vi "BRig_RT_start_v1,12__PortC.vi"() -> ()   [LabVIEW 2014]
uses:
  myRIO_BRig_RT__Case_Exp_stateList.ctl
  myRIO_BRig_RT__Case_NonExp_stateList.ctl
  <vilib>/WebDAVClient/Advanced/SessionHandle.ctl
  <vilib>/Platform/TimedLoop/XDataNode/timing_clust.ctl
  <vilib>/Platform/TimedLoop/XDataNode/nitl_modes.ctl
  <vilib>/Platform/TimedLoop/XDataNode/wakeup.ctl
  <vilib>/myRIO/Common/Instrument Driver Framework/myRIO v1.0/UART/vis/myRIO v1.0 Close UART.vi
  <vilib>/FPGAPlugInAG/myRIO-1900/niLvFpga_Open_myRIO-1900.vi
  <vilib>/rvi/interface/common/dynamic/niFpgaDynamicAddResources.vi
  <vilib>/Utility/error.llb/Error Cluster From Error Code.vi
  <vilib>/rvi/errors/niLvFpgaAdjustHostInterfaceError.vi
  <vilib>/Utility/file.llb/Read From Spreadsheet File (I64).vi
  <vilib>/Utility/file.llb/Write To Spreadsheet File (DBL).vi
  <vilib>/FPGAPlugInAG/Dynamic/niLvFpga_Close_Dynamic.vi
  <vilib>/myRIO/Common/Instrument Driver Framework/Utilities/vis/FPGA Ref Manager.vi
  <vilib>/myRIO/Common/Instrument Driver Framework/myRIO v1.0/myRIO v1.0 Reset FPGA.vi
  <vilib>/myRIO/Common/Instrument Driver Framework/myRIO v1.0/IRQ/vis/myRIO v1.0 IRQ Info FGV.vi
  <vilib>/myRIO/Common/Instrument Driver Framework/myRIO v1.0/IRQ/vis/myRIO v1.0 Timer IRQ Info FGV.vi
  <vilib>/myRIO/Common/Instrument Driver Framework/myRIO v1.0/IRQ/vis/myRIO v1.0 ISR Agent.vi
  <vilib>/rvi/interface/nirviOpenFPGA/nirviOpenFPGA.xnode
  BRig_FPGA_v3,93__PortC__build.lvbitx
  BRig_FPGA_v3,93__PortC.vi
  <vilib>/rvi/interface/nirviReadWriteControl/nirviReadWriteControl.xnode
  <vilib>/Platform/TimedLoop/XDataNode/XDataNode.xnode
  <vilib>/rvi/interface/nirviCloseFPGA/nirviCloseFPGA.xnode
  <vilib>/Platform/TimedLoop/XDataNode/XDNodeRunTimeDep.lvlib
  <vilib>/rvi/interface/Simulation/niFpgaSimulationCallBeginRW.vi
  <vilib>/myRIO/Instrument Drivers/Utilities/Utilities.lvlib
  NiFpgaLv.dll
  <vilib>/WebDAVClient/NI_WebDAV.lvlib
panel:
  out "Solenoid R":bool
  out "Solenoid L":bool
  out "Laser2":bool
  out "Laser1":bool
  out "FreeReward_c_R":u16
  out "FreeReward_c_L":u16
  in  "Laser2_LED":bool
  in  "Laser1_LED":bool
  in  "lick_Rising(F)_or_Falling(T)":bool
  out "T_ExpRun_min":dbl
  out "stop_TimedLoop":bool
  out "BTPR_avg_R":dbl
  out "T2R_avg_R":dbl
  out "BTPR_avg_L":dbl
  out "T2R_avg_L":dbl
  out "BTPR_block":u16
  out "T2R_block":u16
  in  "comm_WebDAV_connect":bool
  in  "I_sendData":bool
  in  "comm_TCP_connect":bool
  out "nRewards_total":u16 caption="# Rewards in Current Block"
  out "BUR_target":u16 caption="Target Trials Per Block"
  in  "input_Threshold_reset":bool
  out "nTrial":u16
  out "allReward_R":bool
  out "allReward_L":bool
  out "Threshold":bool
  out "tLoop":dbl format="%#_2g"
  out "L_Power_l2":dbl
  out "comm_TCP":bool
  in  "get_countPerMS":bool
  out "SolenoidReward":bool
  out "L_Power_l1":dbl caption="LaserPower"
  in  "Recording":bool
  out "FPGA_count2ms":dbl=159.0
  out "error out":errorcluster
  out "cSpout":enum16{"Left", "Right"}(ring) caption="Left or Right Spout"
  out "A4":u32 caption="LickCounter_Right"
  out "A2":u32 caption="LickCounter_Left"
  out "nRewards_Right":u16 caption="# Rewards Total (Right)"
  out "nRewards_Left":u16 caption="# Rewards Total (Left)"
  out "nRewards_cur":u16 caption="# Rewards in Current Block"
  out "TpB_target":u16 caption="Target Trials Per Block"
  out "cState_NonExp":T1 caption="WarmUp State"
  out "iBlock":u16 caption="Current Block"
  out "cState":T2 caption="Experimental State"
  out "iTrial":u16 caption="Current Trial"
  in  "Data Set Prefix":string="Exp1_TM2"
  out "comm_WebDAV":bool
  in  "Host Password":string="sabalab"
  in  "Host UserName":string="Test2"
  in  "STOP_abort":bool caption="Stop LabView\n(Stops myRio and FPGA)"
  in  "STOP_endBlock":bool caption="Stop Experiment\n@ End of Block"
  in  "STOP_endTrial":bool caption="Stop Experiment\n@ End of Trial"
  in  "START":bool caption="Start Experiment"
  # "Experimental Run"
  # "Recording Rig"
  # "FPGA Conversion\n[counts per ms]"
  # "RealTime Cycle\nShould be <5ms"
  # "STOP experiment at"
  # "Exp Run Time"
  # "Reset"
  # "min"
  # "Communication with Host"
  # "Lick Counter"
  # "Give Water?\n(Reward)"
  # "Experimental State"
  # "Left/Right"
  # "Left           Right"
  # "Direction\n(NonSpecific Licking)"
  # "Block Target"
  # "# Blocks"
  # "L          R"
  # "# Trials"
  # "# Rewards"
  # "Bad Trials\nPost Reward"
  # "Trials 2 Reward"
  # "Block"
  # "# Trials"
  # "# Rewards"
  # "Current\nBlock"
  # "WarmUp State"
  # "avg L"
  # "Total"
  # "# Rewards"
  # "# Trials"
  # "avg R"
  # "Laser Power [V]"
  # "Left           Right"
  # "FreeRewards"
  # "Laser1"
  # "Laser2"
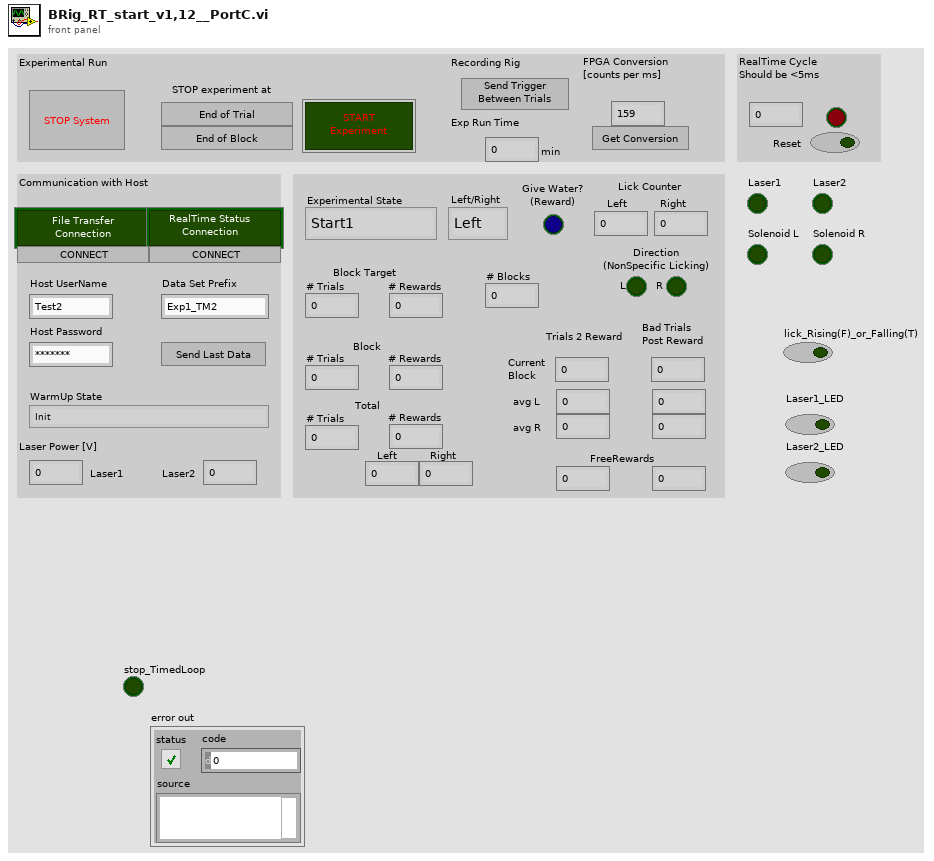
[diagram p1: front panel]
types:
  T1 = typedef "myRIO_BRig_RT__Case_NonExp_stateList.ctl" = enum16{"Init", "UploadSettings_pre", "UploadSettings_Read_dataExp", "UploadSettings_dataExp_1", "UploadSettings_dataExp_2", "UploadSettings_Read_dataLC", "UploadSettings_dataLC_1", "UploadSettings_dataLC_2", "UploadSettings_dataLC_3", "UploadSettings_dataLC_4", "UploadSettings_Read_dataMTrig", "UploadSettings_dataMTrig_1", "UploadSettings_post", "Idle_pre", "IdleEmpty", "IdleEmpty2", "IdleEmpty3", "IdleEmpty4", "Idle", "Idle_2", "Idle_3", "Idle_4", "Idle_5", "Idle_6", "Idle_post", "Cue_pre__pre", "Cue_pre", "Cue", "Cue_LED", "Cue_post", "RewardCalibration_pre", "RewardCalibration", "DispenseWater_pre__pre", "DispenseWater_pre", "DispenseWater", "DispenseWater_post", "TestConnection", "SendData", "Get_FPGA_count_per_ms", "End", "commTCP_connect"}
  T2 = typedef "myRIO_BRig_RT__Case_Exp_stateList.ctl" = enum16{"Start1", "Start2", "Start3", "saveSettings1", "saveSettings2", "saveSettings3", "saveSettings4", "saveSettings_LC_ENL_l1", "saveSettings_LC_ENL_l2", "saveSettings_LC_Cue_l1", "saveSettings_LC_Cue_l2", "saveSettings6_LC_l1_Other", "SaveSettings6_LC_l2_Other", "setSettings_Audio", "setSettings_Laser", "initBlock_pre", "initBlock", "initBlock2", "initBlock_post", "initTrial_pre", "initTrial", "initTrial2", "initTrial3", "initTrial4", "initTrial_LC_ENL1", "initTrial_LC_Cue1", "initTrial_LC_Cue1_2", "initTrial_LC_Sel", "initTrial_post", "ENL1_pre", "ENL1", "ENL1_post", "ENL1Penalty_pre", "ENL1Penalty", "ENL2_pre", "ENL2", "ENL2Penalty_pre", "ENL2Penalty", "Cue1_pre", "Cue1", "Cue1_post", "Cue1Penalty_pre", "Cue1Penalty", "Cue2_pre", "Cue2", "Cue2Penalty_pre", "Cue2Penalty", "Selection_pre", "Selection", "Select_post", "SelectReward_pre", "SelectReward", "SelectRewardPost_pre", "SelectRewardPost", "SelectWrong_pre", "SelectWrong", "SelectWrong_post", "SelectTimeout_pre", "SelectTimeout", "SelectTimeout_post", "endTrial_pre", "endTrial1", "endTrial2", "endTrial3", "endTrial_post", "endBlock_pre", "endBlock", "endBlock_post", "endExp", "commConnect", "commUpload_pre", "commUpload_dataBlock", "commUpload_dataCurrent", "commUpload_dataExp", "commUpload_dataLC", "commUpload_dataTrial", "commUpload_post", "saveData_pre", "saveData_dataBlock", "saveData_dataCurrent", "saveData_dataExp", "saveData_dataLC", "saveData_dataTrial", "saveData_post", "empty_endBlock1", "empty_endBlock2", "empty_endTrial1", "empty_endTrial2", "empty_endTrial3", "empty_endTrial4", "empty_endTrial5", "dummyState", "dummyState_endBlock", "FreeReward_pre", "FreeReward", "FreeRewardPost_pre", "FreeRewardPost"}
  T3 = enum8{"Enabled", "Disabled", "Disabled and Grayed Out"}
  T4 = typedef "NI_WebDAV.lvlib/SessionHandle.ctl" = refnum<k1>
  T5 = typedef "XDNodeRunTimeDep.lvlib/timing_clust.ctl" = cluster{"Expected End [f-1]":u64, "Actual End [f-1]":u64, "Finished Late? [f-1]":bool, "Expected End [i-1]":u64, "Actual End [i-1]":u64, "Finished Late? [i-1]":bool, "Expected Start [i]":u64, "Actual Start [i]":u64, "Expected Start [f]":u64, "Actual Start [f]":u64, "Source Name":string, "Structure Name":string, "Period":i64, "Deadline":i64, "Offset":i64, "Start":i64, "Priority":i32, "Timeout":i32, "Mode":T6, "Wakeup Reason":T7, "Error":errorcluster, "Source Type":string, "Secondary Source Type":string, "Global End Time":u64, "Global Start Time":u64, "Frame Duration":u64, "Iteration Duration":u64, "Assigned CPU":i32, "I/O Scan Engine Mode":u32}
  T6 = typedef "XDNodeRunTimeDep.lvlib/nitl_modes.ctl" = enum32{"No Change", "Process missed periods, maintain original phase", "Discard missed periods, maintain original phase", "Process missed periods, ignore original phase", "Discard missed periods, ignore original phase"}
  T7 = typedef "XDNodeRunTimeDep.lvlib/wakeup.ctl" = enum32{"Normal", "Aborted", "Asynchronous wakeup", "Timing source error", "Timed loop error", "Timeout"}
  T8 = cluster{"read mode":enum16{"polling", "blocking"}, "write mode":enum16{"polling", "blocking"}}
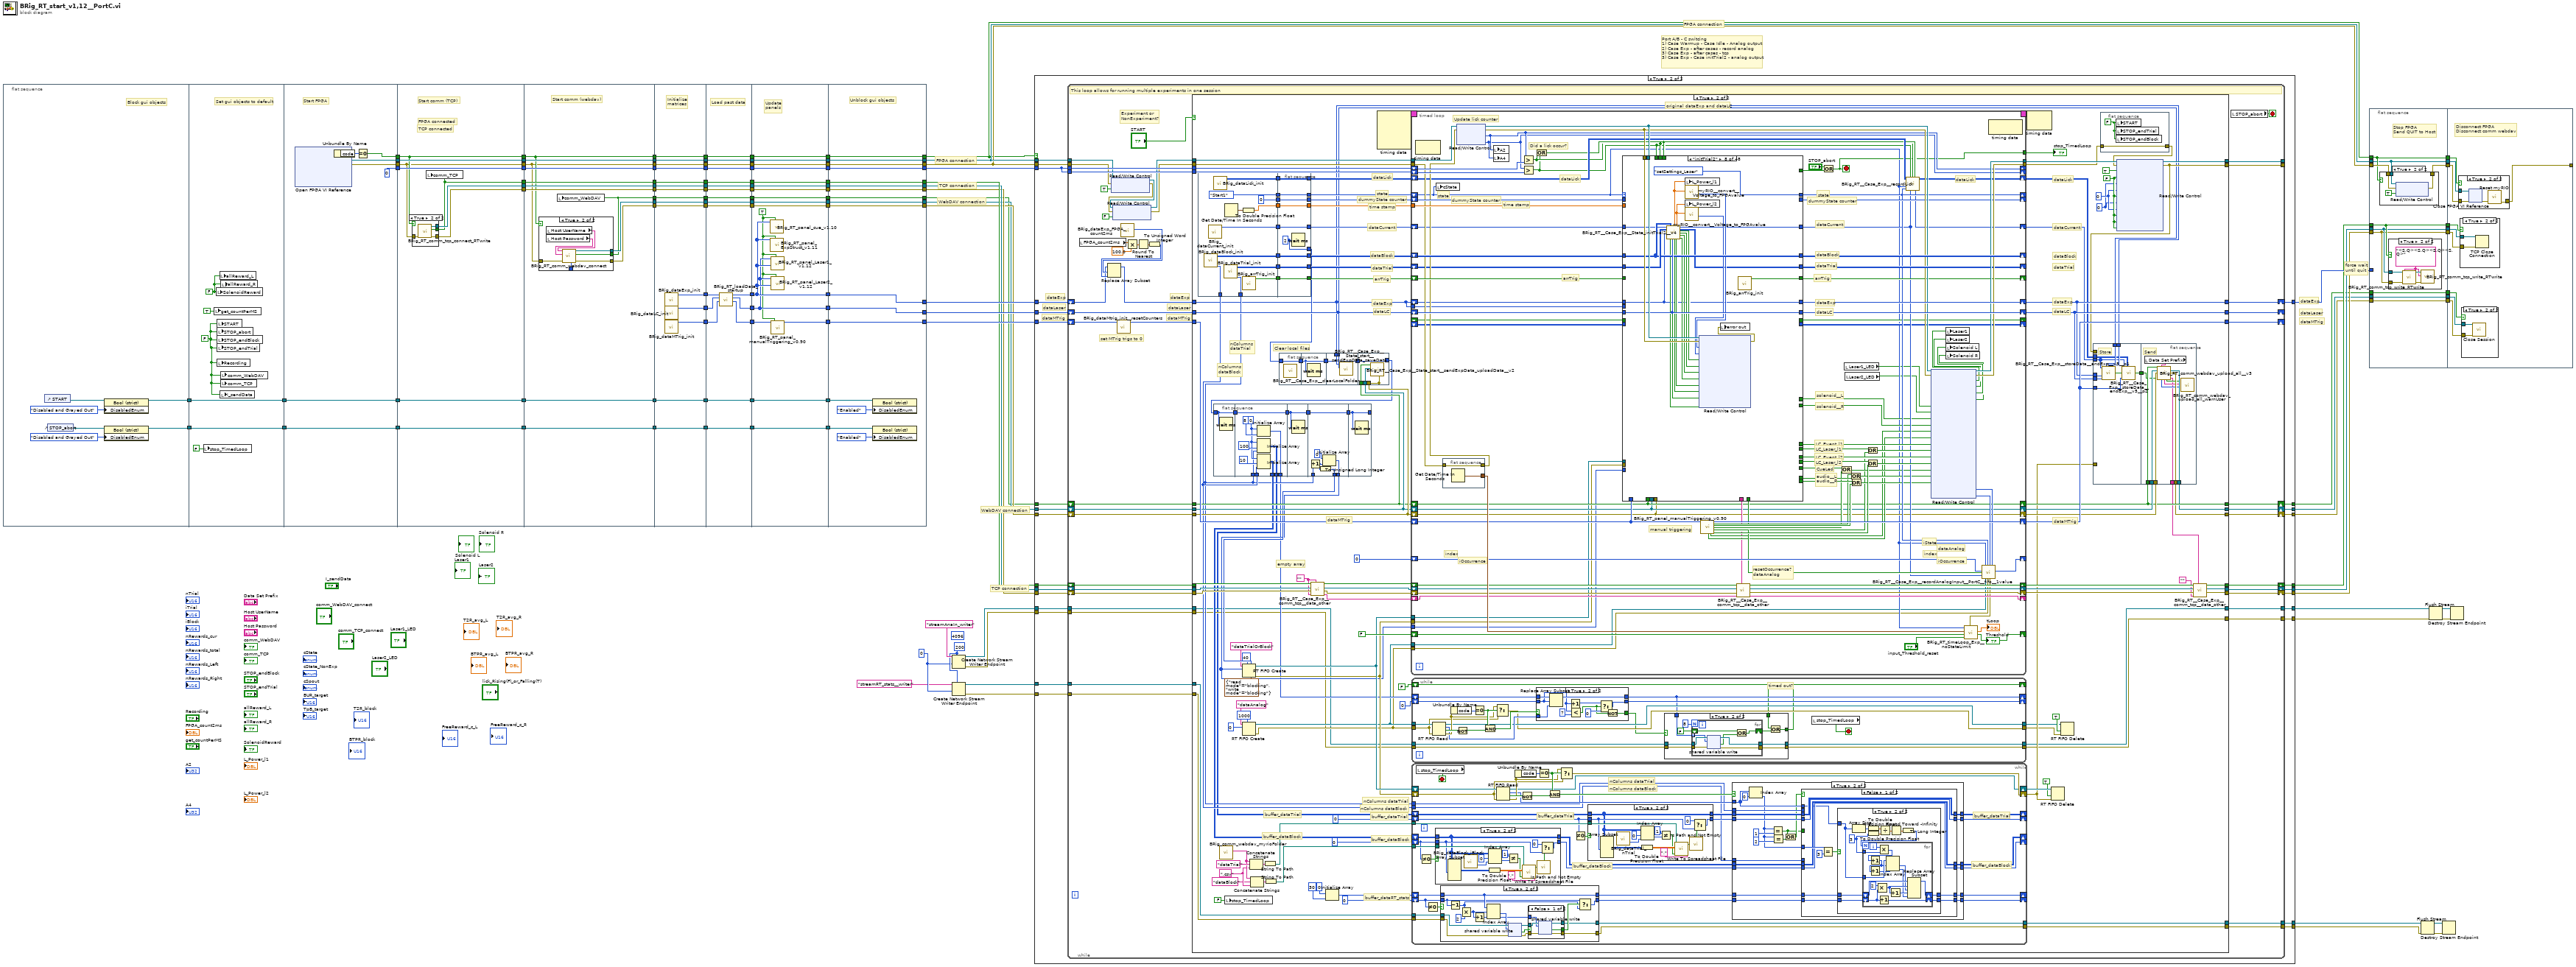
[diagram p0: block diagram]
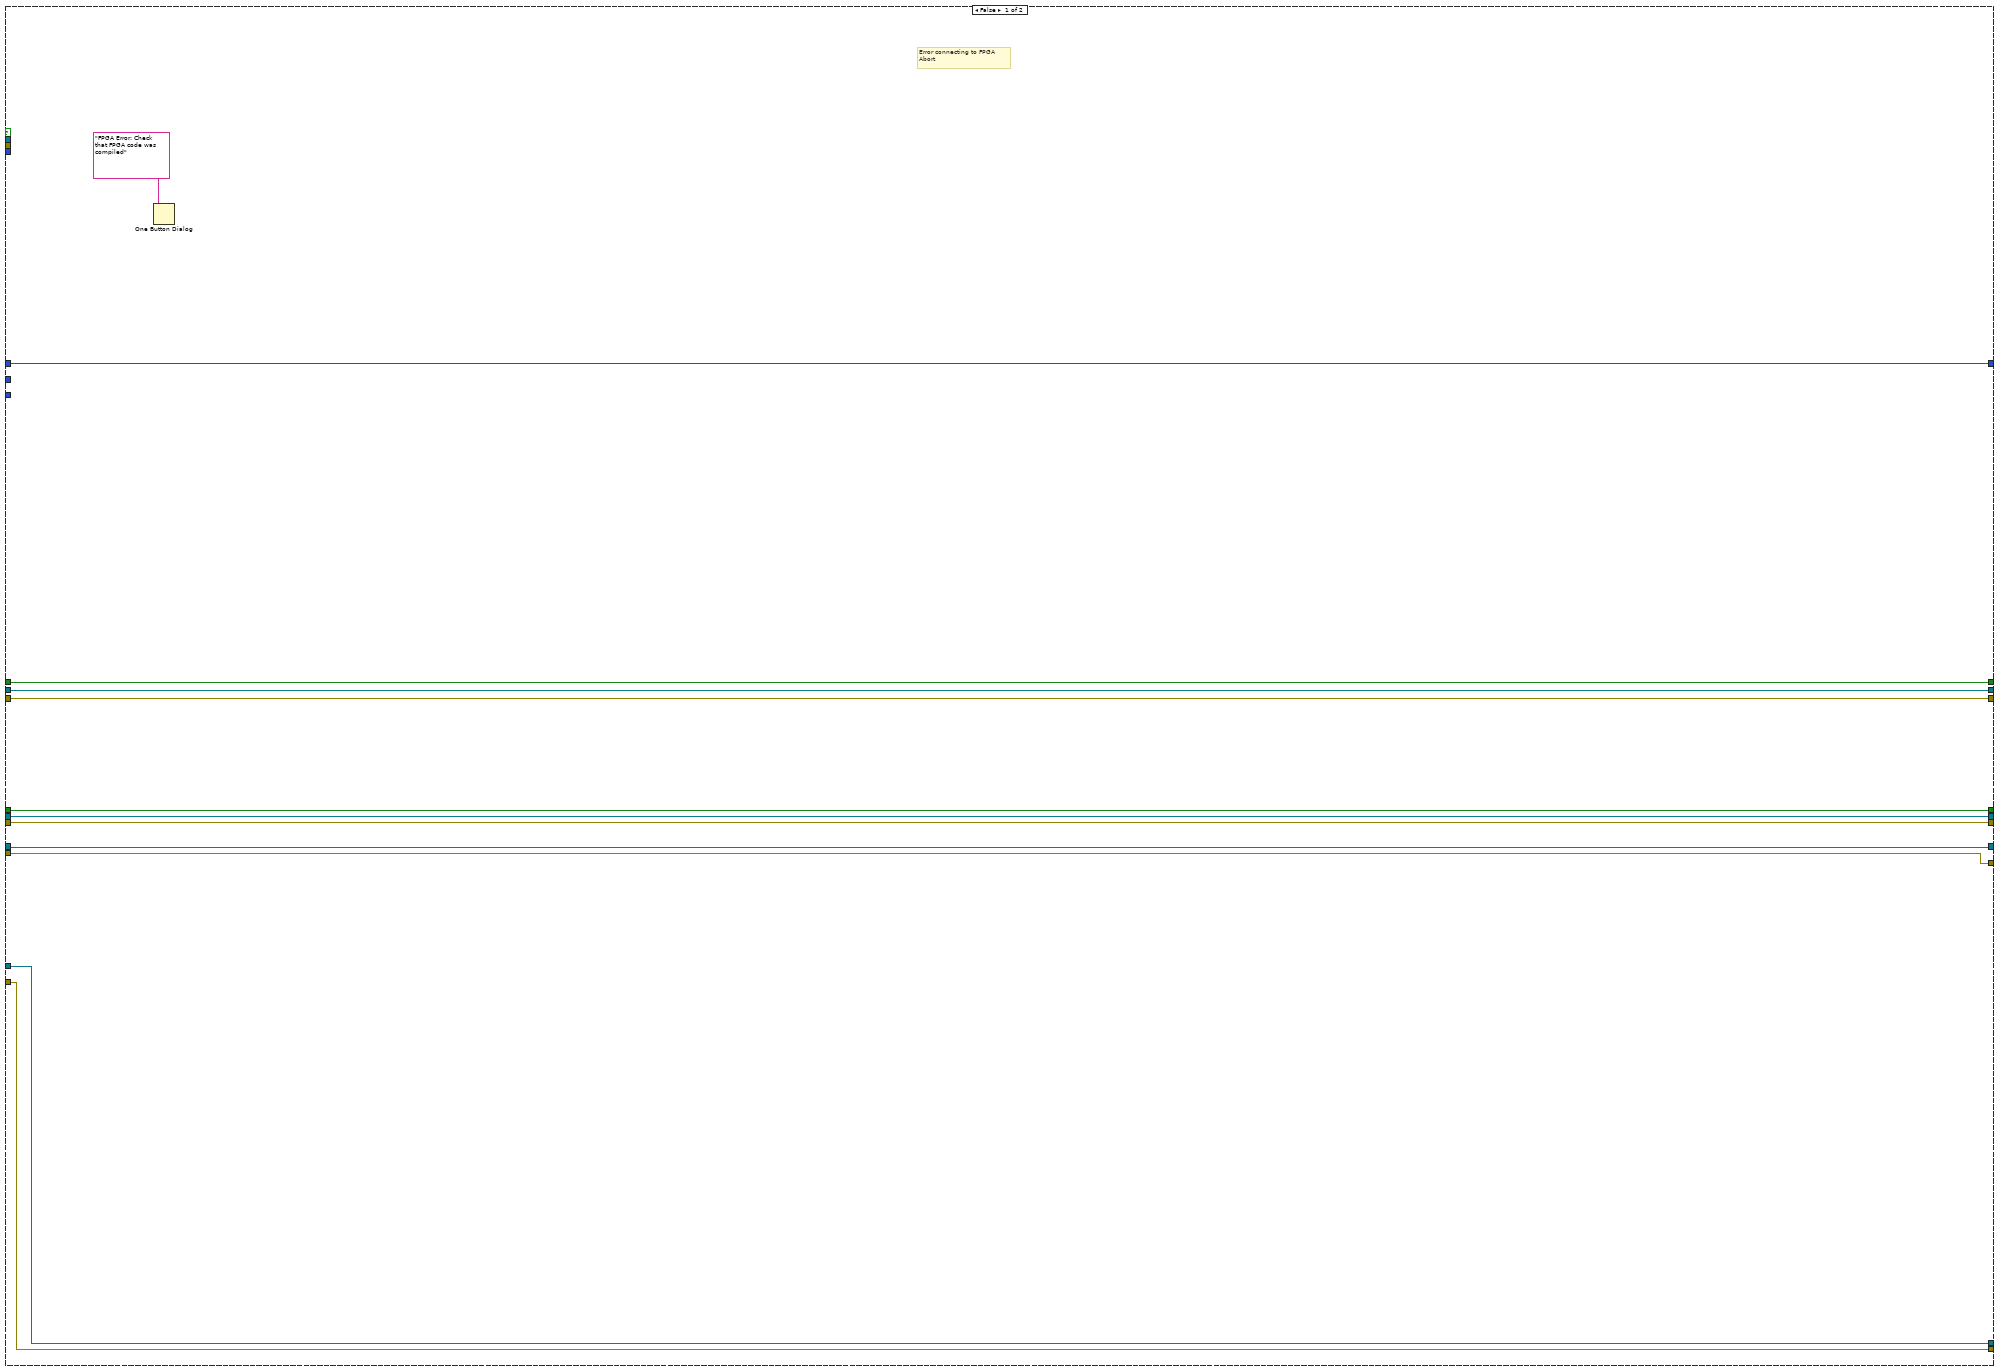
[diagram p2: hidden frame]
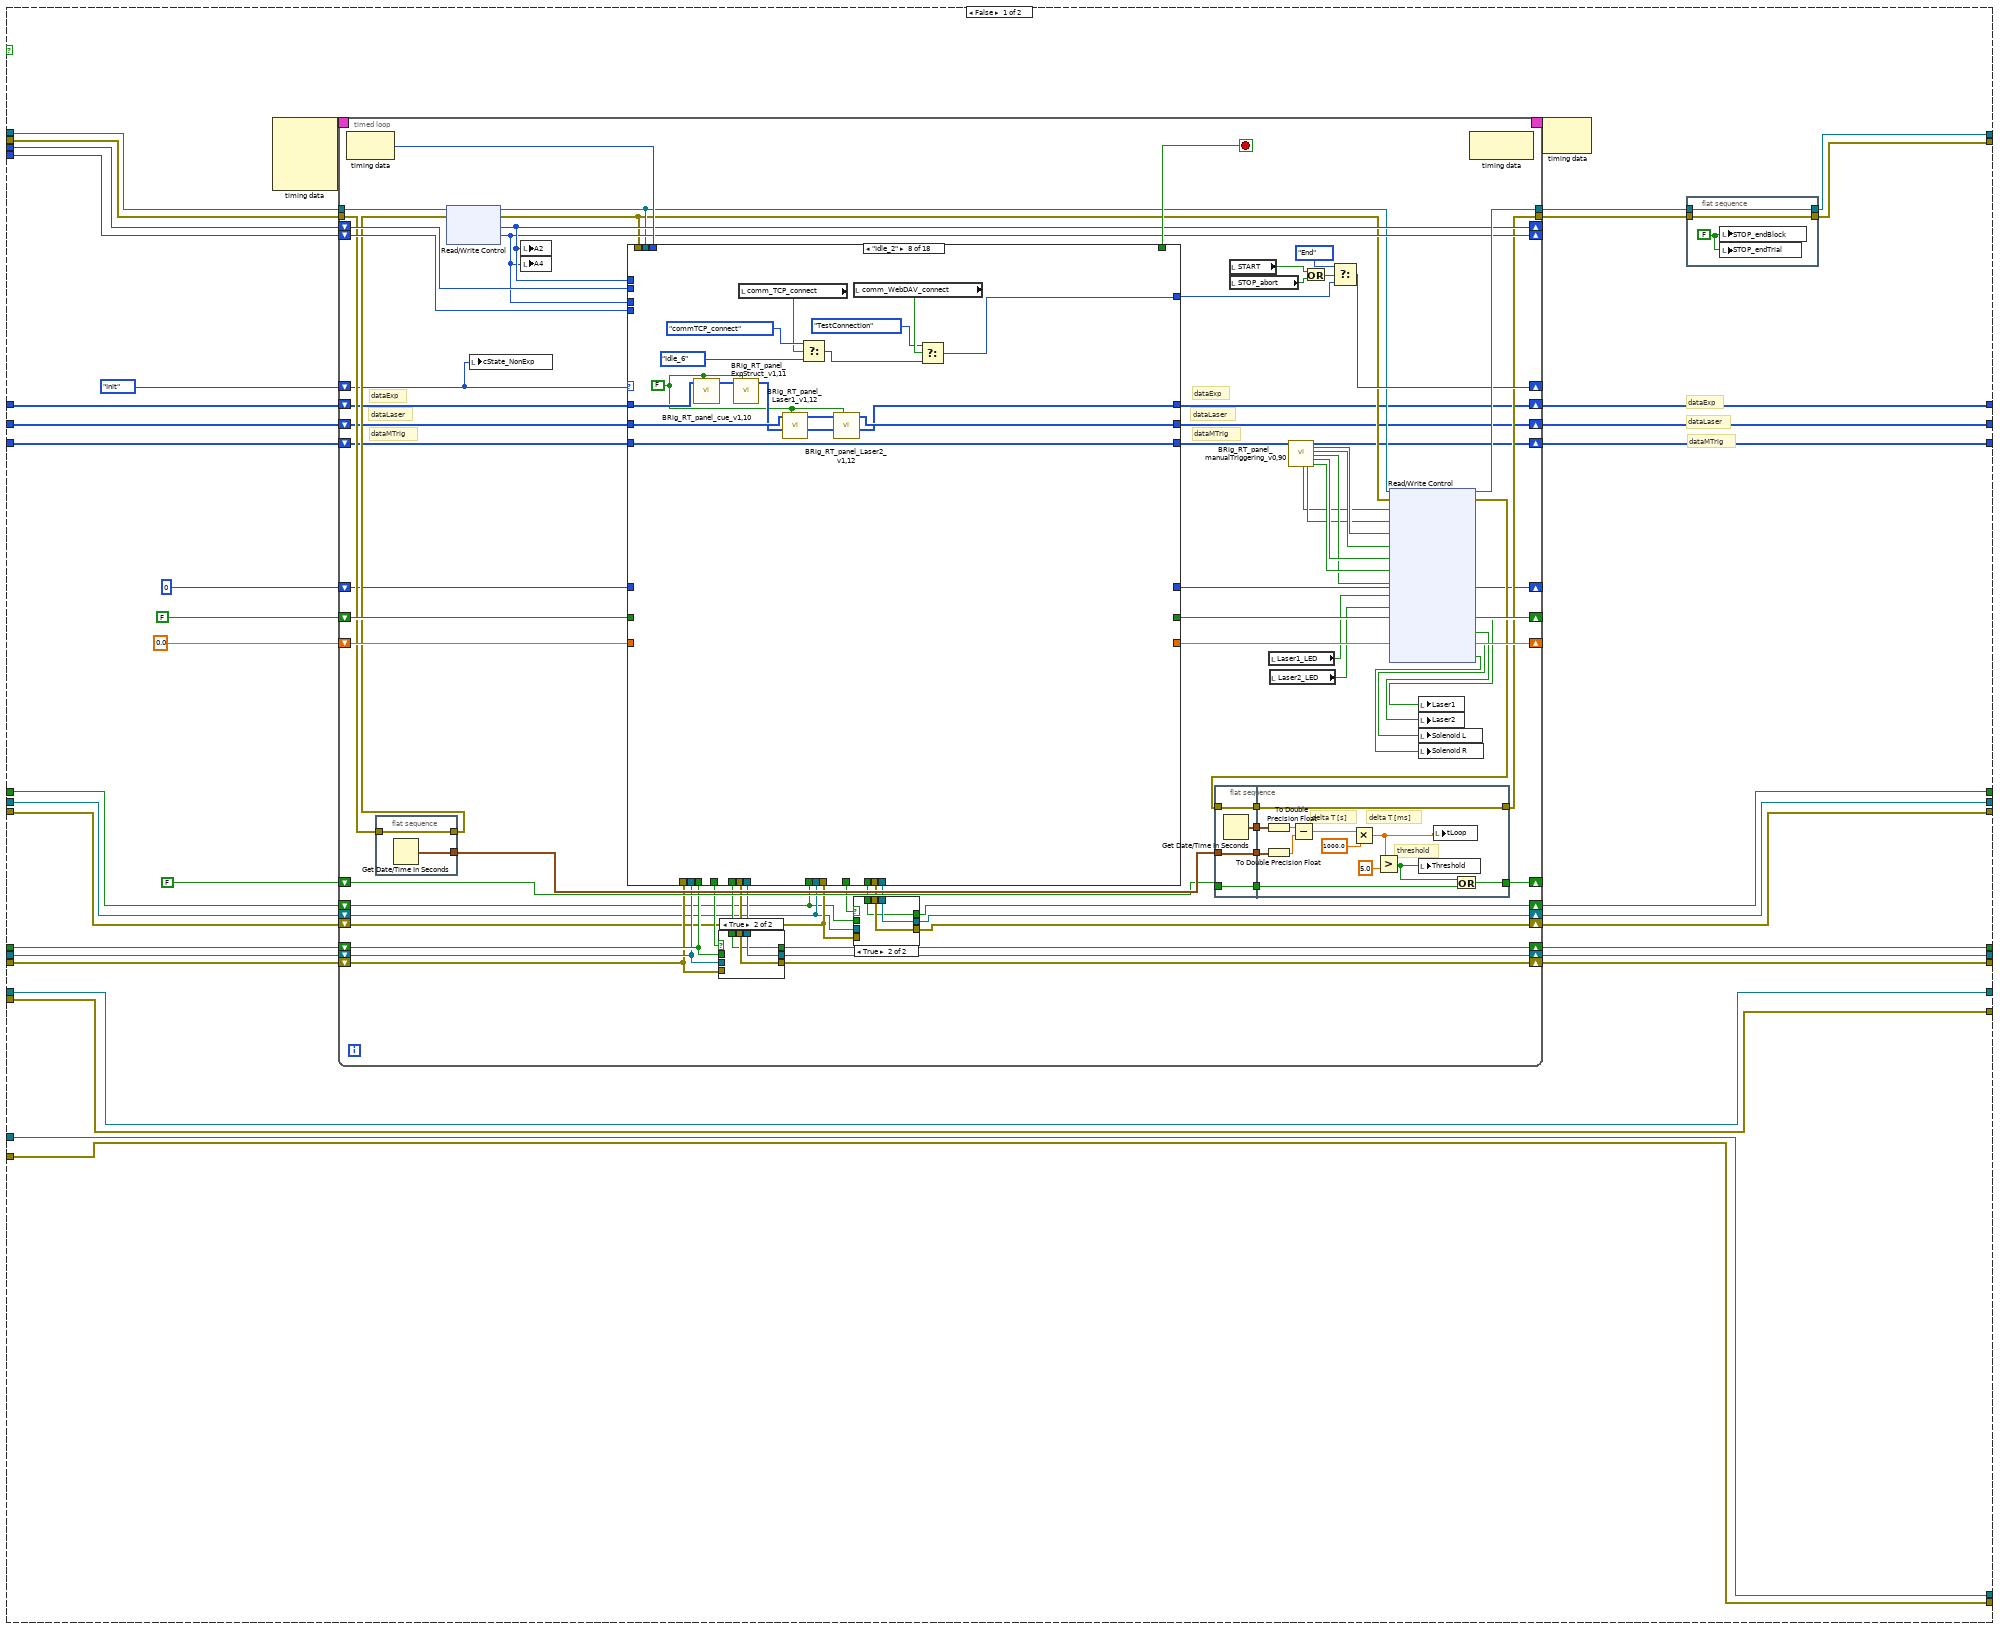
[diagram p3: hidden frame]
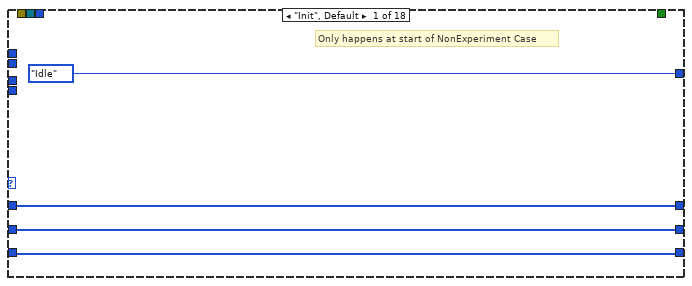
[diagram p6: hidden frame]
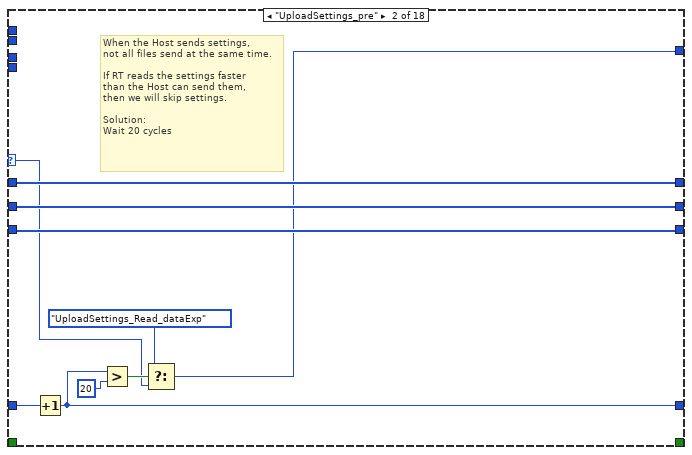
[diagram p7: hidden frame]
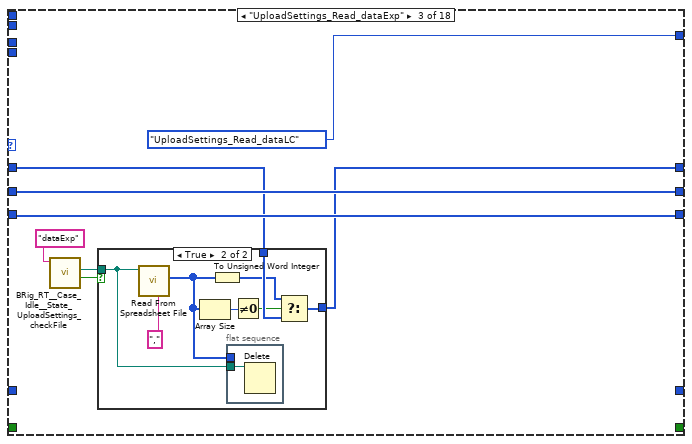
[diagram p8: hidden frame]
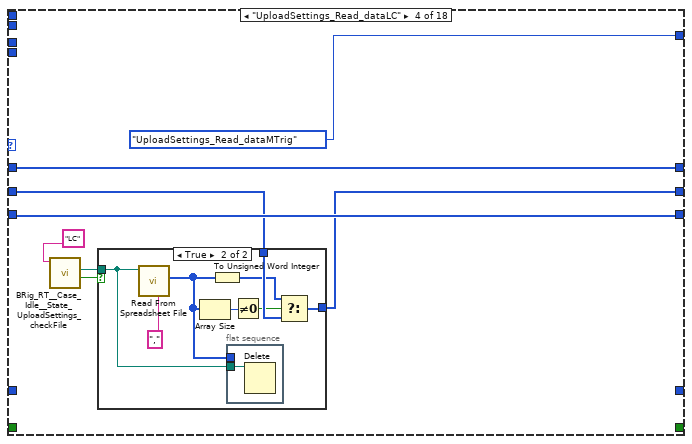
[diagram p10: hidden frame]
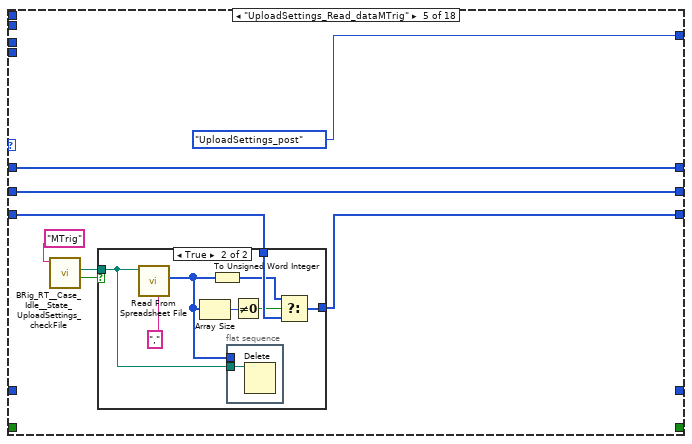
[diagram p12: hidden frame]
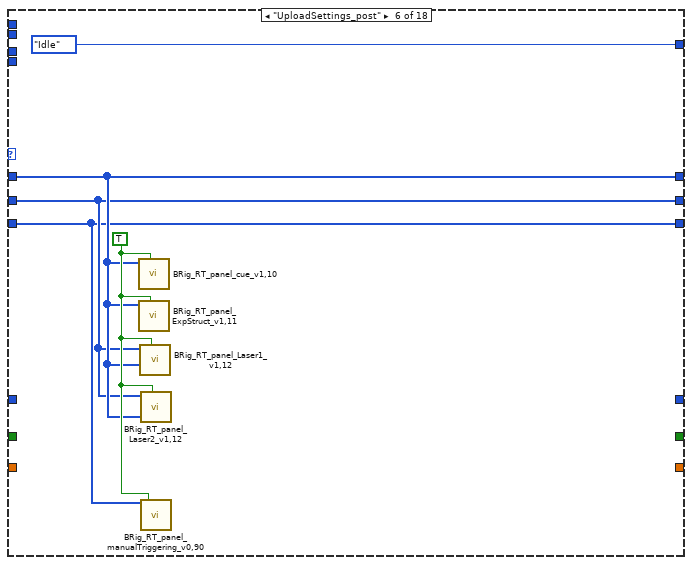
[diagram p14: hidden frame]
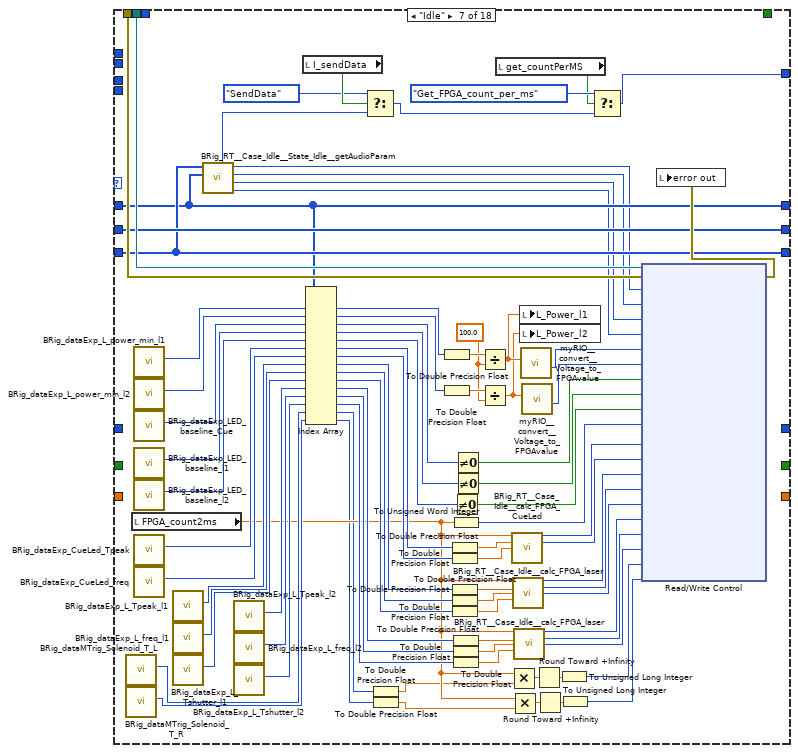
[diagram p15: hidden frame]
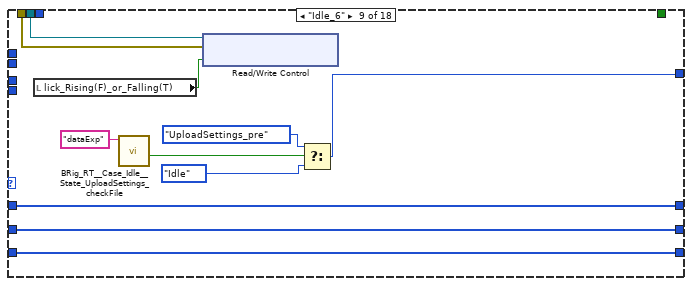
[diagram p16: hidden frame]
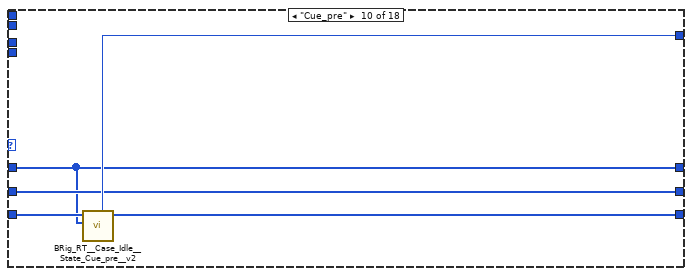
[diagram p17: hidden frame]
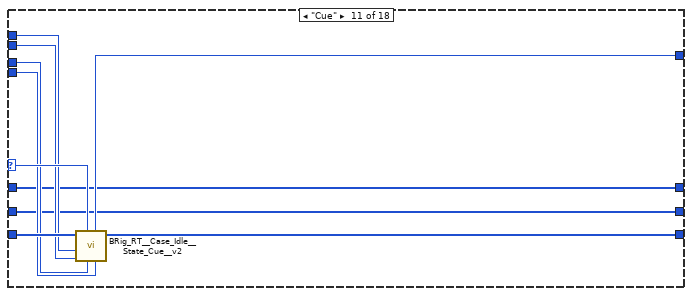
[diagram p18: hidden frame]
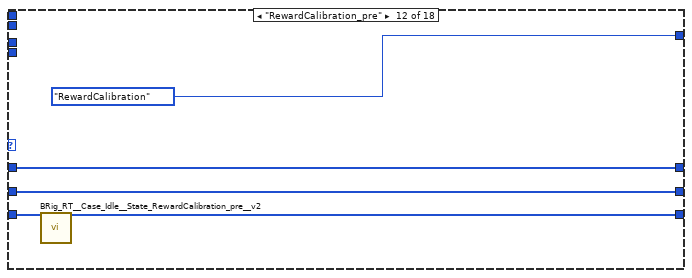
[diagram p19: hidden frame]
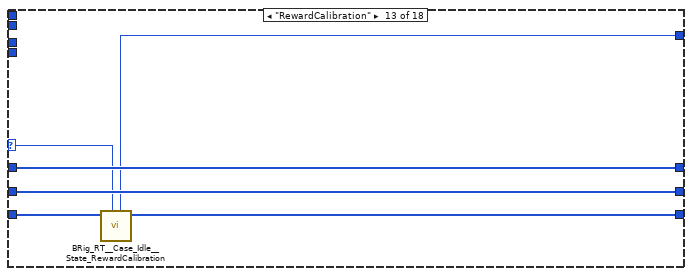
[diagram p20: hidden frame]
diagram:
  w8 = u16 0 ("element")
  (unwired) 4096 ("reader buffer size")
  w9 = 200 ("reader buffer size")
  # "WebDAV connection"
  # "TCP connection"
  # "WebDAV connection"
  # "TCP connection"
  # "FPGA connection"
  # "FPGA connection"
  # "Port A/B - C switcing\n1) Case Warmup - Case Idle - Analog output\n2) Case Exp - after cases - record analog\n3) Case Exp - after cases - tcp\n3) Case Exp - Case initTrial2 - analog output"
  # "force wait\nuntil quit"
  # "dataLaser"
  # "dataExp"
  # "dataMTrig"
  n1 = flat-sequence {
    tunnel: [w123] -> w106
    tunnel: [w122] -> w102
    tunnel: [w132] -> w107
    tunnel: w106 -> [w132]
    tunnel: [w131] -> w103
    tunnel: w102 -> [w131]
    tunnel: [w138] -> w120
    tunnel: [w140] -> w119
    tunnel: [u32 0] -> w118
    tunnel: [w136] -> w117
    tunnel: [w135] -> w108
    tunnel: w107 -> [w135]
    tunnel: [w134] -> w104
    tunnel: w103 -> [w134]
    tunnel: w120 -> [w146]
    tunnel: w119 -> [w149]
    tunnel: w118 -> [w148]
    tunnel: w117 -> [w147]
    tunnel: [w146] -> w116
    tunnel: [w149] -> w115
    tunnel: [w148] -> w114
    tunnel: [w147] -> w113
    tunnel: [w141] -> w112
    tunnel: [w145] -> w111
    tunnel: [w144] -> w110
    tunnel: [w143] -> w109
    tunnel: w108 -> [w143]
    tunnel: [w142] -> w105
    tunnel: w104 -> [w142]
    tunnel: w116 -> [w160]
    tunnel: w115 -> [w168]
    tunnel: w114 -> [w167]
    tunnel: w113 -> [w161]
    tunnel: w112 -> [w166]
    tunnel: w111 -> [w165]
    tunnel: w110 -> [w164]
    tunnel: [w160] -> w73
    tunnel: [w168] -> w72
    tunnel: [w167] -> w71
    tunnel: [w161] -> w70
    tunnel: [w166] -> w69
    tunnel: [w165] -> w68
    tunnel: [w164] -> w67
    tunnel: [w163] -> w66
    tunnel: w109 -> [w163]
    tunnel: [w162] -> w65
    tunnel: w105 -> [w162]
    tunnel: [w159] -> w64
    tunnel: [w157] -> w63
    tunnel: [w158] -> w62
    tunnel: w73 -> [w193]
    tunnel: [w193] -> w61
    tunnel: w72 -> [w192]
    tunnel: [w192] -> w60
    tunnel: w71 -> [w191]
    tunnel: [w191] -> w59
    tunnel: w70 -> [w190]
    tunnel: [w190] -> w58
    tunnel: w69 -> [w189]
    tunnel: [w189] -> w57
    tunnel: w68 -> [w188]
    tunnel: [w188] -> w56
    tunnel: w67 -> [w187]
    tunnel: [w187] -> w55
    tunnel: w66 -> [w186]
    tunnel: [w186] -> w54
    tunnel: w65 -> [w185]
    tunnel: [w185] -> w53
    tunnel: w64 -> [w184]
    tunnel: [w184] -> w52
    tunnel: w63 -> [w183]
    tunnel: [w183] -> w51
    tunnel: w62 -> [w182]
    tunnel: [w182] -> w50
    tunnel: [w181] -> w49
    tunnel: [w180] -> w48
    tunnel: [w179] -> w47
    tunnel: w61 -> [w211]
    tunnel: [w211] -> w46
    tunnel: w60 -> [w210]
    tunnel: [w210] -> w44
    tunnel: w59 -> [w209]
    tunnel: [w209] -> w42
    tunnel: w58 -> [w208]
    tunnel: [w208] -> w40
    tunnel: w57 -> [w207]
    tunnel: [w207] -> w38
    tunnel: w56 -> [w206]
    tunnel: [w206] -> w36
    tunnel: w55 -> [w205]
    tunnel: [w205] -> w34
    tunnel: w54 -> [w204]
    tunnel: [w204] -> w32
    tunnel: w53 -> [w203]
    tunnel: [w203] -> w30
    tunnel: w52 -> [w202]
    tunnel: [w202] -> w28
    tunnel: w51 -> [w201]
    tunnel: [w201] -> w26
    tunnel: w50 -> [w200]
    tunnel: [w200] -> w24
    tunnel: w49 -> [w195]
    tunnel: [w194] -> w22
    tunnel: w48 -> [w197]
    tunnel: [w196] -> w20
    tunnel: w47 -> [w199]
    tunnel: [w198] -> w19
    tunnel: w46 -> [w228]
    tunnel: [w228] -> w45
    tunnel: w44 -> [w227]
    tunnel: [w227] -> w43
    tunnel: w42 -> [w226]
    tunnel: [w226] -> w41
    tunnel: w40 -> [w225]
    tunnel: [w225] -> w39
    tunnel: w38 -> [w224]
    tunnel: [w224] -> w37
    tunnel: w36 -> [w223]
    tunnel: [w223] -> w35
    tunnel: w34 -> [w222]
    tunnel: [w222] -> w33
    tunnel: w32 -> [w221]
    tunnel: [w221] -> w31
    tunnel: w30 -> [w220]
    tunnel: [w220] -> w29
    tunnel: w28 -> [w219]
    tunnel: [w219] -> w27
    tunnel: w26 -> [w218]
    tunnel: [w218] -> w25
    tunnel: w24 -> [w217]
    tunnel: [w217] -> w23
    tunnel: w22 -> [w214]
    tunnel: [w213] -> w21
    tunnel: w20 -> [w215]
    tunnel: w19 -> [w216]
    tunnel: [w216] -> w18
    tunnel: [w215] -> w17
    tunnel: [w235] -> w83
    tunnel: [w236] -> w84
    tunnel: [w237] -> w85
    tunnel: [w242] -> w89
    tunnel: [w243] -> w121
    tunnel: [w244] -> w96
    tunnel: [w245] -> w95
    tunnel: w45 -> [w245]
    tunnel: w43 -> [w244]
    tunnel: w41 -> [w243]
    tunnel: w39 -> [w242]
    tunnel: w37 -> [w237]
    tunnel: w35 -> [w236]
    tunnel: w33 -> [w235]
    tunnel: w31 -> [w239]
    tunnel: w29 -> [w238]
    tunnel: w27 -> [w233]
    tunnel: w25 -> [w234]
    tunnel: w23 -> [w232]
    tunnel: [w234] -> w77
    tunnel: [w233] -> w78
    tunnel: [w232] -> w79
    tunnel: [w229] -> w92
    tunnel: [w230] -> w91
    tunnel: [w231] -> w90
    tunnel: w21 -> [w231]
    tunnel: w18 -> [w229]
    tunnel: w17 -> [w230]
    frame #0 {
      # "Block gui objects"
      n2 = control-ref of="START"() -> (w127:refnum<vi>)
      n3 = control-ref of="STOP_abort"() -> (w124:refnum<vi>)
      n4 = property class="Bool (strict)"(reference=w127, "DisabledEnum"=T3."Disabled and Grayed Out" ("Disabled")) -> (reference out=w123:refnum<vi>)  [unwired: 1 in, 1 out]
      n5 = property class="Bool (strict)"(reference=w124, "DisabledEnum"=T3."Disabled and Grayed Out" ("Disabled")) -> (reference out=w122:refnum<vi>)  [unwired: 1 in, 1 out]
    }
    frame #1 {
      w129 = FALSE ("SolenoidReward")
      w130 = FALSE
      # "Set gui objects to default"
      n6 = local write "stop_TimedLoop"(FALSE ("stop_TimedLoop")) -> ()
      n7 = local write "get_countPerMS"(TRUE ("get_countPerMS")) -> ()
      n8 = local write "SolenoidReward"(w129) -> ()
      n9 = local write "START"(w130) -> ()
      n10 = local write "STOP_abort"(w130) -> ()
      n11 = local write "STOP_endBlock"(w130) -> ()
      n12 = local write "STOP_endTrial"(w130) -> ()
      n13 = local write "Recording"(w130) -> ()
      n14 = local write "allReward_L"(w129) -> ()
      n15 = local write "I_sendData"(w130) -> ()
      n16 = local write "comm_WebDAV"(w130) -> ()
      n17 = local write "comm_TCP"(w130) -> ()
      n18 = local write "allReward_R"(w129) -> ()
    }
    frame #2 {
      # "Start FPGA"
      n19 = xnode "Open FPGA VI Reference"() -> ("FPGA VI Reference Out"=w140:refnum<k20>, "error out"=w138:errorcluster)  [unwired: 2 in]
      n20 = Unbundle By Name(w138) -> ("code"=w137:i32)
      n21 = Equal To 0?(x=w137) -> (x = 0?=w136:bool)
    }
    frame #3 {
      # "TCP connected"
      # "Start comm (TCP)"
      # "FPGA connected"
      n22 = case shown="True" w147 {
        selector: w147 -> [w150 _]
        tunnel: w146 -> [w152 w156]
        tunnel: [refnum<k5> refnum ("output_hTCP") w155] -> w145
        tunnel: [w150 w154] -> w141
        tunnel: [w152 w153] -> w144
        frame False {
        }
        frame True {
          n23 = call "BRig_RT_comm_tcp_connect_RTwrite.vi"("input_error"=w156) -> ("output_error"=w153:errorcluster, "output_connected"=w154:bool, "output_hTCP"=w155:refnum<k5>)  [unwired: 8 in]
        }
      }
      n24 = local write "comm_TCP"(w141) -> ()
    }
    frame #4 {
      # "Start comm (webdav)"
      n25 = case shown="True" w161 {
        selector: w161 -> [w170 _]
        tunnel: [w169 w176] -> w159
        tunnel: [w170 w175] -> w157
        tunnel: w160 -> [w171 w174]
        tunnel: [w171 w173] -> w158
        tunnel: [_ w172] -> _
        frame False {
          w169 = T4 refnum items=["Session NI_WebDAV"] ("output_hSession")
        }
        frame True {
          n26 = local read "Host UserName"() -> (w177:string)
          n27 = local read "Host Password"() -> (w178:string)
          n28 = call "BRig_RT_comm_webdav_connect.vi"("input_error"=w174, "input_password"=w178, "input_username"=w177) -> ("output_error"=w173:errorcluster, "output_Iconnected"=w175:bool, "output_hSession"=w176:T4, "output_code"=w172:u8)  [unwired: 5 in]
        }
      }
      n29 = local write "comm_WebDAV"(w157) -> ()
    }
    frame #5 {
      # "Initialize\nmatrices"
      n30 = call "BRig_dataExp_init.vi"() -> ("output_dataExp"=w179:u16[])  [unwired: 11 in]
      n31 = call "BRig_dataLC_init.vi"() -> ("output_dataLC"=w180:u16[])  [unwired: 11 in]
      n32 = call "BRig_dataMTrig_init.vi"() -> ("output_dataMTrig"=w181:u16[])  [unwired: 5 in]
    }
    frame #6 {
      # "Load past data"
      n33 = call "BRig_RT_loadData_startup.vi"("input_dataMTrig"=w195, "input_dataLC"=w197, "input_dataExp"=w199) -> ("output_dataMTrig"=w194:u16[], "output_dataLC"=w196:u16[], "output_dataExp"=w198:u16[])  [unwired: 6 in]
    }
    frame #7 {
      w212 = TRUE ("input_setValues")
      # "Update\npanels"
      n34 = call "BRig_RT_panel_cue_v1,10.vi"("input_setValues"=w212, "input_dataExp"=w216) -> ()  [unwired: 9 in, 1 out]
      n35 = call "BRig_RT_panel_ExpStruct_v1,11.vi"("input_setValues"=w212, "input_dataExp"=w216) -> ()  [unwired: 9 in, 1 out]
      n36 = call "BRig_RT_panel_Laser1_v1,12.vi"("input_setValues"=w212, "input_dataExp"=w216, "input_dataLC"=w215) -> ()  [unwired: 7 in, 2 out]
      n37 = call "BRig_RT_panel_Laser2_v1,12.vi"("input_setValues"=w212, "input_dataExp"=w216, "input_dataLC"=w215) -> ()  [unwired: 7 in, 2 out]
      n38 = call "BRig_RT_panel_manualTriggering_v0,90.vi"("input_dataMTrig"=w214, "input_setValues"=w212) -> ("output_dataMTrig"=w213:u16[])  [unwired: 10 in, 7 out]
    }
    frame #8 {
      # "Unblock gui objects"
      n39 = property class="Bool (strict)"(reference=w239, "DisabledEnum"=T3."Enabled" ("Disabled")) -> ()  [unwired: 1 in, 2 out]
      n40 = property class="Bool (strict)"(reference=w238, "DisabledEnum"=T3."Enabled" ("Disabled")) -> ()  [unwired: 1 in, 2 out]
    }
  }
  n41 = Create Network Stream Writer Endpoint(7:w9, 9:w8, 11:"streamAnaIn_writer" ("reader name")) -> (0:w10:errorcluster, 3:w11:refnum<k21>)  [unwired: 4 in]
  n42 = Create Network Stream Writer Endpoint(7:w9, 9:w8, 11:"streamRT_stats__writer" ("writer name")) -> (0:w5:errorcluster, 3:w6:refnum<k21>)  [unwired: 4 in]
  n43 = case shown="True" w89 {
    tunnel: w121 -> [_ w284]
    tunnel: w96 -> [_ w283]
    tunnel: w95 -> [_ w282]
    tunnel: [w257 w281] -> w93
    tunnel: w92 -> [w257 w280]
    tunnel: w91 -> [_ w279]
    tunnel: w90 -> [_ w278]
    tunnel: w85 -> [w256 w277]
    tunnel: w84 -> [w255 w276]
    tunnel: w83 -> [w254 w275]
    tunnel: [w256 w274] -> w82
    tunnel: [w255 w273] -> w81
    tunnel: [w254 w272] -> w80
    tunnel: w79 -> [w253 w271]
    tunnel: w78 -> [w252 w270]
    tunnel: w77 -> [w251 w269]
    tunnel: [w253 w268] -> w76
    tunnel: [w252 w267] -> w75
    tunnel: [w251 w266] -> w74
    tunnel: [w250 w265] -> w14
    tunnel: [w249 w264] -> w13
    tunnel: w11 -> [w250 w263]
    tunnel: w10 -> [w249 w262]
    tunnel: w6 -> [w247 w261]
    tunnel: w5 -> [w246 w260]
    tunnel: [w247 w259] -> w2
    tunnel: [w246 w258] -> w1
    frame False {
      # "Error connecting to FPGA\nAbort"
      n44 = One Button Dialog(message="FPGA Error: Check that FPGA code was compiled") -> ()  [unwired: 1 in, 1 out]
    }
    frame True {
      # "dataExp"
      # "dataLaser"
      # "dataMTrig"
      n45 = while {
        tunnel: w283 -> [w322]
        tunnel: w282 -> [w327]
        tunnel: w284 -> [w330]
        tunnel: w284 -> [w329]
        tunnel: [w320] -> _
        tunnel: [w319] -> _
        shift-right: [w318] -> _
        shift-left: w278 -> [w314]
        shift-right: [w316] -> _
        shift-left: w279 -> [w317]
        shift-right: [w315] -> w281
        shift-left: w280 -> [w294]
        shift-right: [w309] -> w274
        shift-left: w277 -> [w312]
        shift-right: [w308] -> w273
        shift-left: w276 -> [w311]
        shift-right: [w307] -> w272
        shift-left: w275 -> [w310]
        shift-right: [w303] -> w268
        shift-left: w271 -> [w306]
        shift-right: [w302] -> w267
        shift-left: w270 -> [w305]
        shift-right: [w301] -> w266
        shift-left: w269 -> [w304]
        tunnel: [w292] -> w265
        tunnel: [w291] -> w264
        tunnel: w263 -> [w290]
        tunnel: w262 -> [w289]
        tunnel: w261 -> [w288]
        tunnel: w260 -> [w287]
        tunnel: [w286] -> w259
        tunnel: [w285] -> w258
        stop <- w328 stop-if-true
        # "set MTrig trigs to 0"
        # "dataExp"
        # "dataLaser"
        # "dataMTrig"
        # "Experiment or\nNonExperiment?"
        # "This loop allows for running multiple experiments in one session"
        n46 = local read "FPGA_count2ms"() -> (w298:dbl)
        n47 = xnode "Read/Write Control"("FPGA VI Reference In"=w322, "error in"=w327, "Counts_Reset"=TRUE) -> ("FPGA VI Reference Out"=w324:refnum<k20>, "error out"=w325:errorcluster)
        n48 = xnode "Read/Write Control"("FPGA VI Reference In"=w324, "error in"=w325, "Counts_Reset"=FALSE) -> ("FPGA VI Reference Out"=w321:refnum<k20>, "error out"=w323:errorcluster)
        n49 = call "BRig_dataMtrig_init__resetCounters.vi"("input_dataMTrig"=w314) -> ("output_dataMTrig"=w313:u16[])  [unwired: 10 in]
        n50 = call "BRig_dataExp_FPGA_count2ms.vi"() -> ("output_FPGA_count2ms"=w299:i32)  [unwired: 11 in]
        n51 = Multiply(x=w298, y=100.0) -> (x*y=w296:dbl)
        n52 = Round To Nearest(number=w296) -> (nearest integer value=w295:dbl)
        n53 = To Unsigned Word Integer(number=w295) -> (unsigned 16bit integer=w300:u16)
        n54 = Replace Array Subset(array=w294, new element=w300, index=w299) -> (w293:u16[])
        n55 = case shown="True" "START" {
          tunnel: w330 -> [w366 w941]
          tunnel: w329 -> [w365 w940]
          tunnel: w323 -> [w363 w929]
          tunnel: w321 -> [w364 w930]
          tunnel: [w361 w938] -> w320
          tunnel: [w359 w907] -> w319
          tunnel: w313 -> [w355 w927]
          tunnel: [w354 w913] -> w318
          tunnel: w317 -> [w353 w877]
          tunnel: w293 -> [w352 w830]
          tunnel: [w351 w912] -> w316
          tunnel: [w350 w911] -> w315
          tunnel: w312 -> [w349 w921]
          tunnel: w311 -> [w348 w920]
          tunnel: w310 -> [w347 w919]
          tunnel: [w346 w896] -> w309
          tunnel: [w345 w895] -> w308
          tunnel: [w344 w894] -> w307
          tunnel: w306 -> [w343 w876]
          tunnel: w305 -> [w342 w875]
          tunnel: w304 -> [w341 w874]
          tunnel: [w340 w903] -> w303
          tunnel: [w339 w902] -> w302
          tunnel: [w338 w904] -> w301
          tunnel: w290 -> [w336 w835]
          tunnel: w289 -> [w335 w834]
          tunnel: [w336 w833] -> w292
          tunnel: [w335 w832] -> w291
          tunnel: w288 -> [w334 w826]
          tunnel: w287 -> [w333 w827]
          tunnel: [w334 w821] -> w286
          tunnel: [w333 w820] -> w285
          frame False {
            # "dataExp"
            # "dataLaser"
            # "dataMTrig"
            n56 = node-c288() -> (w369:T5)  [unwired: 4 in]
            n57 = timed-loop {
              timing: w369 -> [_]
              timing-out: [_] -> w368
              shift-right: [w437] -> _
              shift-left: myRIO_BRig_RT__Case_NonExp_stateList."Init" ("Enum") -> [w406]
              shift-right: [w435] -> _
              shift-left: w366 -> [w436]
              shift-right: [w433] -> _
              shift-left: w365 -> [w434]
              tunnel: [w443] -> w362
              tunnel: [w419] -> w360
              tunnel: w363 -> [w426]
              tunnel: w364 -> [w444]
              shift-right: [w429] -> _
              shift-left: FALSE -> [w430]
              shift-right: [w427] -> _
              shift-left: 0.0 -> [w428]
              shift-right: [w416] -> _
              shift-left: FALSE -> [w417]
              shift-right: [w415] -> w354
              shift-left: w355 -> [w407]
              shift-right: [w401] -> w350
              shift-left: w352 -> [w404]
              shift-right: [w402] -> w351
              shift-left: w353 -> [w403]
              shift-right: [w400] -> w346
              shift-left: w349 -> [w396]
              shift-right: [w399] -> w345
              shift-left: w348 -> [w395]
              shift-right: [w398] -> w344
              shift-left: w347 -> [w394]
              shift-right: [w384] -> w340
              shift-left: w343 -> [w390]
              shift-right: [w385] -> w339
              shift-left: w342 -> [w389]
              shift-right: [w386] -> w338
              shift-left: w341 -> [w388]
              shift-right: [w379] -> _
              shift-left: u16 0 ("y") -> [w380]
              stop <- w446 stop-if-true
              # "dataExp"
              # "dataLaser"
              # "dataExp"
              # "dataLaser"
              # "dataMTrig"
              # "dataMTrig"
              n58 = node-c288() -> (w445:i64)  [unwired: 1 in]
              n59 = flat-sequence {
                tunnel: w426 -> [w475]
                tunnel: [w476] -> w418
                tunnel: [w475] -> w425
                frame #0 {
                  n60 = Get Date/Time In Seconds() -> (seconds since 1Jan1904=w476:timestamp)
                }
              }
              n61 = xnode "Read/Write Control"("FPGA VI Reference In"=w444, "error in"=w425) -> ("FPGA VI Reference Out"=w432:refnum<k20>, "error out"=w431:errorcluster, "A2_LickL"=w435:u32, "A4_LickR"=w433:u32)
              n62 = local write "cState_NonExp"(w406) -> ()
              n63 = local write "A2"(w435) -> ()
              n64 = local write "A4"(w433) -> ()
              n65 = case shown="\"Idle_2\"" w406 {
                selector: w406 -> [_ w483 _ _ _ _ _ _ _ _ w674 _ w682 _ _ w726 w769 w775]
                tunnel: [myRIO_BRig_RT__Case_NonExp_stateList."Idle" ("Enum") w484 myRIO_BRig_RT__Case_NonExp_stateList."UploadSettings_Read_dataLC" ("t") myRIO_BRig_RT__Case_NonExp_stateList."UploadSettings_Read_dataMTrig" ("t") myRIO_BRig_RT__Case_NonExp_stateList."UploadSettings_post" ("t") myRIO_BRig_RT__Case_NonExp_stateList."Idle" ("t") w565 w633 w657 w663 w672 myRIO_BRig_RT__Case_NonExp_stateList."RewardCalibration" ("Enum") w681 myRIO_BRig_RT__Case_NonExp_stateList."Idle" ("Enum") myRIO_BRig_RT__Case_NonExp_stateList."Idle" ("Enum") w725 w769 w776] -> w438
                tunnel: [w479 w490 w498 w516 w530 w545 w577 w649 w655 w664 w673 w676 w683 w697 w709 w735 w767 w784] -> w405
                tunnel: [_ _ _ _ _ _ _ _ _ _ _ _ _ _ _ _ TRUE _] -> w446
                tunnel: w407 -> [w479 w490 w498 w516 w527 w545 w577 w649 w655 w665 w675 w677 w684 w697 w709 w735 w767 w784]
                tunnel: w445 -> [_ _ _ _ _ _ _ _ _ _ _ _ _ _ _ _ _ _]
                tunnel: w436 -> [_ _ _ _ _ _ _ _ _ _ w670 _ _ _ _ _ _ _]
                tunnel: w435 -> [_ _ _ _ _ _ _ _ _ _ w671 _ _ _ _ _ _ _]
                tunnel: w434 -> [_ _ _ _ _ _ _ _ _ _ w668 _ _ _ _ _ _ _]
                tunnel: w433 -> [_ _ _ _ _ _ _ _ _ _ w669 _ _ _ _ _ _ _]
                tunnel: w432 -> [_ _ _ _ _ _ w632 _ w652 _ _ _ _ _ _ w730 _ _]
                tunnel: w431 -> [_ _ _ _ _ _ w631 _ w651 _ _ _ _ _ _ w729 _ _]
                tunnel: w430 -> [_ _ _ _ _ _ _ _ _ _ _ _ _ _ _ w734 _ _]
                tunnel: [_ _ _ _ _ _ _ _ _ _ _ _ _ _ _ TRUE _ _] -> w429
                tunnel: w428 -> [_ _ _ _ _ _ _ _ _ _ _ _ _ _ _ w732 _ _]
                tunnel: [_ _ _ _ _ _ _ _ _ _ _ _ _ _ _ w731 _ _] -> w427
                tunnel: w404 -> [w477 w488 w493 w515 w534 w547 w576 w647 w653 w661 w666 w679 w685 w694 w706 w722 w765 w782]
                tunnel: w403 -> [w478 w489 w497 w509 w531 w546 w578 w646 w654 w662 w667 w678 w686 w695 w707 w723 w766 w783]
                tunnel: [w478 w489 w497 w512 w531 w546 w578 w642 w654 w662 w667 w678 w686 w695 w707 w723 w766 w783] -> w402
                tunnel: [w477 w488 w492 w515 w534 w547 w576 w639 w653 w661 w666 w679 w685 w694 w706 w722 w765 w782] -> w401
                tunnel: [_ _ _ _ _ _ _ _ _ _ _ _ _ _ _ _ _ TRUE] -> w397
                tunnel: w396 -> [_ _ _ _ _ _ _ _ _ _ _ _ _ _ w700 _ _ w781]
                tunnel: w395 -> [_ _ _ _ _ _ _ _ _ _ _ _ _ _ w702 _ _ w777]
                tunnel: w394 -> [_ _ _ _ _ _ _ _ _ _ _ _ _ _ w701 _ _ w780]
                tunnel: [_ _ _ _ _ _ _ _ _ _ _ _ _ _ _ _ _ w779] -> w393
                tunnel: [_ _ _ _ _ _ _ _ _ _ _ _ _ _ _ _ _ w778] -> w392
                tunnel: [_ _ _ _ _ _ _ _ _ _ _ _ _ _ _ _ _ w770] -> w391
                tunnel: w388 -> [_ _ _ _ _ _ _ _ _ _ _ _ _ _ w699 _ _ _]
                tunnel: w389 -> [_ _ _ _ _ _ _ _ _ _ _ _ _ _ w705 _ _ _]
                tunnel: w390 -> [_ _ _ _ _ _ _ _ _ _ _ _ _ w687 w704 _ _ _]
                tunnel: [_ _ _ _ _ _ _ _ _ _ _ _ _ TRUE _ _ _ _] -> w387
                tunnel: [_ _ _ _ _ _ _ _ _ _ _ _ _ w689 _ _ _ _] -> w383
                tunnel: [_ _ _ _ _ _ _ _ _ _ _ _ _ w687 _ _ _ _] -> w382
                tunnel: [_ _ _ _ _ _ _ _ _ _ _ _ _ w688 _ _ _ _] -> w381
                tunnel: w380 -> [_ w482 _ _ _ _ _ _ _ _ _ _ _ _ _ _ _ _]
                tunnel: [_ w481 _ _ _ _ _ _ _ _ _ _ _ _ _ _ _ _] -> w379
                frame "Init", Default {
                  # "Only happens at start of NonExperiment Case"
                }
                frame "UploadSettings_pre" {
                  # "When the Host sends settings,\nnot all files send at the same time.\n\nIf RT reads the settings faster\nthan the Host can send them,\nthen we will skip settings.\n\nSolution:\nWait 20 cycles"
                  n66 = Increment(x=w482) -> (x+1=w481:u16)
                  n67 = Greater?(x=w481, y=u16 20) -> (0:w486:bool)
                  n68 = Select(t=myRIO_BRig_RT__Case_NonExp_stateList."UploadSettings_Read_dataExp", s=w486, f=w483) -> (s? t:f=w484:T1)
                }
                frame "UploadSettings_Read_dataExp" {
                  n69 = call "BRig_RT__Case_Idle__State_UploadSettings_checkFile.vi"("input_dataName"="dataExp") -> ("output_Iexist"=w495:bool, "output_dataPath"=w494:path)  [unwired: 9 in]
                  n70 = case shown="True" w495 {
                    tunnel: w494 -> [_ w501]
                    tunnel: w493 -> [w499 w505]
                    tunnel: [w499 w503] -> w492
                    frame False {
                    }
                    frame True {
                      n71 = call-poly <vilib>:"Read From Spreadsheet File.vi"("delimiter (\\t)"="," ("delimiter (\\t)"), "file path (dialog if empty)"=w501) -> ("first row"=w500:i64[])  [unwired: 5 in, 4 out]
                      n72 = Array Size(array=w500) -> (size(s)=w506:i32)
                      n73 = To Unsigned Word Integer(number=w500) -> (unsigned 16bit integer=w504:u16[])
                      n74 = flat-sequence {
                        tunnel: w501 -> [w508]
                        tunnel: w500 -> [_]
                        frame #0 {
                          n75 = Delete(path (use dialog)=w508) -> ()  [unwired: 4 in, 3 out]
                        }
                      }
                      n76 = Not Equal To 0?(x=w506) -> (x != 0?=w502:bool)
                      n77 = Select(t=w504, s=w502, f=w505) -> (s? t:f=w503:u16[])
                    }
                  }
                }
                frame "UploadSettings_Read_dataLC" {
                  n78 = call "BRig_RT__Case_Idle__State_UploadSettings_checkFile.vi"("input_dataName"="LC") -> ("output_Iexist"=w510:bool, "output_dataPath"=w511:path)  [unwired: 9 in]
                  n79 = case shown="True" w510 {
                    tunnel: w511 -> [_ w519]
                    tunnel: w509 -> [w517 w523]
                    tunnel: [w517 w521] -> w512
                    frame False {
                    }
                    frame True {
                      n80 = call-poly <vilib>:"Read From Spreadsheet File.vi"("delimiter (\\t)"="," ("delimiter (\\t)"), "file path (dialog if empty)"=w519) -> ("first row"=w518:i64[])  [unwired: 5 in, 4 out]
                      n81 = Array Size(array=w518) -> (size(s)=w524:i32)
                      n82 = To Unsigned Word Integer(number=w518) -> (unsigned 16bit integer=w522:u16[])
                      n83 = flat-sequence {
                        tunnel: w519 -> [w526]
                        tunnel: w518 -> [_]
                        frame #0 {
                          n84 = Delete(path (use dialog)=w526) -> ()  [unwired: 4 in, 3 out]
                        }
                      }
                      n85 = Not Equal To 0?(x=w524) -> (x != 0?=w520:bool)
                      n86 = Select(t=w522, s=w520, f=w523) -> (s? t:f=w521:u16[])
                    }
                  }
                }
                frame "UploadSettings_Read_dataMTrig" {
                  n87 = call "BRig_RT__Case_Idle__State_UploadSettings_checkFile.vi"("input_dataName"="MTrig") -> ("output_Iexist"=w528:bool, "output_dataPath"=w529:path)  [unwired: 9 in]
                  n88 = case shown="True" w528 {
                    tunnel: w529 -> [_ w537]
                    tunnel: w527 -> [w535 w541]
                    tunnel: [w535 w539] -> w530
                    frame False {
                    }
                    frame True {
                      n89 = call-poly <vilib>:"Read From Spreadsheet File.vi"("delimiter (\\t)"="," ("delimiter (\\t)"), "file path (dialog if empty)"=w537) -> ("first row"=w536:i64[])  [unwired: 5 in, 4 out]
                      n90 = Array Size(array=w536) -> (size(s)=w542:i32)
                      n91 = To Unsigned Word Integer(number=w536) -> (unsigned 16bit integer=w540:u16[])
                      n92 = flat-sequence {
                        tunnel: w537 -> [w544]
                        tunnel: w536 -> [_]
                        frame #0 {
                          n93 = Delete(path (use dialog)=w544) -> ()  [unwired: 4 in, 3 out]
                        }
                      }
                      n94 = Not Equal To 0?(x=w542) -> (x != 0?=w538:bool)
                      n95 = Select(t=w540, s=w538, f=w541) -> (s? t:f=w539:u16[])
                    }
                  }
                }
                frame "UploadSettings_post" {
                  w548 = TRUE ("input_setValues")
                  n96 = call "BRig_RT_panel_cue_v1,10.vi"("input_setValues"=w548, "input_dataExp"=w547) -> ()  [unwired: 9 in, 1 out]
                  n97 = call "BRig_RT_panel_ExpStruct_v1,11.vi"("input_setValues"=w548, "input_dataExp"=w547) -> ()  [unwired: 9 in, 1 out]
                  n98 = call "BRig_RT_panel_Laser1_v1,12.vi"("input_setValues"=w548, "input_dataExp"=w547, "input_dataLC"=w546) -> ()  [unwired: 7 in, 2 out]
                  n99 = call "BRig_RT_panel_Laser2_v1,12.vi"("input_setValues"=w548, "input_dataExp"=w547, "input_dataLC"=w546) -> ()  [unwired: 7 in, 2 out]
                  n100 = call "BRig_RT_panel_manualTriggering_v0,90.vi"("input_dataMTrig"=w545, "input_setValues"=w548) -> ()  [unwired: 10 in, 8 out]
                }
                frame "Idle" {
                  w622 = 100.0 ("y")
                  n101 = call "BRig_dataMTrig_Solenoid_T_L.vi"() -> ("output_Solenoid_T_L"=w560:i32)  [unwired: 11 in]
                  n102 = call "BRig_dataMTrig_Solenoid_T_R.vi"() -> ("output_Solenoid_T_R"=w559:i32)  [unwired: 11 in]
                  n103 = local read "FPGA_count2ms"() -> (w558:dbl)
                  n104 = call "BRig_dataExp_L_power_min_l1.vi"() -> ("output_L_power_min_l1"=w627:i32)  [unwired: 11 in]
                  n105 = call "BRig_dataExp_L_power_min_l2.vi"() -> ("output_L_power_min_l2"=w626:i32)  [unwired: 11 in]
                  n106 = call "BRig_dataExp_LED_baseline_Cue.vi"() -> ("output_LED_baseline_Cue"=w620:i32)  [unwired: 11 in]
                  n107 = call "BRig_dataExp_LED_baseline_l1.vi"() -> ("output_LED_baseline_l1"=w619:i32)  [unwired: 11 in]
                  n108 = call "BRig_dataExp_LED_baseline_l2.vi"() -> ("output_LED_baseline_l2"=w618:i32)  [unwired: 11 in]
                  n109 = call "BRig_dataExp_CueLed_Tpeak.vi"() -> ("output_CueLed_Tpeak"=w610:i32)  [unwired: 11 in]
                  n110 = call "BRig_dataExp_CueLed_freq.vi"() -> ("output_CueLed_Freq"=w609:i32)  [unwired: 11 in]
                  n111 = call "BRig_dataExp_L_Tpeak_l1.vi"() -> ("output_L_Tpeak_l1"=w602:i32)  [unwired: 11 in]
                  n112 = call "BRig_dataExp_L_freq_l1.vi"() -> ("output_L_freq_l1"=w601:i32)  [unwired: 11 in]
                  n113 = call "BRig_dataExp_L_Tshutter_l1.vi"() -> ("output_L_Tshutter_l1"=w600:i32)  [unwired: 11 in]
                  n114 = call "BRig_RT__Case_Idle__State_Idle__getAudioParam.vi"("input_dataExp"=w576, "input_dataMTrig"=w577) -> ("output_Audio_freq_R"=w572:u8, "output_Audio_amp_R"=w573:u16, "output_Audio_freq_L"=w574:u8, "output_Audio_amp_L"=w575:u16, "output_state"=w571:T1)  [unwired: 5 in]
                  n115 = call "BRig_dataExp_L_Tpeak_l2.vi"() -> ("output_L_Tpeak_l2"=w584:i32)  [unwired: 11 in]
                  n116 = call "BRig_dataExp_L_freq_l2.vi"() -> ("output_L_freq_l2"=w583:i32)  [unwired: 11 in]
                  n117 = call "BRig_dataExp_L_Tshutter_l2.vi"() -> ("output_L_Tshutter_l2"=w582:i32)  [unwired: 11 in]
                  n118 = local read "I_sendData"() -> (w570:bool)
                  n119 = Index Array(array=w576, index #1=w627, index #2=w626, index #3=w620, index #4=w619, index #5=w618, index #6=w610, index #7=w609, index #8=w602, index #9=w601, index #10=w600, index #11=w584, index #12=w583, index #13=w582, index #14=w560, index #15=w559) -> (element #1=w625:u16, element #2=w621:u16, element #3=w617:u16, element #4=w616:u16, element #5=w615:u16, element #6=w606:u16, element #7=w605:u16, element #8=w599:u16, element #9=w598:u16, element #10=w597:u16, element #11=w587:u16, element #12=w586:u16, element #13=w585:u16, element #14=w557:u16, element #15=w556:u16)
                  n120 = Select(t=myRIO_BRig_RT__Case_NonExp_stateList."SendData" ("Enum"), s=w570, f=w571) -> (s? t:f=w567:T1)
                  n121 = To Double Precision Float(number=w557) -> (double precision float=w555:dbl)
                  n122 = To Double Precision Float(number=w556) -> (double precision float=w554:dbl)
                  n123 = To Double Precision Float(number=w625) -> (double precision float=w624:dbl)
                  n124 = To Double Precision Float(number=w621) -> (double precision float=w623:dbl)
                  n125 = To Double Precision Float(number=w606) -> (double precision float=w608:dbl)
                  n126 = To Double Precision Float(number=w605) -> (double precision float=w607:dbl)
                  n127 = To Double Precision Float(number=w599) -> (double precision float=w596:dbl)
                  n128 = To Double Precision Float(number=w598) -> (double precision float=w595:dbl)
                  n129 = To Double Precision Float(number=w597) -> (double precision float=w594:dbl)
                  n130 = To Unsigned Word Integer(number=w558) -> (unsigned 16bit integer=w611:u16)
                  n131 = To Double Precision Float(number=w587) -> (double precision float=w588:dbl)
                  n132 = To Double Precision Float(number=w586) -> (double precision float=w589:dbl)
                  n133 = To Double Precision Float(number=w585) -> (double precision float=w590:dbl)
                  n134 = Not Equal To 0?(x=w615) -> (x != 0?=w612:bool)
                  n135 = Not Equal To 0?(x=w617) -> (x != 0?=w614:bool)
                  n136 = Not Equal To 0?(x=w616) -> (x != 0?=w613:bool)
                  n137 = Divide(x=w624, y=w622) -> (x/y=w551:dbl)
                  n138 = Divide(x=w623, y=w622) -> (x/y=w550:dbl)
                  n139 = local read "get_countPerMS"() -> (w566:bool)
                  n140 = Multiply(x=w558, y=w555) -> (x*y=w564:dbl)
                  n141 = Multiply(x=w558, y=w554) -> (x*y=w562:dbl)
                  n142 = call "BRig_RT__Case_Idle__calc_FPGA_CueLed.vi"("input_FPGA_ms2count"=w558, "input_Tpeak"=w608, "input_Freq"=w607) -> ("output_laser_Npeak"=w604:u32, "output_laser_Nvalley"=w603:u32)  [unwired: 11 in]
                  n143 = call "BRig_RT__Case_Idle__calc_FPGA_laser.vi"("input_FPGA_ms2count"=w558, "input_Tpeak"=w596, "input_Freq"=w595, "input_Tshutter"=w594) -> ("output_laser_Npeak"=w593:u32, "output_laser_Nvalley"=w592:u32, "output_laser_Nshutter"=w591:u32)  [unwired: 9 in]
                  n144 = call "BRig_RT__Case_Idle__calc_FPGA_laser.vi"("input_FPGA_ms2count"=w558, "input_Tpeak"=w588, "input_Freq"=w589, "input_Tshutter"=w590) -> ("output_laser_Npeak"=w581:u32, "output_laser_Nvalley"=w580:u32, "output_laser_Nshutter"=w579:u32)  [unwired: 9 in]
                  n145 = local write "L_Power_l1"(w551) -> ()
                  n146 = local write "L_Power_l2"(w550) -> ()
                  n147 = call "myRIO__convert__Voltage_to_FPGAvalue.vi"("input_voltage"=w551) -> ("output_PortC"=w628:i16)  [unwired: 9 in, 1 out]
                  n148 = call "myRIO__convert__Voltage_to_FPGAvalue.vi"("input_voltage"=w550) -> ("output_PortC"=w629:i16)  [unwired: 9 in, 1 out]
                  n149 = Round Toward +Infinity(x=w564) -> (ceil(x): smallest int >= x=w563:dbl)
                  n150 = Round Toward +Infinity(x=w562) -> (ceil(x): smallest int >= x=w561:dbl)
                  n151 = To Unsigned Long Integer(number=w563) -> (unsigned 32bit integer=w553:u32)
                  n152 = To Unsigned Long Integer(number=w561) -> (unsigned 32bit integer=w552:u32)
                  n153 = Select(t=myRIO_BRig_RT__Case_NonExp_stateList."Get_FPGA_count_per_ms" ("Enum"), s=w566, f=w567) -> (s? t:f=w565:T1)
                  n154 = xnode "Read/Write Control"("FPGA VI Reference In"=w632, "error in"=w631, "audioAmp_L"=w575, "audioFreq_L_kHz"=w574, "audioAmp_R"=w573, "audioFreq_R_kHz"=w572, "AnaOut_0"=w628, "AnaOut_1"=w629, "CueLed_Baseline"=w614, "L1Led_Baseline"=w613, "L2Led_Baseline"=w612, "k1__counter_per_ms"=w611, "CueLed_nPeak"=w604, "CueLed_nValley"=w603, "LC_nPeak_l1"=w593, "LC_nValley_l1"=w592, "LC_nShutter_l1"=w591, "LC_nPeak_l2"=w581, "LC_nValley_l2"=w580, "LC_nShutter_l2"=w579, "Solenoid_nTotal_L"=w553, "Solenoid_nTotal_R"=w552) -> ("error out"=w630:errorcluster)  [unwired: 1 out]
                  n155 = local write "error out"(w630) -> ()
                }
                frame "Idle_2" {
                  w638 = FALSE
                  n156 = call "BRig_RT_panel_cue_v1,10.vi"("input_setValues"=w638, "input_dataExp"=w647) -> ("output_dataExp"=w648:u16[])  [unwired: 9 in]
                  n157 = call "BRig_RT_panel_ExpStruct_v1,11.vi"("input_setValues"=w638, "input_dataExp"=w648) -> ("output_dataExp"=w641:u16[])  [unwired: 9 in]
                  n158 = local read "comm_TCP_connect"() -> (w637:bool)
                  n159 = call "BRig_RT_panel_Laser1_v1,12.vi"("input_setValues"=w638, "input_dataExp"=w641, "input_dataLC"=w646) -> ("output_dataExp"=w640:u16[], "output_dataLC"=w643:u16[])  [unwired: 7 in]
                  n160 = Select(t=myRIO_BRig_RT__Case_NonExp_stateList."commTCP_connect" ("Enum"), s=w637, f=myRIO_BRig_RT__Case_NonExp_stateList."Idle_6" ("Enum")) -> (s? t:f=w635:T1)
                  n161 = call "BRig_RT_panel_Laser2_v1,12.vi"("input_setValues"=w638, "input_dataExp"=w640, "input_dataLC"=w643) -> ("output_dataExp"=w639:u16[], "output_dataLC"=w642:u16[])  [unwired: 7 in]
                  n162 = local read "comm_WebDAV_connect"() -> (w636:bool)
                  n163 = Select(t=myRIO_BRig_RT__Case_NonExp_stateList."TestConnection" ("Enum"), s=w636, f=w635) -> (s? t:f=w633:T1)
                }
                frame "Idle_6" {
                  n164 = local read "lick_Rising(F)_or_Falling(T)"() -> (w650:bool)
                  n165 = call "BRig_RT__Case_Idle__State_UploadSettings_checkFile.vi"("input_dataName"="dataExp") -> ("output_Iexist"=w659:bool)  [unwired: 9 in, 1 out]
                  n166 = xnode "Read/Write Control"("FPGA VI Reference In"=w652, "error in"=w651, "Rising(F)_or_Falling(T)"=w650) -> ()  [unwired: 2 out]
                  n167 = Select(t=myRIO_BRig_RT__Case_NonExp_stateList."UploadSettings_pre" ("Enum"), s=w659, f=myRIO_BRig_RT__Case_NonExp_stateList."Idle") -> (s? t:f=w657:T1)
                }
                frame "Cue_pre" {
                  n168 = call "BRig_RT__Case_Idle__State_Cue_pre__v2.vi"("input_dataExp"=w661, "input_dataMTrig"=w665) -> ("output_dataMTrig"=w664:u16[], "output_state"=w663:T1)  [unwired: 8 in]
                }
                frame "Cue" {
                  n169 = call "BRig_RT__Case_Idle__State_Cue__v2.vi"("input_cLick_R_prev"=w668, "input_cLick_R"=w669, "input_state"=w674, "input_cLick_L_prev"=w670, "input_cLick_L"=w671, "input_dataMTrig"=w675) -> ("output_dataMTrig"=w673:u16[], "output_state"=w672:T1)  [unwired: 4 in]
                }
                frame "RewardCalibration_pre" {
                  n170 = call "BRig_RT__Case_Idle__State_RewardCalibration_pre__v2.vi"("input_dataMTrig"=w677) -> ("output_dataMTrig"=w676:u16[])  [unwired: 26 in]
                }
                frame "RewardCalibration" {
                  n171 = call "BRig_RT__Case_Idle__State_RewardCalibration.vi"("input_state"=w682, "input_dataMTrig"=w684) -> ("output_dataMtrig"=w683:u16[], "output_state"=w681:T1)  [unwired: 8 in]
                }
                frame "TestConnection" {
                  n172 = local read "Host Password"() -> (w690:string)
                  n173 = local read "Host UserName"() -> (w691:string)
                  n174 = call "BRig_RT_comm_webdav_connect.vi"("input_password"=w690, "input_username"=w691) -> ("output_Iconnected"=w689:bool, "output_hSession"=w688:T4)  [unwired: 6 in, 2 out]
                  n175 = local write "comm_WebDAV_connect"(FALSE ("comm_WebDAV_connect")) -> ()
                  n176 = local write "comm_WebDAV"(w689) -> ()
                }
                frame "SendData" {
                  n177 = And(x=w700, y=w699) -> (x .and. y?=w698:bool)
                  n178 = case shown="True" w698 {
                    tunnel: w699 -> [_ w717]
                    tunnel: w705 -> [_ w716]
                    tunnel: w704 -> [_ w715]
                    tunnel: w702 -> [_ w713]
                    tunnel: w701 -> [_ w712]
                    frame False {
                      n179 = One Button Dialog(message="Unable to send data:\n Missing one or more\n connections") -> ()  [unwired: 1 in, 1 out]
                    }
                    frame True {
                      n180 = local read "Data Set Prefix"() -> (w718:string)
                      n181 = call "BRig_RT_comm_webdav_upload_all__v3.vi"("input_I_connected_webdav"=w717, "input_fileName_prefix"=w718, "input_hSession"=w716, "input_error"=w715, "input_True"=TRUE) -> ("output_nFilenames"=w719:i32, "output_arrFilenames"=w720:string[], "output_uploaded"=w721:bool[], "output_strCmd"=w714:string)  [unwired: 5 in, 2 out]
                      n182 = call "BRig_RT_comm_tcp_write_RTwrite.vi"("input_error"=w712, "input_packet"=w714, "input_hTCP"=w713) -> ()  [unwired: 5 in, 4 out]
                      n183 = call "BRig_RT_comm_webdav_upload_all_warnUser.vi"("input_n"=w719, "input_arrFilenames"=w720, "input_arrUploaded"=w721) -> ()  [unwired: 9 in]
                    }
                  }
                  n184 = local write "I_sendData"(FALSE ("I_sendData")) -> ()
                }
                frame "Get_FPGA_count_per_ms" {
                  # "Used to automatically determine how many FPGA cycles in 1 ms"
                  n185 = case shown="True" w734 {
                    selector: w734 -> [w736 _]
                    tunnel: w732 -> [_ w749]
                    tunnel: [w740 w749] -> w731
                    tunnel: w730 -> [w739 w747]
                    tunnel: w729 -> [w738 w746]
                    tunnel: [w737 w744] -> w724
                    tunnel: [w736 w743] -> w728
                    frame False {
                      n186 = Get Date/Time In Seconds() -> (seconds since 1Jan1904=w741:timestamp)
                      n187 = To Double Precision Float(number=w741) -> (double precision float=w740:dbl)
                      n188 = xnode "Read/Write Control"("FPGA VI Reference In"=w739, "error in"=w738, "timeTrial_trig"=TRUE ("timeTrial")) -> ("error out"=w737:errorcluster)  [unwired: 1 out]
                      n189 = local write "get_countPerMS"(w736) -> ()
                    }
                    frame True {
                      w745 = 1.0
                      n190 = Get Date/Time In Seconds() -> (seconds since 1Jan1904=w750:timestamp)
                      n191 = To Double Precision Float(number=w750) -> (double precision float=w751:dbl)
                      n192 = Subtract(x=w751, y=w749) -> (x-y=w748:dbl)
                      n193 = Less Or Equal?(x=w745, y=w748) -> (x <= y?=w743:bool)
                      n194 = case shown="True" w743 {
                        tunnel: w747 -> [_ w764]
                        tunnel: w746 -> [w752 w763]
                        tunnel: w745 -> [_ w754]
                        tunnel: [w752 w753] -> w744
                        frame False {
                        }
                        frame True {
                          n195 = xnode "Read/Write Control"("FPGA VI Reference In"=w764, "error in"=w763) -> ("FPGA VI Reference Out"=w761:refnum<k20>, "error out"=w760:errorcluster, "timeTrial_count"=w755:u32)
                          n196 = Multiply(x=w754, y=1000.0) -> (x*y=w758:dbl)
                          n197 = To Double Precision Float(number=w755) -> (double precision float=w757:dbl)
                          n198 = Divide(x=w757, y=w758) -> (x/y=w759:dbl)
                          n199 = local write "FPGA_count2ms"(w759) -> ()
                          n200 = xnode "Read/Write Control"("FPGA VI Reference In"=w761, "error in"=w760, "timeTrial_trig"=FALSE ("timeTrial")) -> ("error out"=w753:errorcluster)  [unwired: 1 out]
                        }
                      }
                    }
                  }
                  n201 = Select(t=myRIO_BRig_RT__Case_NonExp_stateList."Idle" ("Enum"), s=w728, f=w726) -> (s? t:f=w725:T1)
                  n202 = local write "error out"(w724) -> ()
                }
                frame "End" {
                }
                frame "commTCP_connect" {
                  n203 = local read "comm_TCP_connect"() -> (w774:bool)
                  n204 = case shown="True" w781 {
                    tunnel: w780 -> [w791 w800]
                    tunnel: [w790 w796] -> w778
                    tunnel: [w789 w793] -> w770
                    tunnel: [w788 w794] -> w779
                    tunnel: w777 -> [_ w801]
                    frame False {
                      n205 = call "BRig_RT_comm_tcp_connect_RTwrite.vi"("input_error"=w791) -> ("output_error"=w788:errorcluster, "output_connected"=w789:bool, "output_hTCP"=w790:refnum<k5>)  [unwired: 8 in]
                    }
                    frame True {
                      n206 = call "BRig_RT_comm_tcp_write_RTwrite.vi"("input_error"=w800, "input_packet"="<test>", "input_hTCP"=w801) -> ("output_error"=w795:errorcluster, "output_I_NotDisconnected"=w792:bool, "output_I_write"=w798:bool, "output_hTCP"=w797:refnum<k5>)  [unwired: 5 in]
                      n207 = case shown="False" w798 {
                        selector: w798 -> [_ w812]
                        tunnel: w797 -> [w807 w814]
                        tunnel: [w802 w814] -> w796
                        tunnel: w795 -> [w806 w813]
                        tunnel: [w804 w813] -> w794
                        tunnel: [w803 w812] -> w793
                        tunnel: w792 -> [w808 _]
                        frame False {
                          n208 = case shown="True" w808 {
                            tunnel: w807 -> [_ w811]
                            tunnel: w806 -> [w809 w810]
                            tunnel: [w809 w810] -> w805
                            frame False {
                            }
                            frame True {
                              n209 = TCP Close Connection(connection ID=w811, error in (no error)=w810) -> ()  [unwired: 1 in, 2 out]
                            }
                          }
                          n210 = call "BRig_RT_comm_tcp_connect_RTwrite.vi"("input_error"=w805) -> ("output_error"=w804:errorcluster, "output_connected"=w803:bool, "output_hTCP"=w802:refnum<k5>)  [unwired: 8 in]
                        }
                        frame True {
                        }
                      }
                    }
                  }
                  n211 = Not(x=w774) -> (.not. x?=w773:bool)
                  n212 = Or(x=w773, y=w770) -> (x .or. y?=w772:bool)
                  n213 = case shown="True" w772 {
                    tunnel: [w785 myRIO_BRig_RT__Case_NonExp_stateList."Idle" ("Enum")] -> w776
                    tunnel: w775 -> [w785 _]
                    frame False {
                    }
                    frame True {
                      n214 = local write "comm_TCP_connect"(FALSE) -> ()
                    }
                  }
                  n215 = local write "comm_TCP"(w770) -> ()
                }
              }
              n216 = case shown="True" w397 {
                tunnel: [w455 w456] -> w400
                tunnel: [w454 w457] -> w399
                tunnel: [w453 w458] -> w398
                tunnel: w396 -> [w455 _]
                tunnel: w395 -> [w454 _]
                tunnel: w394 -> [w453 _]
                tunnel: w393 -> [_ w458]
                tunnel: w392 -> [_ w457]
                tunnel: w391 -> [_ w456]
                frame False {
                }
                frame True {
                }
              }
              n217 = case shown="True" w387 {
                tunnel: [w449 w450] -> w386
                tunnel: [w448 w451] -> w385
                tunnel: [w447 w452] -> w384
                tunnel: w388 -> [w449 _]
                tunnel: w389 -> [w448 _]
                tunnel: w390 -> [w447 _]
                tunnel: w382 -> [_ w452]
                tunnel: w381 -> [_ w451]
                tunnel: w383 -> [_ w450]
                frame False {
                }
                frame True {
                }
              }
              n218 = flat-sequence {
                tunnel: w420 -> [w462]
                tunnel: w418 -> [w460]
                tunnel: [w462] -> w424
                tunnel: [w461] -> w423
                tunnel: [w460] -> w422
                tunnel: [w459] -> w421
                tunnel: w417 -> [w459]
                tunnel: [w474] -> w419
                tunnel: w424 -> [w474]
                tunnel: w423 -> [w473]
                tunnel: w422 -> [w471]
                tunnel: w421 -> [w466]
                tunnel: [w465] -> w416
                frame #0 {
                  n219 = Get Date/Time In Seconds() -> (seconds since 1Jan1904=w461:timestamp)
                }
                frame #1 {
                  # "threshold"
                  # "delta T [ms]"
                  # "delta T [s]"
                  n220 = To Double Precision Float(number=w473) -> (double precision float=w472:dbl)
                  n221 = To Double Precision Float(number=w471) -> (double precision float=w470:dbl)
                  n222 = Subtract(x=w472, y=w470) -> (x-y=w469:dbl)
                  n223 = Multiply(x=w469, y=1000.0) -> (x*y=w464:dbl)
                  n224 = Greater?(x=w464, y=5.0) -> (0:w463:bool)
                  n225 = local write "Threshold"(w463) -> ()
                  n226 = local write "tLoop"(w464) -> ()
                  n227 = Or(x=w463, y=w466) -> (x .or. y?=w465:bool)
                }
              }
              n228 = local read "START"() -> (w441:bool)
              n229 = local read "STOP_abort"() -> (w440:bool)
              n230 = local read "Laser1_LED"() -> (w378:bool)
              n231 = local read "Laser2_LED"() -> (w377:bool)
              n232 = call "BRig_RT_panel_manualTriggering_v0,90.vi"("input_dataMTrig"=w405) -> ("output_Solenoid_R"=w408:bool, "output_Solenoid_L"=w409:bool, "output_dataMTrig"=w415:u16[], "output_Audio_L"=w410:bool, "output_Audio_R"=w411:bool, "output_CueLed"=w412:bool, "output_Laser_l1"=w413:bool, "output_Laser_l2"=w414:bool)  [unwired: 11 in]
              n233 = Or(x=w441, y=w440) -> (x .or. y?=w439:bool)
              n234 = Select(t=myRIO_BRig_RT__Case_NonExp_stateList."End" ("Enum"), s=w439, f=w438) -> (s? t:f=w437:T1)
              n235 = xnode "Read/Write Control"("FPGA VI Reference In"=w432, "error in"=w431, "A1_SR"=w408, "A3_SL"=w409, "audioTrigger_L"=w410, "audioTrigger_R"=w411, "LC_Laser_l1"=w413, "LC_Laser_l2"=w414, "CueLed_Event"=w412, "L1Led_ON"=w378, "L2Led_ON"=w377) -> ("FPGA VI Reference Out"=w443:refnum<k20>, "error out"=w420:errorcluster, "fpga_laser1"=w373:bool, "fpga_laser2"=w374:bool, "fpga_solenoid_L"=w375:bool, "fpga_solenoid_R"=w376:bool)
              n236 = local write "Laser1"(w373) -> ()
              n237 = local write "Laser2"(w374) -> ()
              n238 = local write "Solenoid L"(w375) -> ()
              n239 = local write "Solenoid R"(w376) -> ()
              n240 = node-c288() -> ()  [unwired: 1 in, 1 out]
            }
            n241 = node-c288(w368) -> ()  [unwired: 1 out]
            n242 = flat-sequence {
              tunnel: w362 -> [w372]
              tunnel: [w372] -> w361
              tunnel: w360 -> [w371]
              tunnel: [w371] -> w359
              frame #0 {
                w370 = FALSE
                n243 = local write "STOP_endBlock"(w370) -> ()
                n244 = local write "STOP_endTrial"(w370) -> ()
              }
            }
          }
          frame True {
            w884 = ".csv" ("string")
            w914 = ""
            w923 = u8 0
            w924 = u16 0 ("AudioLeft_phase_inc")
            w925 = FALSE
            # "buffer_dataRT_stats"
            # "Clear local files"
            # "empty array"
            # "buffer_dataBlock"
            # "buffer_dataTrial"
            # "nColumns dataBlock"
            # "nColumns dataTrial"
            # "buffer_dataBlock"
            # "buffer_dataTrial"
            # "nColumns\ndataBlock"
            # "nColumns\ndataTrial"
            # "original dataExp and dataLC"
            # "dataLick"
            # "dataTrial"
            # "dataBlock"
            # "dataCurrent"
            # "arrTrig"
            # "time stamp"
            # "dummyState counter"
            # "dataTrial"
            # "dataLick"
            # "dataLC"
            # "dataLC"
            # "dataBlock"
            # "dataMTrig"
            # "dataMTrig"
            # "dataExp"
            # "dataExp"
            # "dataCurrent"
            # "state"
            n245 = flat-sequence {
              tunnel: [w1021] -> w854
              tunnel: [w1020] -> w858
              tunnel: [w1029] -> w872
              tunnel: [w1028] -> w871
              tunnel: [myRIO_BRig_RT__Case_Exp_stateList."Start1" ("Enum")] -> w870
              tunnel: [w1026] -> w869
              tunnel: [u16 0] -> w868
              tunnel: [w1024] -> w867
              tunnel: [w1023] -> w866
              tunnel: [w1022] -> w865
              tunnel: [w1031] -> w880
              tunnel: [w1032] -> w881
              tunnel: [w1033] -> w931
              tunnel: [w1034] -> w933
              tunnel: [w1035] -> w934
              tunnel: [w1036] -> w935
              tunnel: [w1037] -> w936
              tunnel: [w1038] -> w937
              tunnel: w872 -> [w1038]
              tunnel: w871 -> [w1037]
              tunnel: w870 -> [w1036]
              tunnel: w869 -> [w1035]
              tunnel: w868 -> [w1034]
              tunnel: w867 -> [w1033]
              tunnel: w866 -> [w1032]
              tunnel: w865 -> [w1031]
              tunnel: [w1030] -> w863
              frame #0 {
                n246 = call "BRig_dataBlock_init.vi"() -> ("output_nCol"=w1020:i32, "output_dataBlock"=w1022:u16[][])  [unwired: 10 in]
                n247 = call "BRig_dataCurrent_init.vi"() -> ("output_dataCurrent"=w1029:u16[])  [unwired: 11 in]
                n248 = call "BRig_dataLick_init.vi"() -> ("output_dataLick"=w1028:u16[][])  [unwired: 11 in]
                n249 = call "BRig_dataTrial_init.vi"() -> ("output_nCol"=w1021:i32, "output_dataTrial"=w1023:u16[][])  [unwired: 10 in]
                n250 = Get Date/Time In Seconds() -> (seconds since 1Jan1904=w1019:timestamp)
                n251 = To Double Precision Float(number=w1019) -> (double precision float=w1026:dbl)
                n252 = call "BRig_arrTrig_init.vi"() -> ("output_arrTrig"=w1024:bool[])  [unwired: 11 in]
              }
              frame #1 {
                w1030 = u32 2 ("milliseconds to wait")
                n253 = Wait (ms)(milliseconds to wait=w1030) -> ()  [unwired: 1 out]
              }
            }
            n254 = flat-sequence {
              tunnel: w860 -> [w1000]
              tunnel: [w1000] -> w859
              tunnel: w859 -> [w1009]
              tunnel: [w1007] -> w842
              tunnel: [w1006] -> w829
              tunnel: [w1003] -> w857
              tunnel: w858 -> [w1002]
              tunnel: w854 -> [w1001]
              tunnel: [w1009] -> w856
              tunnel: w856 -> [w1011]
              tunnel: [w1011] -> w855
              tunnel: w855 -> [w1017]
              tunnel: w854 -> [w1016]
              tunnel: [w1014] -> w849
              tunnel: [w1012] -> w852
              tunnel: [w1017] -> w853
              tunnel: [w1018] -> _
              tunnel: w853 -> [w1018]
              frame #0 {
                n255 = Wait (ms)(milliseconds to wait=w1000) -> ()  [unwired: 1 out]
              }
              frame #1 {
                w1004 = u16 0 ("element")
                n256 = Initialize Array(w1004, 8 ("dimension size")) -> (w1007:u16[])
                n257 = Initialize Array(w1004, 100 ("dimension size"), w1001) -> (w1006:u16[][])
                n258 = Initialize Array(w1004, 10 ("dimension size"), w1002) -> (w1003:u16[][])
              }
              frame #2 {
                n259 = Wait (ms)(milliseconds to wait=w1011) -> ()  [unwired: 1 out]
              }
              frame #3 {
                n260 = Increment(x=w1016) -> (x+1=w1013:i32)
                n261 = To Unsigned Long Integer(number=w1013) -> (unsigned 32bit integer=w1012:u32)
                n262 = Initialize Array(u16 0 ("element"), w1013) -> (w1014:u16[])
              }
              frame #4 {
                n263 = Wait (ms)(milliseconds to wait=w1018) -> ()  [unwired: 1 out]
              }
            }
            n264 = call "BRig_comm_webdav_myrioFolder.vi"() -> ("output_myrioFolder"=w885:string)  [unwired: 11 in]
            n265 = local write "stop_TimedLoop"(FALSE ("stop_TimedLoop")) -> ()
            n266 = RT FIFO Create(0:"dataTrialOrBlock" ("name (unnamed)"), 1:w849, 4:u32 40 ("size (10)"), 6:w852, 7:T8 {"read mode"=enum."blocking", "write mode"=enum."blocking"} ("r/w modes (polling,polling)")) -> (8:w851:refnum<k33>, 11:w850:errorcluster)  [unwired: 3 in, 1 out]
            n267 = RT FIFO Create(0:"dataAnalog" ("name (unnamed)"), 1:u16 0 ("element"), 4:u32 1000 ("size (10)")) -> (8:w837:refnum<k33>, 11:w836:errorcluster)  [unwired: 5 in, 1 out]
            n268 = Concatenate Strings(w885, "dataTrial" ("input_filename"), w884) -> (w886:string)
            n269 = Concatenate Strings(w885, "dataBlock" ("input_filename"), w884) -> (w887:string)
            n270 = String To Path(string=w886) -> (path=w890:path)
            n271 = String To Path(string=w887) -> (path=w882:path)
            n272 = flat-sequence {
              tunnel: [w1039] -> w864
              tunnel: w863 -> [w1039]
              tunnel: w864 -> [w1040]
              tunnel: [w1040] -> w861
              tunnel: w877 -> [w1043]
              tunnel: w830 -> [w1042]
              tunnel: [w1041] -> w862
              tunnel: w861 -> [w1041]
              tunnel: [w1047] -> _
              tunnel: w876 -> [w1047]
              tunnel: w875 -> [w1046]
              tunnel: w874 -> [w1045]
              tunnel: [w1044] -> w860
              tunnel: w862 -> [w1044]
              frame #0 {
                n273 = call "BRig_RT__Case_Exp__clearLocalFolder.vi"() -> ()  [unwired: 12 in]
              }
              frame #1 {
                n274 = Wait (ms)(milliseconds to wait=w1040) -> ()  [unwired: 1 out]
              }
              frame #2 {
                n275 = call "BRig_RT__Case_Exp__State_start__sendExpData_saveData.vi"("input_dataLC"=w1043, "input_dataExp"=w1042) -> ()  [unwired: 10 in]
              }
              frame #3 {
                n276 = call "BRig_RT__Case_Exp__State_start__sendExpData_uploadData__v2.vi"("input_error"=w1047, "input_hSession"=w1046, "input_connected"=w1045) -> ()  [unwired: 8 in, 1 out]
              }
            }
            n277 = call "BRig_RT__Case_Exp__comm_tcp__data_other.vi"("input_strState"=w914, "input_strAccum"=w914, "input_error"=w919, "input_hTCP"=w920, "input_I_connected_TCP"=w921) -> ("output_strAccum"=w915:string, "output_error"=w916:errorcluster, "output_hTCP"=w917:refnum<k5>, "output_I_connect_TCP"=w918:bool)  [unwired: 3 in]
            n278 = Initialize Array(u16 0 ("element"), 30 ("dimension size")) -> (w824:u16[])
            n279 = node-c288() -> (w943:T5)  [unwired: 4 in]
            n280 = timed-loop {
              timing: w943 -> [_]
              timing-out: [_] -> w942
              shift-right: [w1333] -> _
              shift-left: w935 -> [w1288]
              tunnel: w930 -> [w1377]
              tunnel: w929 -> [w1357]
              shift-right: [w1321] -> _
              shift-left: w941 -> [w1376]
              shift-right: [w1320] -> _
              shift-left: w940 -> [w1375]
              tunnel: [w1368] -> w922
              tunnel: [w1369] -> w939
              shift-right: [w1331] -> w910
              shift-left: w937 -> [w1305]
              shift-right: [w1374] -> w911
              shift-left: w830 -> [w1307]
              shift-right: [w1351] -> w913
              shift-left: w927 -> [w1308]
              shift-right: [w1372] -> _
              shift-left: w880 -> [w1373]
              shift-right: [w1370] -> w912
              shift-left: w877 -> [w1371]
              shift-right: [w1327] -> w909
              shift-left: w936 -> [w1334]
              shift-right: [w1367] -> _
              shift-left: w881 -> [w1306]
              tunnel: w934 -> [w1366]
              shift-right: [w1340] -> _
              shift-left: u16 0 -> [w1339]
              shift-right: [w1360] -> _
              shift-left: w933 -> [w1361]
              shift-right: [w1358] -> _
              shift-left: w931 -> [w1359]
              shift-right: [w1352] -> _
              shift-left: FALSE -> [w1354]
              shift-right: [w1296] -> w901
              shift-left: w918 -> [w1315]
              shift-right: [w1295] -> w900
              shift-left: w917 -> [w1314]
              shift-right: [w1293] -> w899
              shift-left: w916 -> [w1313]
              shift-right: [w1294] -> _
              shift-left: w915 -> [w1312]
              shift-right: [w1302] -> w906
              shift-left: w876 -> [w1302]
              shift-right: [w1304] -> w904
              shift-left: w874 -> [w1304]
              shift-right: [w1303] -> w905
              shift-left: w875 -> [w1303]
              shift-right: [w1301] -> _
              shift-left: _ -> [w1299]
              shift-right: [w1300] -> _
              shift-left: _ -> [w1298]
              tunnel: [w1297] -> w893
              tunnel: w851 -> [w1291]
              tunnel: w850 -> [w1290]
              tunnel: w849 -> [w1289]
              tunnel: w837 -> [w1287]
              tunnel: w836 -> [w1286]
              tunnel: w830 -> [w1285]
              stop <- w1297 stop-if-true
              # "iOccurrence"
              # "index"
              # "resetOccurrence?\ndataAnalog"
              # "dataLick"
              # "dataLick"
              # "dummyState counter"
              # "dummyState counter"
              # "iOccurrence"
              # "arrTrig"
              # "arrTrig"
              # "CueLed"
              # "LC_Laser_l2"
              # "LC_Event_l2"
              # "LC_Laser_l1"
              # "LC_Event_l1"
              # "iState"
              # "dataAnalog"
              # "index"
              # "manual triggering"
              # "dataTrial"
              # "dataBlock"
              # "dataExp"
              # "dataCurrent"
              # "time stamp"
              # "audio__L\naudio__R"
              # "dataLC"
              # "solenoid__R"
              # "solenoid__L"
              # "Did a lick occur?"
              # "Update lick counter"
              # "state"
              # "state"
              n281 = node-c288() -> ()  [unwired: 1 in, 1 out]
              n282 = local write "cState"(w1288) -> ()
              n283 = flat-sequence {
                tunnel: w1357 -> [w1378]
                tunnel: [w1379] -> w1355
                tunnel: [w1378] -> w1356
                frame #0 {
                  n284 = Get Date/Time In Seconds() -> (seconds since 1Jan1904=w1379:timestamp)
                }
              }
              n285 = xnode "Read/Write Control"("FPGA VI Reference In"=w1377, "error in"=w1356) -> ("FPGA VI Reference Out"=w1363:refnum<k20>, "error out"=w1362:errorcluster, "A2_LickL"=w1321:u32, "A4_LickR"=w1320:u32)
              n286 = local write "A2"(w1321) -> ()
              n287 = local write "A4"(w1320) -> ()
              n288 = Greater?(x=w1321, y=w1376) -> (0:w1329:bool)
              n289 = Greater?(x=w1320, y=w1375) -> (0:w1328:bool)
              n290 = Or(x=w1329, y=w1328) -> (x .or. y?=w1330:bool)
              n291 = case shown="\"initTrial2\"" w1288 {
                selector: w1288 -> [_ _ _ _ _ _ _ _ _ _ _ _ _ _ w1634 w1650 _ w1679 _ _ w1726 w1753 _ w1779 _ w1823 _ w1875 _ w1895 _ w1961 _ w2031 _ _ _ _ w2149 _ w2173 w2204 w2225 w2250 _ w2315 w2325 _]
                tunnel: [myRIO_BRig_RT__Case_Exp_stateList."Start2" ("Enum") myRIO_BRig_RT__Case_Exp_stateList."Start3" ("Enum") myRIO_BRig_RT__Case_Exp_stateList."saveSettings1" ("Enum") myRIO_BRig_RT__Case_Exp_stateList."initBlock" ("Enum") myRIO_BRig_RT__Case_Exp_stateList."initTrial_LC_ENL1" ("Enum") myRIO_BRig_RT__Case_Exp_stateList."initTrial" ("Enum") myRIO_BRig_RT__Case_Exp_stateList."initTrial2" ("Enum") myRIO_BRig_RT__Case_Exp_stateList."setSettings_Laser" ("Enum") myRIO_BRig_RT__Case_Exp_stateList."ENL1_pre" ("Enum") myRIO_BRig_RT__Case_Exp_stateList."initTrial_LC_Cue1" ("Enum") myRIO_BRig_RT__Case_Exp_stateList."initTrial_LC_Sel" ("Enum") myRIO_BRig_RT__Case_Exp_stateList."initTrial4" ("Enum") w1612 w1624 w1632 w1648 myRIO_BRig_RT__Case_Exp_stateList."ENL1Penalty" ("Enum") w1677 w1692 w1704 w1725 w1752 myRIO_BRig_RT__Case_Exp_stateList."Cue1Penalty" ("Enum") w1780 w1796 w1818 myRIO_BRig_RT__Case_Exp_stateList."SelectReward" ("Enum") w1874 myRIO_BRig_RT__Case_Exp_stateList."SelectRewardPost" ("Enum") w1894 myRIO_BRig_RT__Case_Exp_stateList."SelectWrong" ("Enum") w1960 myRIO_BRig_RT__Case_Exp_stateList."SelectTimeout" ("Enum") w2030 myRIO_BRig_RT__Case_Exp_stateList."saveData_dataTrial" ("Enum") w2065 w2100 w2138 w2149 myRIO_BRig_RT__Case_Exp_stateList."initBlock" ("Enum") w2171 w2205 w2224 w2249 myRIO_BRig_RT__Case_Exp_stateList."FreeReward" ("Enum") w2313 w2323 myRIO_BRig_RT__Case_Exp_stateList."FreeRewardPost" ("Enum")] -> w1333
                tunnel: w1330 -> [_ _ _ _ _ _ _ _ _ _ _ _ w1613 w1625 w1633 w1649 _ _ w1693 w1705 w1727 w1754 _ _ _ _ _ _ _ _ _ _ _ _ _ _ _ _ _ _ _ _ _ _ _ _ _ _]
                tunnel: w1329 -> [_ _ _ _ _ _ _ _ _ _ _ _ _ _ _ _ _ _ _ _ _ _ _ _ w1788 w1819 _ _ _ _ _ _ _ _ _ _ _ _ _ _ _ _ _ _ _ _ _ _]
                tunnel: w1328 -> [_ _ _ _ _ _ _ _ _ _ _ _ _ _ _ _ _ _ _ _ _ _ _ _ w1787 w1820 _ _ _ _ _ _ _ _ _ _ _ _ _ _ _ _ _ _ _ _ _ _]
                tunnel: w1305 -> [w1389 w1395 w1427 w1431 w1452 w1504 w1517 w1530 w1557 w1572 w1582 w1599 w1611 w1623 w1641 w1657 w1668 w1676 w1694 w1706 w1728 w1755 w1772 w1778 w1799 w1816 w1860 w1871 w1883 w1893 w1922 w1959 w1992 w2029 w2044 w2071 w2109 w2128 w2148 w2155 w2174 w2207 w2223 w2240 w2285 w2311 w2322 w2333]
                tunnel: w1307 -> [w1380 w1394 w1417 w1429 w1440 w1503 w1525 w1531 w1568 w1571 w1581 w1591 w1607 w1619 w1644 w1660 w1667 w1684 w1691 w1703 w1731 w1758 w1765 w1786 w1795 w1815 w1862 w1873 w1881 w1900 w1918 w1966 w1988 w2036 w2054 w2063 w2107 w2111 w2147 w2152 w2176 w2209 w2235 w2255 w2268 w2316 w2326 w2332]
                tunnel: [w1389 w1395 w1427 w1431 w1452 w1502 w1516 w1533 w1557 w1575 w1589 w1598 w1614 w1626 w1640 w1656 w1669 w1675 w1688 w1700 w1711 w1738 w1771 w1777 w1794 w1817 w1857 w1876 w1882 w1891 w1915 w1957 w1985 w2028 w2046 w2071 w2109 w2128 w2148 w2155 w2174 w2207 w2223 w2240 w2291 w2312 w2321 w2331] -> w1332
                tunnel: [w1380 w1394 w1416 w1429 w1440 w1503 w1525 w1531 w1568 w1571 w1581 w1591 w1607 w1619 w1644 w1660 w1667 w1684 w1691 w1703 w1731 w1758 w1765 w1786 w1795 w1815 w1862 w1873 w1881 w1900 w1918 w1966 w1988 w2036 w2054 w2060 w2107 w2114 w2147 w2152 w2176 w2209 w2235 w2255 w2269 w2316 w2326 w2332] -> w1374
                tunnel: [_ _ _ _ _ _ _ _ _ _ _ _ _ _ _ _ _ _ _ _ _ _ _ _ _ _ _ w1865 _ _ _ _ _ _ _ _ _ _ _ _ _ _ _ _ _ w2305 _ _] -> w1317
                tunnel: [_ _ _ _ _ _ _ _ _ _ _ _ _ _ _ _ _ _ _ _ _ _ _ _ _ _ _ w1864 _ _ _ _ _ _ _ _ _ _ _ _ _ _ _ _ _ w2306 _ _] -> w1316
                tunnel: w1373 -> [w1388 w1392 w1425 w1433 w1465 w1500 w1521 w1547 w1569 w1577 w1588 w1596 w1616 w1628 w1643 w1659 w1664 w1682 w1696 w1708 w1730 w1757 w1770 w1783 w1805 w1827 w1859 w1878 w1887 w1898 w1920 w1964 w1990 w2035 w2040 w2072 w2098 w2130 w2145 w2154 w2156 w2210 w2233 w2253 w2294 w2318 w2328 w2340]
                tunnel: [w1388 w1392 w1425 w1433 w1465 w1499 w1520 w1547 w1569 w1577 w1588 w1596 w1616 w1628 w1643 w1659 w1664 w1682 w1696 w1708 w1730 w1757 w1770 w1783 w1805 w1827 w1858 w1878 w1887 w1898 w1919 w1964 w1989 w2035 w2040 w2072 w2098 w2130 w2145 w2154 w2156 w2210 w2233 w2253 w2294 w2318 w2328 w2340] -> w1372
                tunnel: w1371 -> [w1381 w1393 w1426 w1432 w1460 w1505 w1529 w1548 w1570 w1576 w1583 w1597 w1615 w1627 w1642 w1658 w1665 w1683 w1695 w1707 w1729 w1756 w1769 w1785 w1804 w1828 w1861 w1877 w1890 w1899 w1924 w1965 w1994 w2034 w2053 w2062 w2110 w2132 w2146 w2151 w2175 w2208 w2234 w2254 w2295 w2319 w2329 w2341]
                tunnel: [w1381 w1393 w1426 w1432 w1460 w1505 w1529 w1548 w1570 w1576 w1583 w1597 w1615 w1627 w1642 w1658 w1665 w1683 w1695 w1707 w1729 w1756 w1769 w1785 w1804 w1828 w1861 w1877 w1890 w1899 w1924 w1965 w1994 w2034 w2053 w2061 w2110 w2132 w2146 w2151 w2175 w2208 w2234 w2254 w2295 w2319 w2329 w2341] -> w1370
                tunnel: [_ _ _ _ _ _ _ _ _ _ _ _ _ _ _ _ _ _ _ _ _ _ _ _ _ _ _ _ _ _ _ _ _ _ _ _ _ _ TRUE _ _ _ _ _ _ _ _ _] -> w1335
                tunnel: [_ _ _ _ _ _ _ _ _ _ _ _ _ _ _ _ _ _ _ _ w1713 w1740 _ _ _ _ _ _ _ _ _ _ _ _ _ _ _ _ _ _ _ _ _ _ _ _ _ _] -> w1365
                tunnel: [_ _ _ _ _ _ _ _ _ _ _ _ _ _ _ _ _ _ _ _ w1712 w1739 _ _ _ _ _ _ _ _ _ _ _ _ _ _ _ _ _ _ _ _ _ _ _ _ _ _] -> w1364
                tunnel: w1306 -> [w1386 w1391 w1423 w1430 w1464 w1498 w1524 w1549 w1561 w1578 w1587 w1595 w1610 w1622 w1631 w1647 w1661 w1681 w1690 w1702 w1716 w1743 w1767 w1782 w1803 w1807 w1854 w1872 w1888 w1897 w1917 w1963 w1987 w2033 w2052 w2070 w2108 w2129 w2143 w2153 w2160 w2187 w2232 w2252 w2289 w2317 w2327 w2339]
                tunnel: [w1386 w1391 w1423 w1430 w1464 w1497 w1519 w1532 w1555 w1574 w1586 w1594 w1609 w1621 w1630 w1646 w1661 w1681 w1689 w1701 w1715 w1742 w1767 w1782 w1803 w1806 w1853 w1872 w1888 w1897 w1914 w1963 w1984 w2033 w2051 w2070 w2108 w2129 w2143 w2153 w2160 w2187 w2232 w2252 w2289 w2317 w2327 w2339] -> w1367
                tunnel: w1366 -> [_ _ _ _ _ _ _ _ _ _ _ _ _ _ _ _ _ _ _ _ _ _ _ _ _ _ _ _ _ _ _ _ _ _ w2045 _ _ _ _ _ _ _ _ _ _ _ _ _]
                tunnel: w1363 -> [w1385 _ _ _ w1461 w1492 w1528 w1553 w1566 _ _ w1602 _ _ _ _ _ _ _ _ w1717 w1744 _ _ w1801 w1826 w1852 _ _ _ _ _ w1968 _ w2048 _ _ _ w2141 _ _ _ _ _ w2275 _ _ _]
                tunnel: w1362 -> [w1384 _ _ _ w1462 w1491 w1518 w1552 w1565 _ _ w1601 _ _ _ _ _ _ _ _ w1718 w1745 _ _ w1802 w1825 w1851 _ _ _ _ _ w1967 _ w2047 _ _ _ w2140 _ _ _ _ _ w2274 _ _ _]
                tunnel: [_ _ _ _ _ _ _ _ _ _ _ _ _ _ w1639 w1655 _ _ _ _ w1723 w1750 _ _ w1793 w1813 _ _ _ _ _ _ _ _ _ _ _ _ _ _ _ _ _ _ _ _ _ _] -> w1341
                tunnel: [_ _ _ _ _ _ _ _ _ _ _ _ _ _ w1638 w1654 _ _ _ _ w1722 w1749 _ _ w1792 w1812 _ _ _ _ _ _ _ _ _ _ _ _ _ _ _ _ _ _ _ _ _ _] -> w1322
                tunnel: [_ _ _ _ _ _ _ _ TRUE ("Recording") _ _ _ _ _ _ _ _ _ _ _ _ _ _ _ _ _ _ _ _ _ _ _ _ _ _ _ _ _ _ _ _ _ _ _ _ _ _ _] -> w1338
                tunnel: w1361 -> [_ _ _ _ _ _ _ _ _ _ _ _ _ _ _ _ _ _ _ _ _ _ _ _ _ _ _ _ _ _ _ _ _ _ _ _ _ _ _ _ w2172 w2203 w2230 w2237 _ _ _ _]
                tunnel: [_ _ _ _ _ _ _ _ _ _ _ _ _ _ _ _ _ _ _ _ _ _ _ _ _ _ _ _ _ _ _ _ _ _ _ _ _ _ _ _ w2170 w2202 w2228 w2238 _ _ _ _] -> w1360
                tunnel: w1359 -> [_ _ _ _ w1434 _ _ _ w1562 w1579 w1585 w1593 w1606 w1618 w1635 w1651 w1662 w1680 w1687 w1699 w1724 w1751 w1766 w1781 w1789 w1814 _ _ _ _ _ _ _ _ _ _ _ _ _ _ _ _ _ _ _ _ _ _]
                tunnel: [_ _ _ _ w1434 _ _ w1534 w1562 w1573 w1584 w1592 w1605 w1617 w1635 w1651 w1662 w1680 w1686 w1698 w1724 w1751 w1766 w1781 w1789 w1814 _ _ _ _ _ _ _ _ _ _ _ _ _ _ _ _ _ _ _ _ _ _] -> w1358
                tunnel: [_ _ _ _ _ _ _ _ _ _ _ _ _ _ w1637 w1653 _ _ _ _ w1721 w1748 _ _ w1791 w1811 _ _ _ _ _ _ _ _ _ _ _ _ _ _ _ _ _ _ _ _ _ _] -> w1345
                tunnel: [_ _ _ _ _ _ _ _ _ _ _ _ _ _ w1636 w1652 _ _ _ _ w1720 w1747 _ _ w1790 w1810 _ _ _ _ _ _ _ _ _ _ _ _ _ _ _ _ _ _ _ _ _ _] -> w1346
                tunnel: [_ _ _ _ _ _ _ _ _ _ _ _ _ _ _ _ _ _ _ _ w1714 w1741 _ _ _ _ _ _ _ _ _ _ _ _ _ _ _ _ _ _ _ _ _ _ _ _ _ _] -> w1348
                tunnel: [_ _ "<S,S>" ("string") _ _ _ _ _ w1556 _ _ _ _ _ _ _ _ _ _ _ _ _ _ _ _ _ w1855 _ _ _ w1913 _ w1983 _ w2043 _ _ w2124 _ _ _ _ _ _ _ _ _ _] -> w1311
                tunnel: w1308 -> [_ _ _ _ _ _ _ _ _ _ _ _ _ _ _ _ _ _ _ _ _ _ _ _ _ _ _ _ _ _ _ _ _ _ _ _ _ _ _ _ _ _ _ _ w2280 _ _ _]
                tunnel: w1304 -> [_ _ _ _ _ _ _ _ _ _ _ _ _ _ _ _ _ _ _ _ _ _ _ _ _ _ _ _ _ _ _ _ _ _ _ _ _ w2123 _ _ _ _ _ _ _ _ _ _]
                tunnel: w1303 -> [_ _ _ _ _ _ _ _ _ _ _ _ _ _ _ _ _ _ _ _ _ _ _ _ _ _ _ _ _ _ _ _ _ _ _ _ _ _ _ _ _ _ _ _ _ _ _ _]
                tunnel: w1302 -> [_ _ _ _ _ _ _ _ _ _ _ _ _ _ _ _ _ _ _ _ _ _ _ _ _ _ _ _ _ _ _ _ _ _ _ _ _ _ _ _ _ _ _ _ _ _ _ _]
                tunnel: [_ _ _ _ _ _ _ _ _ _ _ _ _ _ _ _ _ _ _ _ _ _ _ _ _ _ _ _ _ _ _ _ _ _ _ w2064 _ _ _ _ _ _ _ _ _ _ _ _] -> w1301
                tunnel: [_ _ _ _ _ _ _ _ _ _ _ _ _ _ _ _ _ _ _ _ _ _ _ _ _ _ _ _ _ _ _ _ _ _ _ w2069 _ _ _ _ _ _ _ _ _ _ _ _] -> w1300
                tunnel: w1299 -> [_ _ _ _ _ _ _ _ _ _ _ _ _ _ _ _ _ _ _ _ _ _ _ _ _ _ _ _ _ _ _ _ _ _ _ w2068 _ _ _ _ _ _ _ _ _ _ _ _]
                tunnel: w1298 -> [_ _ _ _ _ _ _ _ _ _ _ _ _ _ _ _ _ _ _ _ _ _ _ _ _ _ _ _ _ _ _ _ _ _ _ w2059 _ _ _ _ _ _ _ _ _ _ _ _]
                tunnel: w1291 -> [_ _ w1398 _ _ w1481 w1512 _ _ _ _ _ _ _ _ _ _ _ _ _ _ _ _ _ _ _ w1840 _ _ _ w1903 _ w1973 _ _ _ _ _ _ _ w2167 w2190 _ _ w2260 _ _ _]
                tunnel: w1290 -> [_ _ w1397 _ _ w1482 w1511 _ _ _ _ _ _ _ _ _ _ _ _ _ _ _ _ _ _ _ w1839 _ _ _ w1901 _ w1971 _ _ _ _ _ _ _ w2166 w2189 _ _ w2259 _ _ _]
                tunnel: w1289 -> [_ _ _ _ _ _ _ _ _ _ _ _ _ _ _ _ _ _ _ _ _ _ _ _ _ _ _ _ _ _ _ _ _ _ _ _ _ _ _ _ w2164 w2188 _ _ _ _ _ _]
                tunnel: w1285 -> [_ _ _ _ _ _ _ _ _ _ _ _ _ _ _ _ _ _ _ _ w1710 w1737 _ _ _ _ _ _ _ _ _ _ _ _ _ _ _ _ _ _ _ _ _ _ _ _ _ _]
                frame "Start1", Default {
                  w1383 = FALSE ("SelectionState")
                  n292 = xnode "Read/Write Control"("FPGA VI Reference In"=w1385, "error in"=w1384, "SelectionState"=w1383, "LR_reward_Laser_l1"=w1383, "LR_wrong_Laser_l1"=w1383, "LR_reward_Event_l1"=w1383, "LR_wrong_Event_l1"=w1383, "Left(F)_or_Right(T)"=w1383, "SelectionState"=w1383, "LR_reward_Laser_l2"=w1383, "LR_wrong_laser_l2"=w1383, "LR_reward_Event_l2"=w1383, "LR_wrong_Event_l2"=w1383, "LC_Event_l1"=w1383, "LC_Laser_l1"=w1383, "LC_Laser_l2"=w1383, "LC_Event_l2"=w1383, "CueLed_Event"=w1383) -> ("error out"=w1382:errorcluster)  [unwired: 1 out]
                  n293 = local write "error out"(w1382) -> ()
                }
                frame "Start2" {
                }
                frame "Start3" {
                  w1401 = u16 3 ("element")
                  w1399 = u16 0 ("element")
                  w1413 = u16 0 ("new element/subarray")
                  w1418 = 0.0 ("BTPR_avg_L")
                  w1421 = FALSE ("SolenoidReward")
                  w1419 = u16 0 ("BTPR_block")
                  w1422 = u16 0 ("nRewards_cur")
                  # "Goal:\nPrepare dataCurrent"
                  n294 = call "BRig_dataExp_FreeReward_c_L.vi"() -> ("output_FreeReward_c_L"=w1415:i32)  [unwired: 11 in]
                  n295 = call "BRig_dataExp_FreeReward_c_R.vi"() -> ("output_FreeReward_c_R"=w1414:i32)  [unwired: 11 in]
                  n296 = local write "nRewards_cur"(w1422) -> ()
                  n297 = local write "nRewards_total"(w1422) -> ()
                  n298 = local write "nRewards_Left"(w1422) -> ()
                  n299 = local write "nRewards_Right"(w1422) -> ()
                  n300 = local write "BUR_target"(w1422) -> ()
                  n301 = local write "TpB_target"(w1422) -> ()
                  n302 = local write "iBlock"(w1422) -> ()
                  n303 = local write "iTrial"(w1422) -> ()
                  n304 = local write "nTrial"(w1422) -> ()
                  n305 = local write "SolenoidReward"(w1421) -> ()
                  n306 = local write "allReward_L"(w1421) -> ()
                  n307 = local write "allReward_R"(w1421) -> ()
                  n308 = Replace Array Subset(array=w1417, new element #1=w1413, index #1=w1415, new element #2=w1413, index #2=w1414) -> (w1416:u16[])
                  n309 = call "BRig_dataRT_stats__T2R_cur.vi"() -> ("output_T2R_cur"=w1412:i32)  [unwired: 11 in]
                  n310 = call "BRig_dataRT_stats__BTPR_cur.vi"() -> ("output_BTPR_cur"=w1411:i32)  [unwired: 11 in]
                  n311 = call "BRig_dataRT_stats__T2R_avg_L.vi"() -> ("output_T2R_avg_L__x100"=w1406:i32)  [unwired: 11 in]
                  n312 = call "BRig_dataRT_stats__T2R_avg_R.vi"() -> ("output_T2R_avg_R__x100"=w1405:i32)  [unwired: 11 in]
                  n313 = call "BRig_dataRT_stats__BTPR_avg_L.vi"() -> ("output_BTPR_avg_L__x100"=w1410:i32)  [unwired: 11 in]
                  n314 = call "BRig_dataRT_stats__BTPR_avg_R.vi"() -> ("output_BTPR_avg_R__x100"=w1402:i32)  [unwired: 11 in]
                  n315 = local write "FreeReward_c_L"(w1413) -> ()
                  n316 = local write "FreeReward_c_R"(w1413) -> ()
                  n317 = local write "BTPR_block"(w1419) -> ()
                  n318 = local write "T2R_block"(w1419) -> ()
                  n319 = local write "BTPR_avg_L"(w1418) -> ()
                  n320 = local write "BTPR_avg_R"(w1418) -> ()
                  n321 = local write "T2R_avg_L"(w1418) -> ()
                  n322 = local write "T2R_avg_R"(w1418) -> ()
                  n323 = To Unsigned Word Integer(number=w1406) -> (unsigned 16bit integer=w1407:u16)
                  n324 = To Unsigned Word Integer(number=w1412) -> (unsigned 16bit integer=w1409:u16)
                  n325 = To Unsigned Word Integer(number=w1405) -> (unsigned 16bit integer=w1404:u16)
                  n326 = To Unsigned Word Integer(number=w1411) -> (unsigned 16bit integer=w1408:u16)
                  n327 = To Unsigned Word Integer(number=w1410) -> (unsigned 16bit integer=w1403:u16)
                  n328 = To Unsigned Word Integer(number=w1402) -> (unsigned 16bit integer=w1400:u16)
                  n329 = Build Array(w1401, w1409, w1399, w1401, w1408, w1399, w1401, w1407, w1399, w1401, w1404, w1399, w1401, w1403, w1399, w1401, w1400, w1399) -> (w1396:u16[])
                  n330 = RT FIFO Write(0:w1398, 1:w1396, 3:w1397) -> ()  [unwired: 2 in, 4 out]
                }
                frame "saveSettings1" {
                }
                frame "setSettings_Laser" {
                  n331 = call "BRig_dataExp_LED_baseline_Cue.vi"() -> ("output_LED_baseline_Cue"=w1449:i32)  [unwired: 11 in]
                  n332 = call "BRig_dataExp_LED_baseline_l1.vi"() -> ("output_LED_baseline_l1"=w1450:i32)  [unwired: 11 in]
                  n333 = call "BRig_dataExp_LED_baseline_l2.vi"() -> ("output_LED_baseline_l2"=w1448:i32)  [unwired: 11 in]
                  n334 = call "BRig_dataExp_I_anySelect.vi"() -> ("output_I_anySelect"=w1442:i32)  [unwired: 11 in]
                  n335 = call "BRig_dataExp_I_trialUntilReward.vi"() -> ("output_I_trialUntilReward"=w1441:i32)  [unwired: 11 in]
                  n336 = local read "FPGA_count2ms"() -> (w1459:dbl)
                  n337 = call "BRig_RT__Case_Exp__State_setLaserSettings.vi"("input_FPGA_count2ms"=w1459, "input_dataExp"=w1440, "input_dataLC"=w1460) -> ("output_LR_nTotal_l1"=w1458:u32, "output_LR_nTotal_l2"=w1457:u32, "output_LR_reward_nDelay_l1"=w1456:u32, "output_LR_wrong_nDelay_l1"=w1455:u32, "output_LR_reward_nDelay_l2"=w1454:u32, "output_LR_wrong_nDelay_l2"=w1453:u32)  [unwired: 11 in]
                  n338 = Index Array(array=w1440, index #1=w1449, index #2=w1450, index #3=w1448, index #4=w1442, index #5=w1441) -> (element #1=w1447:u16, element #2=w1446:u16, element #3=w1445:u16, element #4=w1444:u16, element #5=w1443:u16)
                  n339 = Not Equal To 0?(x=w1446) -> (x != 0?=w1438:bool)
                  n340 = Not Equal To 0?(x=w1444) -> (x != 0?=w1436:bool)
                  n341 = Not Equal To 0?(x=w1447) -> (x != 0?=w1439:bool)
                  n342 = Not Equal To 0?(x=w1445) -> (x != 0?=w1437:bool)
                  n343 = Not Equal To 0?(x=w1443) -> (x != 0?=w1435:bool)
                  n344 = xnode "Read/Write Control"("FPGA VI Reference In"=w1461, "error in"=w1462, "LR_reward_nTotal_l1"=w1458, "LR_wrong_nTotal_l1"=w1458, "LR_reward_nTotal_l2"=w1457, "LR_wrong_nTotal_l2"=w1457, "LR_reward_nDelay_l1"=w1456, "LR_wrong_nDelay_l1"=w1455, "LR_reward_nDelay_l2"=w1454, "LR_wrong_nDelay_l2"=w1453, "CueLed_Baseline"=w1439, "L1Led_Baseline"=w1438, "L2Led_Baseline"=w1437, "I_allReward"=w1436, "ignoreWrong"=w1435) -> ("error out"=→"error out":errorcluster)  [unwired: 1 out]
                }
                frame "initBlock" {
                  w1466 = u16 0 ("element")
                  w1468 = u16 3
                  w1484 = u16 0 ("BTPR_block")
                  n345 = local write "nRewards_cur"(u16 0 ("nRewards_cur")) -> ()
                  n346 = local write "BTPR_block"(w1484) -> ()
                  n347 = local write "T2R_block"(w1484) -> ()
                  n348 = call "BRig_RT__Case_Exp__State_initBlock.vi"("input_dataCurrent"=w1504, "input_dataExp"=w1503, "input_dataBlock"=w1500, "input_dataTrial"=w1498) -> ("output_iSpout"=w1489:u16, "output_speaker_amp_R"=w1493:u16, "output_iBlock"=w1473:u16, "output_speaker_freq_R"=w1494:u8, "output_BUR_target"=w1474:u16, "output_speaker_amp_L"=w1495:u16, "output_TpB_target"=w1475:u16, "output_speaker_freq_L"=w1496:u8, "output_dataCurrent"=w1502:u16[], "output_dataBlock"=w1499:u16[][], "output_dataTrial"=w1497:u16[][])  [unwired: 5 in]
                  n349 = Type Cast(type=enum16{"Left", "Right"}."Left", x=w1489) -> (*(type *) &x=w1486:enum16{"Left", "Right"})
                  n350 = Not Equal To 0?(x=w1489) -> (x != 0?=w1485:bool)
                  n351 = call "BRig_dataRT_stats__TpB_target.vi"() -> ("output_TpB_target"=w1476:i32)  [unwired: 11 in]
                  n352 = call "BRig_dataRT_stats__BUR_target.vi"() -> ("output_BUR_target"=w1477:i32)  [unwired: 11 in]
                  n353 = call "BRig_dataRT_stats__iBlock.vi"() -> ("output_iBlock"=w1478:i32)  [unwired: 11 in]
                  n354 = call "BRig_dataRT_stats__T2R_cur.vi"() -> ("output_T2R_cur"=w1471:i32)  [unwired: 11 in]
                  n355 = call "BRig_dataRT_stats__BTPR_cur.vi"() -> ("output_BTPR_cur"=w1470:i32)  [unwired: 11 in]
                  n356 = local write "cSpout"(w1486) -> ()
                  n357 = xnode "Read/Write Control"("FPGA VI Reference In"=w1492, "error in"=w1491, "Left(F)_or_Right(T)"=w1485, "audioFreq_L_kHz"=w1496, "audioAmp_L"=w1495, "audioFreq_R_kHz"=w1494, "audioAmp_R"=w1493) -> ("error out"=w1490:errorcluster)  [unwired: 1 out]
                  n358 = To Unsigned Word Integer(number=w1471) -> (unsigned 16bit integer=w1469:u16)
                  n359 = To Unsigned Word Integer(number=w1476) -> (unsigned 16bit integer=w1483:u16)
                  n360 = To Unsigned Word Integer(number=w1477) -> (unsigned 16bit integer=w1480:u16)
                  n361 = To Unsigned Word Integer(number=w1478) -> (unsigned 16bit integer=w1479:u16)
                  n362 = To Unsigned Word Integer(number=w1470) -> (unsigned 16bit integer=w1467:u16)
                  n363 = local write "error out"(w1490) -> ()
                  n364 = local write "iBlock"(w1473) -> ()
                  n365 = local write "BUR_target"(w1474) -> ()
                  n366 = local write "TpB_target"(w1475) -> ()
                  n367 = Build Array(w1468, w1483, w1475, w1468, w1480, w1474, w1468, w1479, w1473, w1468, w1469, w1466, w1468, w1467, w1466) -> (w1472:u16[])
                  n368 = RT FIFO Write(0:w1481, 1:w1472, 3:w1482) -> ()  [unwired: 2 in, 4 out]
                }
                frame "initTrial" {
                  w1508 = u16 3
                  n369 = xnode "Read/Write Control"("FPGA VI Reference In"=w1528, "error in"=w1518, "SelectionState"=FALSE) -> ("error out"=w1527:errorcluster)  [unwired: 1 out]
                  n370 = call "BRig_RT__Case_Exp__State_initTrial__v3.vi"("input_dataCurrent"=w1517, "input_dataBlock"=w1521, "input_dataTrial"=w1524, "input_dataExp"=w1525) -> ("output_iTrial"=w1506:u16, "output_nTrial"=w1507:u16, "output_SolenoidReward"=w1523:bool, "output_dataCurrent"=w1516:u16[], "output_dataBlock"=w1520:u16[][], "output_dataTrial"=w1519:u16[][])  [unwired: 6 in]
                  n371 = call "BRig_dataRT_stats__nTrial.vi"() -> ("output_nTrial"=w1510:i32)  [unwired: 11 in]
                  n372 = call "BRig_dataRT_stats__iTrial.vi"() -> ("output_iTrial"=w1509:i32)  [unwired: 11 in]
                  n373 = local write "iTrial"(w1506) -> ()
                  n374 = local write "nTrial"(w1507) -> ()
                  n375 = local write "SolenoidReward"(w1523) -> ()
                  n376 = To Unsigned Word Integer(number=w1510) -> (unsigned 16bit integer=w1515:u16)
                  n377 = To Unsigned Word Integer(number=w1509) -> (unsigned 16bit integer=w1513:u16)
                  n378 = local write "error out"(w1527) -> ()
                  n379 = Build Array(w1508, w1515, w1507, w1508, w1513, w1506) -> (w1514:u16[])
                  n380 = RT FIFO Write(0:w1512, 1:w1514, 3:w1511) -> ()  [unwired: 2 in, 4 out]
                }
                frame "initTrial2" {
                  n381 = call "BRig_RT__Case_Exp__State_initTrial2__v4.vi"("input_dataCurrent"=w1530, "input_dataTrial"=w1549, "input_dataExp"=w1531, "input_dataBlock"=w1547, "input_dataLC"=w1548) -> ("output_L_Wrong_Laser_l2"=w1539:bool, "output_L_Wrong_Event_l2"=w1540:bool, "output_L_Power_l1"=w1538:dbl, "output_L_Reward_Laser_l2"=w1541:bool, "output_L_Power_l2"=w1537:dbl, "output_L_Reward_Event_l2"=w1542:bool, "output_dataCurrent"=w1533:u16[], "output_dataTrial"=w1532:u16[][], "output_L_Reward_Event_l1"=w1546:bool, "output_L_Reward_Laser_l1"=w1545:bool, "output_L_Wrong_Event_l1"=w1544:bool, "output_L_Wrong_Laser_l1"=w1543:bool)  [unwired: 3 in]
                  n382 = local write "L_Power_l1"(w1538) -> ()
                  n383 = call "myRIO__convert__Voltage_to_FPGAvalue.vi"("input_voltage"=w1538) -> ("output_PortC"=w1535:i16)  [unwired: 9 in, 1 out]
                  n384 = local write "L_Power_l2"(w1537) -> ()
                  n385 = call "myRIO__convert__Voltage_to_FPGAvalue.vi"("input_voltage"=w1537) -> ("output_PortC"=w1536:i16)  [unwired: 9 in, 1 out]
                  n386 = xnode "Read/Write Control"("FPGA VI Reference In"=w1553, "error in"=w1552, "AnaOut_0"=w1535, "AnaOut_1"=w1536, "LR_reward_Event_l1"=w1546, "LR_reward_Laser_l1"=w1545, "LR_wrong_Event_l1"=w1544, "LR_wrong_Laser_l1"=w1543, "LR_reward_Event_l2"=w1542, "LR_reward_Laser_l2"=w1541, "LR_wrong_Event_l2"=w1540, "LR_wrong_laser_l2"=w1539) -> ("error out"=w1550:errorcluster)  [unwired: 1 out]
                  n387 = local write "error out"(w1550) -> ()
                  n388 = call "BRig_arrTrig_init.vi"() -> ("output_arrTrig"=w1534:bool[])  [unwired: 11 in]
                }
                frame "initTrial4" {
                  # "resetOccurrence?\ndataAnalog"
                  n389 = local read "FPGA_count2ms"() -> (w1558:dbl)
                  n390 = local read "lick_Rising(F)_or_Falling(T)"() -> (w1554:bool)
                  n391 = local read "Recording"() -> (w1560:bool)
                  n392 = call "BRig_RT_comm_tcp_write_RTwrite__RunState_Trial_start.vi"("input_dataCurrent"=w1557) -> ("output_strCmd"=w1556:string)  [unwired: 10 in]
                  n393 = call "BRig_RT__Case_Exp__State_initTrial4.vi"("input_Recording"=w1560, "input_FPGA_count2ms"=w1558, "input_dataTrial"=w1561) -> ("output_Solenoid_nTotal"=w1559:u32, "output_dataTrial"=w1555:u16[][])  [unwired: 7 in]
                  n394 = xnode "Read/Write Control"("FPGA VI Reference In"=w1566, "error in"=w1565, "Solenoid_nTotal_L"=w1559, "Solenoid_nTotal_R"=w1559, "A6_Act"=w1560, "Rising(F)_or_Falling(T)"=w1554) -> ("error out"=w1564:errorcluster)  [unwired: 1 out]
                  n395 = local write "error out"(w1564) -> ()
                }
                frame "initTrial_LC_ENL1" {
                  n396 = call "BRig_RT__Case_Exp__State_initTrial__LC_ENL__v4.vi"("input_arrTrig"=w1579, "input_dataTrial"=w1578, "input_dataExp"=w1571, "input_dataLC"=w1576, "input_dataCurrent"=w1572) -> ("output_dataTrial"=w1574:u16[][], "output_dataCurrent"=w1575:u16[], "output_arrTrig"=w1573:bool[])  [unwired: 4 in]
                }
                frame "initTrial_LC_Cue1" {
                  n397 = call "BRig_RT__Case_Exp__State_initTrial__LC_Cue__v4.vi"("input_arrTrig"=w1585, "input_dataTrial"=w1587, "input_dataExp"=w1581, "input_dataLC"=w1583, "input_dataCurrent"=w1582) -> ("output_dataTrial"=w1586:u16[][], "output_dataCurrent"=w1589:u16[], "output_arrTrig"=w1584:bool[])  [unwired: 4 in]
                }
                frame "initTrial_LC_Sel" {
                  n398 = call "BRig_RT__Case_Exp__State_initTrial__LC_Select__v4.vi"("input_arrTrig"=w1593, "input_dataTrial"=w1595, "input_dataExp"=w1591, "input_dataLC"=w1597, "input_dataCurrent"=w1599) -> ("output_dataTrial"=w1594:u16[][], "output_dataCurrent"=w1598:u16[], "output_arrTrig"=w1592:bool[])  [unwired: 4 in]
                  n399 = xnode "Read/Write Control"("FPGA VI Reference In"=w1602, "error in"=w1601, "A6_Act"=FALSE) -> ("error out"=w1603:errorcluster)  [unwired: 1 out]
                  n400 = local write "error out"(w1603) -> ()
                }
                frame "ENL1_pre" {
                  n401 = call "BRig_RT__Case_Exp__State_ENLPre__v4.vi"("input_arrTrig"=w1606, "input_ENL2"=FALSE, "input_I_lick"=w1613, "input_dataExp"=w1607, "input_dataTrial"=w1610, "input_dataCurrent"=w1611) -> ("output_arrTrig"=w1605:bool[], "output_dataTrial"=w1609:u16[][], "output_dataCurrent"=w1614:u16[], "output_state"=w1612:T2)  [unwired: 2 in]
                }
                frame "ENL2_pre" {
                  n402 = call "BRig_RT__Case_Exp__State_ENLPre__v4.vi"("input_arrTrig"=w1618, "input_ENL2"=TRUE, "input_I_lick"=w1625, "input_dataExp"=w1619, "input_dataTrial"=w1622, "input_dataCurrent"=w1623) -> ("output_arrTrig"=w1617:bool[], "output_dataTrial"=w1621:u16[][], "output_dataCurrent"=w1626:u16[], "output_state"=w1624:T2)  [unwired: 2 in]
                }
                frame "ENL1" {
                  n403 = call "BRig_RT__Case_Exp__State_ENL__v3.vi"("input_dataCurrent"=w1641, "input_dataTrial"=w1631, "input_ENL2"=FALSE, "input_arrTrig"=w1635, "input_state"=w1634, "I_lick"=w1633) -> ("output_l2_laserOn"=w1636:bool, "output_l2_laserEvent"=w1637:bool, "output_l1_laserOn"=w1638:bool, "output_state"=w1632:T2, "output_l1_laserEvent"=w1639:bool, "output_dataCurrent"=w1640:u16[], "output_dataTrial"=w1630:u16[][])  [unwired: 7 in]
                }
                frame "ENL2" {
                  n404 = call "BRig_RT__Case_Exp__State_ENL__v3.vi"("input_dataCurrent"=w1657, "input_dataTrial"=w1647, "input_ENL2"=TRUE, "input_arrTrig"=w1651, "input_state"=w1650, "I_lick"=w1649) -> ("output_l2_laserOn"=w1652:bool, "output_l2_laserEvent"=w1653:bool, "output_l1_laserOn"=w1654:bool, "output_state"=w1648:T2, "output_l1_laserEvent"=w1655:bool, "output_dataCurrent"=w1656:u16[], "output_dataTrial"=w1646:u16[][])  [unwired: 7 in]
                }
                frame "ENL1Penalty_pre" {
                  n405 = call "BRig_dataCurrent_c_generic.vi"() -> ("output_count_generic"=w1673:i32)  [unwired: 11 in]
                  n406 = call "BRig_dataCurrent_T_generic.vi"() -> ("output_T_generic"=w1671:i32)  [unwired: 11 in]
                  n407 = call "BRig_dataExp_T_ENLPenalty.vi"() -> ("output_ENL_penalty"=w1666:i32)  [unwired: 11 in]
                  n408 = Index Array(array=w1667, index=w1666) -> (element=w1670:u16)
                  n409 = Replace Array Subset(array=w1668, new element #1=u16 0 ("new element/subarray"), index #1=w1673, new element #2=w1670, index #2=w1671) -> (w1669:u16[])
                }
                frame "ENL1Penalty" {
                  n410 = call "BRig_RT__Case_Exp__generic__incrementCountTilThreshold.vi"("input_dataCurrent"=w1676) -> ("output_dataCurrent"=w1675:u16[], "output_underThreshold"=w1674:bool)  [unwired: 9 in]
                  n411 = Select(t=w1679, s=w1674, f=myRIO_BRig_RT__Case_Exp_stateList."ENL1_pre" ("Enum")) -> (s? t:f=w1677:T2)
                }
                frame "Cue1_pre" {
                  n412 = call "BRig_RT__Case_Exp__State_CuePre__v3.vi"("input_dataCurrent"=w1694, "input_dataTrial"=w1690, "input_Cue2"=FALSE ("input_ENL2"), "input_I_lick"=w1693, "input_dataExp"=w1691, "input_arrTrig"=w1687) -> ("output_state"=w1692:T2, "output_arrTrig"=w1686:bool[], "output_dataCurrent"=w1688:u16[], "output_dataTrial"=w1689:u16[][])  [unwired: 10 in]
                }
                frame "Cue2_pre" {
                  n413 = call "BRig_RT__Case_Exp__State_CuePre__v3.vi"("input_dataCurrent"=w1706, "input_dataTrial"=w1702, "input_Cue2"=TRUE ("input_ENL2"), "input_I_lick"=w1705, "input_dataExp"=w1703, "input_arrTrig"=w1699) -> ("output_state"=w1704:T2, "output_arrTrig"=w1698:bool[], "output_dataCurrent"=w1700:u16[], "output_dataTrial"=w1701:u16[][])  [unwired: 10 in]
                }
                frame "Cue1" {
                  n414 = call "BRig_RT__Case_Exp__State_Cue__v3.vi"("input_dataCurrent"=w1728, "input_dataTrial"=w1716, "input_dataExp"=w1710, "input_Cue2"=FALSE, "input_arrTrig"=w1724, "input_state"=w1726, "I_lick"=w1727) -> ("output_l2_laserOn"=w1720:bool, "output_l2_laserEvent"=w1721:bool, "output_SelectionState"=w1719:bool, "output_l1_laserOn"=w1722:bool, "output_state"=w1725:T2, "output_l1_laserEvent"=w1723:bool, "output_dataCurrent"=w1711:u16[], "output_dataTrial"=w1715:u16[][], "output_CueLed"=w1714:bool, "output_Audio_L"=w1713:bool, "output_Audio_R"=w1712:bool)  [unwired: 2 in]
                  n415 = case shown="True" w1719 {
                    selector: w1719 -> [_ w1734]
                    tunnel: w1718 -> [_ w1733]
                    tunnel: w1717 -> [_ w1732]
                    frame False {
                    }
                    frame True {
                      n416 = xnode "Read/Write Control"("FPGA VI Reference In"=w1732, "error in"=w1733, "SelectionState"=w1734) -> ("error out"=w1735:errorcluster)  [unwired: 1 out]
                      n417 = local write "error out"(w1735) -> ()
                    }
                  }
                }
                frame "Cue2" {
                  n418 = call "BRig_RT__Case_Exp__State_Cue__v3.vi"("input_dataCurrent"=w1755, "input_dataTrial"=w1743, "input_dataExp"=w1737, "input_Cue2"=TRUE, "input_arrTrig"=w1751, "input_state"=w1753, "I_lick"=w1754) -> ("output_l2_laserOn"=w1747:bool, "output_l2_laserEvent"=w1748:bool, "output_SelectionState"=w1746:bool, "output_l1_laserOn"=w1749:bool, "output_state"=w1752:T2, "output_l1_laserEvent"=w1750:bool, "output_dataCurrent"=w1738:u16[], "output_dataTrial"=w1742:u16[][], "output_CueLed"=w1741:bool, "output_Audio_L"=w1740:bool, "output_Audio_R"=w1739:bool)  [unwired: 2 in]
                  n419 = case shown="True" w1746 {
                    selector: w1746 -> [_ w1761]
                    tunnel: w1745 -> [_ w1760]
                    tunnel: w1744 -> [_ w1759]
                    frame False {
                    }
                    frame True {
                      n420 = xnode "Read/Write Control"("FPGA VI Reference In"=w1759, "error in"=w1760, "SelectionState"=w1761) -> ("error out"=w1762:errorcluster)  [unwired: 1 out]
                      n421 = local write "error out"(w1762) -> ()
                    }
                  }
                }
                frame "Cue1Penalty_pre" {
                  n422 = call "BRig_dataCurrent_c_generic.vi"() -> ("output_count_generic"=w1775:i32)  [unwired: 11 in]
                  n423 = call "BRig_dataCurrent_T_generic.vi"() -> ("output_T_generic"=w1773:i32)  [unwired: 11 in]
                  n424 = call "BRig_dataExp_T_CuePenalty.vi"() -> ("output_T_CuePenalty"=w1764:i32)  [unwired: 11 in]
                  n425 = Index Array(array=w1765, index=w1764) -> (element=w1763:u16)
                  n426 = Replace Array Subset(array=w1772, new element #1=u16 0 ("new element/subarray"), index #1=w1775, new element #2=w1763, index #2=w1773) -> (w1771:u16[])
                }
                frame "Cue1Penalty" {
                  n427 = call "BRig_RT__Case_Exp__generic__incrementCountTilThreshold.vi"("input_dataCurrent"=w1778) -> ("output_dataCurrent"=w1777:u16[], "output_underThreshold"=w1776:bool)  [unwired: 9 in]
                  n428 = Select(t=w1779, s=w1776, f=myRIO_BRig_RT__Case_Exp_stateList."ENL1_pre" ("Enum")) -> (s? t:f=w1780:T2)
                }
                frame "Selection_pre" {
                  n429 = xnode "Read/Write Control"("FPGA VI Reference In"=w1801, "error in"=w1802) -> ("error out"=w1800:errorcluster, "SelectReward"=w1797:bool, "SelectWrong"=w1798:bool)  [unwired: 1 out]
                  n430 = call "BRig_RT__Case_Exp__State_SelectPre.vi"("input_dataCurrent"=w1799, "input_SelectWrong"=w1798, "input_SelectReward"=w1797, "input_dataExp"=w1795, "input_LickL"=w1788, "input_LickR"=w1787, "input_arrTrig"=w1789) -> ("output_state"=w1796:T2, "output_dataCurrent"=w1794:u16[], "output_l1_laserEvent"=w1793:bool, "output_l1_laserOn"=w1792:bool, "output_l2_laserOn"=w1790:bool, "output_l2_laserEvent"=w1791:bool)  [unwired: 3 in]
                  n431 = local write "error out"(w1800) -> ()
                }
                frame "Selection" {
                  n432 = xnode "Read/Write Control"("FPGA VI Reference In"=w1826, "error in"=w1825) -> ("error out"=w1824:errorcluster, "SelectReward"=w1821:bool, "SelectWrong"=w1822:bool)  [unwired: 1 out]
                  n433 = call "BRig_RT__Case_Exp__State_Selection.vi"("input_state"=w1823, "input_dataCurrent"=w1816, "input_dataTrial"=w1807, "input_dataExp"=w1815, "input_arrTrig"=w1814, "input_FPGA_SelectWrong"=w1822, "input_FPGA_SelectReward"=w1821, "input_LickR"=w1820, "input_LickL"=w1819) -> ("output_LC_Laser_l2"=w1810:bool, "output_LC_Event_l2"=w1811:bool, "output_LC_Laser_l1"=w1812:bool, "output_LC_Event_l1"=w1813:bool, "output_state"=w1818:T2, "output_dataCurrent"=w1817:u16[], "output_dataTrial"=w1806:u16[][], "output_anySelect_L"=w1808:bool, "output_anySelect_R"=w1809:bool)  [unwired: 2 in]
                  n434 = local write "allReward_L"(w1808) -> ()
                  n435 = local write "allReward_R"(w1809) -> ()
                  n436 = local write "error out"(w1824) -> ()
                }
                frame "SelectReward_pre" {
                  w1836 = u16 3
                  n437 = call "BRig_dataRT_stats__nReward_left.vi"() -> ("output_nReward_left"=w1833:i32)  [unwired: 11 in]
                  n438 = call "BRig_dataRT_stats__nReward_right.vi"() -> ("output_nReward_right"=w1834:i32)  [unwired: 11 in]
                  n439 = call "BRig_dataRT_stats__nReward_cur.vi"() -> ("output_nReward_cur"=w1835:i32)  [unwired: 11 in]
                  n440 = call "BRig_dataRT_stats__nReward.vi"() -> ("output_nReward"=w1838:i32)  [unwired: 11 in]
                  n441 = call "BRig_RT__Case_Exp__State_RewardPre.vi"("input_dataCurrent"=w1860, "input_dataBlock"=w1859, "input_dataTrial"=w1854) -> ("output_T_Reward"=w1850:u16, "output_c_nReward_total_R"=w1829:u16, "output_c_nReward_total_L"=w1830:u16, "output_dataCurrent"=w1857:u16[], "output_dataBlock"=w1858:u16[][], "output_c_nReward_total"=w1832:u16, "output_nReward"=w1831:u16, "output_dataTrial"=w1853:u16[][])  [unwired: 5 in]
                  n442 = local read "FPGA_count2ms"() -> (w1849:dbl)
                  n443 = local write "nRewards_cur"(w1831) -> ()
                  n444 = local write "nRewards_total"(w1832) -> ()
                  n445 = To Unsigned Word Integer(number=w1833) -> (unsigned 16bit integer=w1844:u16)
                  n446 = To Unsigned Word Integer(number=w1834) -> (unsigned 16bit integer=w1842:u16)
                  n447 = To Unsigned Word Integer(number=w1835) -> (unsigned 16bit integer=w1841:u16)
                  n448 = To Unsigned Word Integer(number=w1838) -> (unsigned 16bit integer=w1837:u16)
                  n449 = local write "nRewards_Right"(w1829) -> ()
                  n450 = local write "nRewards_Left"(w1830) -> ()
                  n451 = To Double Precision Float(number=w1850) -> (double precision float=w1848:dbl)
                  n452 = Multiply(x=w1849, y=w1848) -> (x*y=w1846:dbl)
                  n453 = Round Toward +Infinity(x=w1846) -> (ceil(x): smallest int >= x=w1847:dbl)
                  n454 = Build Array(w1836, w1844, w1830, w1836, w1842, w1829, w1836, w1841, w1831, w1836, w1837, w1832) -> (w1843:u16[])
                  n455 = To Unsigned Long Integer(number=w1847) -> (unsigned 32bit integer=w1845:u32)
                  n456 = call "BRig_RT_comm_tcp_write_RTwrite__RunState_Trial_selResult.vi"("input_dataTrial"=w1853, "iReward_or_iError"=TRUE, "input_dataCurrent"=w1857) -> ("output_strCmd"=w1855:string)  [unwired: 8 in]
                  n457 = RT FIFO Write(0:w1840, 1:w1843, 3:w1839) -> ()  [unwired: 2 in, 4 out]
                  n458 = xnode "Read/Write Control"("FPGA VI Reference In"=w1852, "error in"=w1851, "Solenoid_nTotal_L"=w1845, "Solenoid_nTotal_R"=w1845) -> ()  [unwired: 2 out]
                }
                frame "SelectReward" {
                  n459 = call "BRig_dataCurrent_c_generic.vi"() -> ("output_count_generic"=w1870:i32)  [unwired: 11 in]
                  n460 = call "BRig_RT__Case_Exp__State_Reward.vi"("input_dataCurrent"=w1871, "input_state"=w1875, "input_dataExp"=w1873) -> ("output_state"=w1874:T2, "output_dataCurrent"=w1876:u16[], "output__L"=w1868:bool, "output__R"=w1867:bool)  [unwired: 9 in]
                  n461 = Index Array(array=w1871, index=w1870) -> (element=w1869:u16)
                  n462 = Equal To 0?(x=w1869) -> (x = 0?=w1866:bool)
                  n463 = And(x=w1868, y=w1866) -> (x .and. y?=w1865:bool)
                  n464 = And(x=w1867, y=w1866) -> (x .and. y?=w1864:bool)
                }
                frame "SelectRewardPost_pre" {
                  n465 = call "BRig_dataExp_T_RewardPost.vi"() -> ("output_T_RewardPost"=w1880:i32)  [unwired: 11 in]
                  n466 = call "BRig_dataCurrent_c_generic.vi"() -> ("output_count_generic"=w1886:i32)  [unwired: 11 in]
                  n467 = call "BRig_dataCurrent_T_generic.vi"() -> ("output_T_generic"=w1885:i32)  [unwired: 11 in]
                  n468 = Index Array(array=w1881, index=w1880) -> (element=w1879:u16)
                  n469 = Replace Array Subset(array=w1883, new element #1=u16 0 ("new element/subarray"), index #1=w1886, new element #2=w1879, index #2=w1885) -> (w1882:u16[])
                }
                frame "SelectRewardPost" {
                  n470 = call "BRig_RT__Case_Exp__generic__incrementCountTilThreshold.vi"("input_dataCurrent"=w1893) -> ("output_dataCurrent"=w1891:u16[], "output_underThreshold"=w1892:bool)  [unwired: 9 in]
                  n471 = Select(t=w1895, s=w1892, f=myRIO_BRig_RT__Case_Exp_stateList."endTrial1" ("Enum")) -> (s? t:f=w1894:T2)
                }
                frame "SelectWrong_pre" {
                  n472 = call "BRig_RT__Case_Exp__State_WrongOrTimeout_Pre__v4.vi"("input_dataCurrent"=w1922, "input_WorTO"=FALSE, "input_dataBlock"=w1920, "input_dataTrial"=w1917, "input_dataExp"=w1918) -> ("output_T2R"=w1912:bool, "output_T2R_or_BTPR"=w1904:u16, "output_dataCurrent"=w1915:u16[], "output_dataBlock"=w1919:u16[][], "output_dataTrial"=w1914:u16[][], "output_BTPRavg"=w1908:dbl, "output_T2Ravg"=w1909:dbl, "output_R(F)_or_L(T)"=w1910:bool, "output_haveNewAvg"=w1911:bool)  [unwired: 1 in, 1 out]
                  n473 = case shown="False" w1912 {
                    tunnel: w1904 -> [w1954 w1956]
                    tunnel: [w1953 w1955] -> w1907
                    frame False {
                      n474 = call "BRig_dataRT_stats__BTPR_cur.vi"() -> ("output_BTPR_cur"=w1953:i32)  [unwired: 11 in]
                      n475 = local write "BTPR_block"(w1954) -> ()
                    }
                    frame True {
                      n476 = call "BRig_dataRT_stats__T2R_cur.vi"() -> ("output_T2R_cur"=w1955:i32)  [unwired: 11 in]
                      n477 = local write "T2R_block"(w1956) -> ()
                    }
                  }
                  n478 = To Unsigned Word Integer(number=w1907) -> (unsigned 16bit integer=w1905:u16)
                  n479 = case shown="True" w1911 {
                    tunnel: w1910 -> [_ w1944]
                    tunnel: w1909 -> [_ w1934]
                    tunnel: w1908 -> [_ w1930]
                    tunnel: u16 3 -> [w1928 w1937]
                    tunnel: w1905 -> [w1927 w1933]
                    tunnel: w1904 -> [w1926 w1936]
                    tunnel: [w1925 w1935] -> w1902
                    frame False {
                      n480 = Build Array(w1928, w1927, w1926) -> (w1925:u16[])
                    }
                    frame True {
                      w1929 = 100.0 ("y")
                      n481 = case shown="False" w1944 {
                        tunnel: w1934 -> [w1947 w1952]
                        tunnel: w1930 -> [w1948 w1951]
                        tunnel: [w1945 w1950] -> w1943
                        tunnel: [w1946 w1949] -> w1942
                        frame False {
                          n482 = local write "BTPR_avg_R"(w1948) -> ()
                          n483 = call "BRig_dataRT_stats__BTPR_avg_R.vi"() -> ("output_BTPR_avg_R__x100"=w1946:i32)  [unwired: 11 in]
                          n484 = local write "T2R_avg_R"(w1947) -> ()
                          n485 = call "BRig_dataRT_stats__T2R_avg_R.vi"() -> ("output_T2R_avg_R__x100"=w1945:i32)  [unwired: 11 in]
                        }
                        frame True {
                          n486 = call "BRig_dataRT_stats__BTPR_avg_L.vi"() -> ("output_BTPR_avg_L__x100"=w1949:i32)  [unwired: 11 in]
                          n487 = local write "BTPR_avg_L"(w1951) -> ()
                          n488 = local write "T2R_avg_L"(w1952) -> ()
                          n489 = call "BRig_dataRT_stats__T2R_avg_L.vi"() -> ("output_T2R_avg_L__x100"=w1950:i32)  [unwired: 11 in]
                        }
                      }
                      n490 = Multiply(x=w1934, y=w1929) -> (x*y=w1931:dbl)
                      n491 = Multiply(x=w1930, y=w1929) -> (x*y=w1932:dbl)
                      n492 = To Unsigned Word Integer(number=w1931) -> (unsigned 16bit integer=w1938:u16)
                      n493 = To Unsigned Word Integer(number=w1932) -> (unsigned 16bit integer=w1939:u16)
                      n494 = To Unsigned Word Integer(number=w1942) -> (unsigned 16bit integer=w1940:u16)
                      n495 = To Unsigned Word Integer(number=w1943) -> (unsigned 16bit integer=w1941:u16)
                      n496 = Build Array(w1937, w1941, w1938, w1937, w1940, w1939, w1937, w1933, w1936) -> (w1935:u16[])
                    }
                  }
                  n497 = RT FIFO Write(0:w1903, 1:w1902, 3:w1901) -> ()  [unwired: 2 in, 4 out]
                  n498 = call "BRig_RT_comm_tcp_write_RTwrite__RunState_Trial_selResult.vi"("input_dataTrial"=w1914, "iReward_or_iError"=FALSE, "input_dataCurrent"=w1915) -> ("output_strCmd"=w1913:string)  [unwired: 8 in]
                }
                frame "SelectWrong" {
                  n499 = call "BRig_RT__Case_Exp__generic__incrementCountTilThreshold.vi"("input_dataCurrent"=w1959) -> ("output_dataCurrent"=w1957:u16[], "output_underThreshold"=w1958:bool)  [unwired: 9 in]
                  n500 = Select(t=w1961, s=w1958, f=myRIO_BRig_RT__Case_Exp_stateList."endTrial1" ("Enum")) -> (s? t:f=w1960:T2)
                }
                frame "SelectTimeout_pre" {
                  n501 = call "BRig_RT__Case_Exp__State_WrongOrTimeout_Pre__v4.vi"("input_dataCurrent"=w1992, "input_WorTO"=TRUE, "input_dataBlock"=w1990, "input_dataTrial"=w1987, "input_dataExp"=w1988) -> ("output_T2R"=w1982:bool, "output_T2R_or_BTPR"=w1974:u16, "output_dataCurrent"=w1985:u16[], "output_dataBlock"=w1989:u16[][], "output_dataTrial"=w1984:u16[][], "output_BTPRavg"=w1978:dbl, "output_T2Ravg"=w1979:dbl, "output_R(F)_or_L(T)"=w1980:bool, "output_haveNewAvg"=w1981:bool)  [unwired: 1 in, 1 out]
                  n502 = xnode "Read/Write Control"("FPGA VI Reference In"=w1968, "error in"=w1967, "SelectionState"=FALSE) -> ("error out"=w1969:errorcluster)  [unwired: 1 out]
                  n503 = case shown="False" w1982 {
                    tunnel: w1974 -> [w2024 w2026]
                    tunnel: [w2023 w2025] -> w1977
                    frame False {
                      n504 = call "BRig_dataRT_stats__BTPR_cur.vi"() -> ("output_BTPR_cur"=w2023:i32)  [unwired: 11 in]
                      n505 = local write "BTPR_block"(w2024) -> ()
                    }
                    frame True {
                      n506 = call "BRig_dataRT_stats__T2R_cur.vi"() -> ("output_T2R_cur"=w2025:i32)  [unwired: 11 in]
                      n507 = local write "T2R_block"(w2026) -> ()
                    }
                  }
                  n508 = To Unsigned Word Integer(number=w1977) -> (unsigned 16bit integer=w1975:u16)
                  n509 = case shown="True" w1981 {
                    tunnel: w1980 -> [_ w2014]
                    tunnel: w1979 -> [_ w2004]
                    tunnel: w1978 -> [_ w2000]
                    tunnel: u16 3 -> [w1998 w2007]
                    tunnel: w1975 -> [w1997 w2003]
                    tunnel: w1974 -> [w1996 w2006]
                    tunnel: [w1995 w2005] -> w1972
                    frame False {
                      n510 = Build Array(w1998, w1997, w1996) -> (w1995:u16[])
                    }
                    frame True {
                      w1999 = 100.0 ("y")
                      n511 = case shown="True" w2014 {
                        tunnel: w2004 -> [w2017 w2022]
                        tunnel: w2000 -> [w2018 w2021]
                        tunnel: [w2015 w2020] -> w2013
                        tunnel: [w2016 w2019] -> w2012
                        frame False {
                          n512 = local write "BTPR_avg_R"(w2018) -> ()
                          n513 = call "BRig_dataRT_stats__BTPR_avg_R.vi"() -> ("output_BTPR_avg_R__x100"=w2016:i32)  [unwired: 11 in]
                          n514 = local write "T2R_avg_R"(w2017) -> ()
                          n515 = call "BRig_dataRT_stats__T2R_avg_R.vi"() -> ("output_T2R_avg_R__x100"=w2015:i32)  [unwired: 11 in]
                        }
                        frame True {
                          n516 = call "BRig_dataRT_stats__BTPR_avg_L.vi"() -> ("output_BTPR_avg_L__x100"=w2019:i32)  [unwired: 11 in]
                          n517 = local write "BTPR_avg_L"(w2021) -> ()
                          n518 = local write "T2R_avg_L"(w2022) -> ()
                          n519 = call "BRig_dataRT_stats__T2R_avg_L.vi"() -> ("output_T2R_avg_L__x100"=w2020:i32)  [unwired: 11 in]
                        }
                      }
                      n520 = Multiply(x=w2004, y=w1999) -> (x*y=w2001:dbl)
                      n521 = Multiply(x=w2000, y=w1999) -> (x*y=w2002:dbl)
                      n522 = To Unsigned Word Integer(number=w2001) -> (unsigned 16bit integer=w2008:u16)
                      n523 = To Unsigned Word Integer(number=w2002) -> (unsigned 16bit integer=w2009:u16)
                      n524 = To Unsigned Word Integer(number=w2012) -> (unsigned 16bit integer=w2010:u16)
                      n525 = To Unsigned Word Integer(number=w2013) -> (unsigned 16bit integer=w2011:u16)
                      n526 = Build Array(w2007, w2011, w2008, w2007, w2010, w2009, w2007, w2003, w2006) -> (w2005:u16[])
                    }
                  }
                  n527 = local write "error out"(w1969) -> ()
                  n528 = RT FIFO Write(0:w1973, 1:w1972, 3:w1971) -> ()  [unwired: 2 in, 4 out]
                  n529 = call "BRig_RT_comm_tcp_write_RTwrite__RunState_Trial_selResult.vi"("input_dataTrial"=w1984, "iReward_or_iError"=FALSE, "input_dataCurrent"=w1985) -> ("output_strCmd"=w1983:string)  [unwired: 8 in]
                }
                frame "SelectTimeout" {
                  n530 = call "BRig_RT__Case_Exp__generic__incrementCountTilThreshold.vi"("input_dataCurrent"=w2029) -> ("output_dataCurrent"=w2028:u16[], "output_underThreshold"=w2027:bool)  [unwired: 9 in]
                  n531 = Select(t=w2031, s=w2027, f=myRIO_BRig_RT__Case_Exp_stateList."endTrial1" ("Enum")) -> (s? t:f=w2030:T2)
                }
                frame "endTrial1" {
                  n532 = call "BRig_RT_comm_tcp_write_RTwrite__RunState_Trial_end.vi"("input_dataCurrent"=w2044) -> ("output_strCmd"=w2043:string)  [unwired: 10 in]
                  n533 = call "BRig_RT__Case_Exp__State_endTrial__v2.vi"("input_dataBlock"=w2040, "input_timeStamp_start"=w2045, "input_dataTrial"=w2052, "input_dataCurrent"=w2044) -> ("output_BTPRavg"=w2037:dbl, "output_T2Ravg"=w2038:dbl, "output_dataTrial"=w2051:u16[][], "output_dataCurrent"=w2046:u16[], "output_R(F)_or_L(T)"=w2039:bool, "output_runTime"=→"T_ExpRun_min":dbl)  [unwired: 2 in]
                  n534 = xnode "Read/Write Control"("FPGA VI Reference In"=w2048, "error in"=w2047, "SelectionState"=FALSE) -> ("error out"=w2049:errorcluster)  [unwired: 1 out]
                  n535 = case shown="False" w2039 {
                    tunnel: w2038 -> [w2055 w2058]
                    tunnel: w2037 -> [w2056 w2057]
                    frame False {
                      n536 = local write "BTPR_avg_R"(w2056) -> ()
                      n537 = local write "T2R_avg_R"(w2055) -> ()
                    }
                    frame True {
                      n538 = local write "BTPR_avg_L"(w2057) -> ()
                      n539 = local write "T2R_avg_L"(w2058) -> ()
                    }
                  }
                  n540 = local write "error out"(w2049) -> ()
                }
                frame "endTrial2" {
                  n541 = case shown="True" w2068 {
                    tunnel: [w2076 _] -> w2069
                    tunnel: [w2075 w2078] -> w2064
                    tunnel: w2063 -> [w2073 w2086]
                    tunnel: w2062 -> [w2074 w2084]
                    tunnel: [w2074 w2083] -> w2061
                    tunnel: [w2073 w2085] -> w2060
                    tunnel: w2059 -> [_ w2077]
                    frame False {
                      # "Receive commands"
                      n542 = call "BRig_RT__Case_Exp__UploadClosedLoop__v3.vi"() -> ("all rows"=w2076:i64[][], "output_haveCmd"=w2075:bool)  [unwired: 10 in]
                    }
                    frame True {
                      # "Parse commands and update"
                      n543 = Array Size(array=w2077) -> (size(s)=w2082:i32[])
                      n544 = Index Array(array=w2082, index=0) -> (element=w2080:i32)
                      n545 = Not Equal To 0?(x=w2080) -> (x != 0?=w2079:bool)
                      n546 = case shown="False" w2079 {
                        selector: w2079 -> [w2090 w2092]
                        tunnel: w2086 -> [w2088 w2096]
                        tunnel: [w2088 w2095] -> w2085
                        tunnel: w2084 -> [w2087 w2094]
                        tunnel: [w2087 w2093] -> w2083
                        tunnel: [w2090 w2092] -> w2078
                        tunnel: w2077 -> [_ w2091]
                        frame False {
                          w2089 = TRUE ("input_setValues")
                          # "Update"
                          n547 = call "BRig_RT_panel_cue_v0,90.vi"("input_setValues"=w2089, "input_dataExp"=w2088) -> ()  [unwired: 9 in, 1 out]
                          n548 = call "BRig_RT_panel_ExpStruct_v0,96.vi"("input_setValues"=w2089, "input_dataExp"=w2088) -> ()  [unwired: 9 in, 1 out]
                          n549 = call "BRig_RT_panel_Laser1_v0,90.vi"("input_setValues"=w2089, "input_dataExp"=w2088, "input_dataLC"=w2087) -> ()  [unwired: 7 in, 2 out]
                          n550 = call "BRig_RT_panel_Laser2_v0,90.vi"("input_setValues"=w2089, "input_dataExp"=w2088, "input_dataLC"=w2087) -> ()  [unwired: 7 in, 2 out]
                        }
                        frame True {
                          # "Parse"
                          n551 = call "BRig_RT__Case_Exp__UploadClosedLoop__updateSettings.vi"("input_newSettings"=w2091, "input_dataLC"=w2094, "input_dataExp"=w2096) -> ("output_dataLC"=w2093:u16[], "output_dataExp"=w2095:u16[])  [unwired: 7 in]
                        }
                      }
                    }
                  }
                  n552 = Select(t=myRIO_BRig_RT__Case_Exp_stateList."endTrial2", s=w2064, f=myRIO_BRig_RT__Case_Exp_stateList."endTrial3" ("Enum")) -> (s? t:f=w2065:T2)
                }
                frame "endTrial3" {
                  n553 = call "BRig_RT__Case_Exp__endTrial_checkFreeReward.vi"("input_dataBlock"=w2098, "input_dataExp"=w2107, "input_dataTrial"=w2108, "input_dataCurrent"=w2109) -> ("output_state"=w2099:T2, "output_endBlock"=w2097:bool)  [unwired: 6 in]
                  n554 = local read "STOP_endTrial"() -> (w2106:bool)
                  n555 = local read "STOP_abort"() -> (w2105:bool)
                  n556 = local read "START"() -> (w2103:bool)
                  n557 = Not(x=w2103) -> (.not. x?=w2104:bool)
                  n558 = Compound Arithmetic op=OR(w2106, w2104, w2105, w2097) -> (w2102:bool)
                  n559 = Select(t=myRIO_BRig_RT__Case_Exp_stateList."saveData_dataBlock" ("Enum"), s=w2102, f=w2099) -> (s? t:f=w2100:T2)
                }
                frame "endBlock" {
                  # "Get latest\nlaserSwitch"
                  n560 = call "BRig_dataExp_Loop_c_ExpStruct.vi"() -> ("output_Loop_c_ExpStruct"=w2118:i32)  [unwired: 11 in]
                  n561 = call "BRig_dataExp_LaserSwitch.vi"() -> ("output_LaserSwitch"=w2113:i32)  [unwired: 11 in]
                  n562 = local read "START"() -> (w2137:bool)
                  n563 = local read "STOP_endBlock"() -> (w2133:bool)
                  n564 = local read "STOP_endTrial"() -> (w2135:bool)
                  n565 = local read "STOP_abort"() -> (w2134:bool)
                  n566 = Replace Array Subset(array=w2111, new element=u16 2 ("new element/subarray"), index=w2118) -> (w2116:u16[])
                  n567 = call "BRig_RT_panel_ExpStruct_v1,11.vi"("input_setValues"=FALSE, "input_dataExp"=w2116) -> ("output_dataExp"=w2115:u16[])  [unwired: 9 in]
                  n568 = Index Array(array=w2115, index=w2113) -> (element=w2112:u16)
                  n569 = Not(x=w2137) -> (.not. x?=w2136:bool)
                  n570 = Select(t=myRIO_BRig_RT__Case_Exp_stateList."commUpload_dataTrial" ("Enum"), s=w2123, f=myRIO_BRig_RT__Case_Exp_stateList."initBlock" ("Enum")) -> (s? t:f=w2120:T2)
                  n571 = Replace Array Subset(array=w2111, new element=w2112, index=w2113) -> (w2114:u16[])
                  n572 = Compound Arithmetic op=OR(w2136, w2133, w2135, w2134) -> (w2127:bool)
                  n573 = Select(t=myRIO_BRig_RT__Case_Exp_stateList."endExp" ("Enum"), s=w2127, f=w2120) -> (s? t:f=w2138:T2)
                  n574 = Select(t="<S,E>" ("string"), s=w2127, f="") -> (s? t:f=w2124:string)
                }
                frame "endExp" {
                  n575 = xnode "Read/Write Control"("FPGA VI Reference In"=w2141, "error in"=w2140, "A6_Act"=FALSE) -> ("error out"=w2142:errorcluster)  [unwired: 1 out]
                  n576 = local write "error out"(w2142) -> ()
                }
                frame "commUpload_dataTrial" {
                }
                frame "saveData_dataBlock" {
                  n577 = Increment(x=w2172) -> (x+1=w2170:u16)
                  n578 = Replace Array Subset(array=w2164, new element=u16 2 ("new element/subarray"), index=0) -> (w2158:u16[])
                  n579 = Index Array(array=w2156, index (row)=0) -> (element=w2159:u16[])  [unwired: 1 in]
                  n580 = for {
                    tunnel: w2159 -> [w2182] mode=indexing
                    shift-right: [w2181] -> w2157
                    shift-left: w2158 -> [w2185]
                    i -> [w2184]
                    n581 = Increment(x=w2184) -> (x+1=w2183:i32)
                    n582 = Replace Array Subset(array=w2185, new element=w2182, index=w2183) -> (w2181:u16[])
                  }
                  n583 = RT FIFO Write(0:w2167, 1:w2157, 3:w2166) -> (11:w2169:errorcluster)  [unwired: 2 in, 3 out]
                  n584 = Unbundle By Name(w2169) -> ("code"=w2168:i32)
                  n585 = Greater?(x=w2170, y=u16 3) -> (0:w2178:bool)
                  n586 = Equal To 0?(x=w2168) -> (x = 0?=w2165:bool)
                  n587 = Or(x=w2178, y=w2165) -> (x .or. y?=w2177:bool)
                  n588 = Select(t=myRIO_BRig_RT__Case_Exp_stateList."endBlock" ("Enum"), s=w2177, f=w2173) -> (s? t:f=w2171:T2)
                }
                frame "saveData_dataTrial" {
                  n589 = Increment(x=w2203) -> (x+1=w2202:u16)
                  n590 = Replace Array Subset(array=w2188, new element=u16 1 ("new element/subarray"), index=0) -> (w2192:u16[])
                  n591 = Index Array(array=w2187, index (row)=0) -> (element=w2193:u16[])  [unwired: 1 in]
                  n592 = for {
                    tunnel: w2193 -> [w2212] mode=indexing
                    shift-right: [w2211] -> w2191
                    shift-left: w2192 -> [w2215]
                    i -> [w2214]
                    n593 = Increment(x=w2214) -> (x+1=w2213:i32)
                    n594 = Replace Array Subset(array=w2215, new element=w2212, index=w2213) -> (w2211:u16[])
                  }
                  n595 = RT FIFO Write(0:w2190, 1:w2191, 3:w2189) -> (11:w2198:errorcluster)  [unwired: 2 in, 3 out]
                  n596 = Unbundle By Name(w2198) -> ("code"=w2197:i32)
                  n597 = Equal To 0?(x=w2197) -> (x = 0?=w2186:bool)
                  n598 = Greater?(x=w2202, y=u16 3) -> (0:w2200:bool)
                  n599 = Or(x=w2200, y=w2186) -> (x .or. y?=w2199:bool)
                  n600 = Select(t=myRIO_BRig_RT__Case_Exp_stateList."endTrial2" ("Enum"), s=w2199, f=w2204) -> (s? t:f=w2205:T2)
                }
                frame "dummyState" {
                  n601 = call "BRig_dataCurrent_iTrial.vi"() -> ("output_iTrial"=w2222:i32)  [unwired: 11 in]
                  n602 = Index Array(array=w2223, index=w2222) -> (element=w2221:u16)
                  n603 = Equal?(x=w2221, y=u16 1) -> (x = y?=w2219:bool)
                  n604 = Equal To 0?(x=w2230) -> (x = 0?=w2231:bool)
                  n605 = Select(t=u16 13, s=w2219, f=u16 15) -> (s? t:f=w2216:u16)
                  n606 = Select(t=w2216, s=w2231, f=w2230) -> (s? t:f=w2229:u16)
                  n607 = Decrement(x=w2229) -> (x-1=w2228:u16)
                  n608 = Equal To 0?(x=w2228) -> (x = 0?=w2227:bool)
                  n609 = Select(t=myRIO_BRig_RT__Case_Exp_stateList."initTrial" ("Enum"), s=w2227, f=w2225) -> (s? t:f=w2224:T2)
                }
                frame "dummyState_endBlock" {
                  n610 = call "BRig_dataCurrent_iTrial.vi"() -> ("output_iTrial"=w2246:i32)  [unwired: 11 in]
                  n611 = Index Array(array=w2240, index=w2246) -> (element=w2236:u16)
                  n612 = Equal?(x=w2236, y=u16 1) -> (x = y?=w2244:bool)
                  n613 = Equal To 0?(x=w2237) -> (x = 0?=w2248:bool)
                  n614 = Select(t=u16 1, s=w2244, f=u16 3) -> (s? t:f=w2241:u16)
                  n615 = Select(t=w2241, s=w2248, f=w2237) -> (s? t:f=w2247:u16)
                  n616 = Decrement(x=w2247) -> (x-1=w2238:u16)
                  n617 = Equal To 0?(x=w2238) -> (x = 0?=w2239:bool)
                  n618 = Select(t=myRIO_BRig_RT__Case_Exp_stateList."initBlock" ("Enum"), s=w2239, f=w2250) -> (s? t:f=w2249:T2)
                }
                frame "FreeReward_pre" {
                  w2286 = u16 0 ("new element/subarray")
                  # "Duration = MTrig duration"
                  # "Duration = Reward Time"
                  n619 = call "BRig_dataCurrent_FreeReward_c.vi"() -> ("output_FreeReward_c"=w2287:i32)  [unwired: 11 in]
                  n620 = call "BRig_dataCurrent_iSpout.vi"() -> ("output_iSpout"=w2284:i32)  [unwired: 11 in]
                  n621 = call "BRig_dataCurrent_c_generic.vi"() -> ("output_count_generic"=w2293:i32)  [unwired: 11 in]
                  n622 = call "BRig_dataCurrent_T_generic.vi"() -> ("output_T_generic"=w2292:i32)  [unwired: 11 in]
                  n623 = Index Array(array=w2285, index=w2284) -> (element=w2283:u16)
                  n624 = call "BRig_dataMTrig_Solenoid_T_L.vi"() -> ("output_Solenoid_T_L"=w2282:i32)  [unwired: 11 in]
                  n625 = call "BRig_dataMTrig_Solenoid_T_R.vi"() -> ("output_Solenoid_T_R"=w2281:i32)  [unwired: 11 in]
                  n626 = local read "FPGA_count2ms"() -> (w2263:dbl)
                  n627 = call "BRig_dataTrial_T_Reward.vi"() -> ("output_T_Reward"=w2288:i32)  [unwired: 11 in]
                  n628 = Equal To 0?(x=w2283) -> (x = 0?=w2265:bool)
                  n629 = Select(t=w2282, s=w2265, f=w2281) -> (s? t:f=w2279:i32)
                  n630 = Index Array(array=w2289, index (row)=0 ("disabled index (row)"), index (col)=w2288) -> ()  [unwired: 1 out]
                  n631 = Index Array(array=w2280, index=w2279) -> (element=w2276:u16)
                  n632 = Replace Array Subset(array=w2285, new element #1=w2286, index #1=w2287, new element #2=w2286, index #2=w2293, new element #3=w2276, index #3=w2292) -> (w2291:u16[])
                  n633 = To Double Precision Float(number=w2276) -> (double precision float=w2264:dbl)
                  n634 = Multiply(x=w2264, y=w2263) -> (x*y=w2277:dbl)
                  n635 = call "BRig_dataExp_FreeReward_c_L.vi"() -> ("output_FreeReward_c_L"=w2270:i32)  [unwired: 11 in]
                  n636 = call "BRig_dataExp_FreeReward_c_R.vi"() -> ("output_FreeReward_c_R"=w2271:i32)  [unwired: 11 in]
                  n637 = Round Toward +Infinity(x=w2277) -> (ceil(x): smallest int >= x=w2278:dbl)
                  n638 = Select(t=w2270, s=w2265, f=w2271) -> (s? t:f=w2267:i32)
                  n639 = To Unsigned Long Integer(number=w2278) -> (unsigned 32bit integer=w2273:u32)
                  n640 = xnode "Read/Write Control"("FPGA VI Reference In"=w2275, "error in"=w2274, "Solenoid_nTotal_L"=w2273, "Solenoid_nTotal_R"=w2273) -> ()  [unwired: 2 out]
                  n641 = Index Array(array=w2268, index=w2267) -> (element=w2266:u16)
                  n642 = Increment(x=w2266) -> (x+1=w2256:u16)
                  n643 = case shown="True" w2265 {
                    tunnel: w2256 -> [w2297 w2299]
                    tunnel: [w2296 w2298] -> w2258
                    frame True {
                      n644 = local write "FreeReward_c_L"(w2297) -> ()
                      n645 = call "BRig_dataRT_stats__FreeReward_c_L.vi"() -> ("output_FreeReward_c_L"=w2296:i32)  [unwired: 11 in]
                    }
                    frame False {
                      n646 = local write "FreeReward_c_R"(w2299) -> ()
                      n647 = call "BRig_dataRT_stats__FreeReward_c_R.vi"() -> ("output_FreeReward_c_R"=w2298:i32)  [unwired: 11 in]
                    }
                  }
                  n648 = To Unsigned Word Integer(number=w2258) -> (unsigned 16bit integer=w2257:u16)
                  n649 = Build Array(u16 3, w2257, w2256) -> (w2262:u16[])
                  n650 = Replace Array Subset(array=w2268, new element=w2256, index=w2267) -> (w2269:u16[])
                  n651 = RT FIFO Write(0:w2260, 1:w2262, 3:w2259) -> ()  [unwired: 2 in, 4 out]
                }
                frame "FreeReward" {
                  n652 = call "BRig_dataCurrent_iSpout.vi"() -> ("output_iSpout"=w2310:i32)  [unwired: 11 in]
                  n653 = call "BRig_dataCurrent_c_generic.vi"() -> ("output_count_generic"=w2304:i32)  [unwired: 11 in]
                  n654 = Index Array(array=w2311, index #1=w2310, index #2=w2304) -> (element #1=w2309:u16, element #2=w2303:u16)
                  n655 = Equal To 0?(x=w2309) -> (x = 0?=w2307:bool)
                  n656 = Equal To 0?(x=w2303) -> (x = 0?=w2302:bool)
                  n657 = Not(x=w2307) -> (.not. x?=w2308:bool)
                  n658 = call "BRig_RT__Case_Exp__generic__incrementCountTilThreshold.vi"("input_dataCurrent"=w2311) -> ("output_dataCurrent"=w2312:u16[], "output_underThreshold"=w2301:bool)  [unwired: 9 in]
                  n659 = Select(t=w2315, s=w2301, f=myRIO_BRig_RT__Case_Exp_stateList."FreeRewardPost_pre" ("Enum")) -> (s? t:f=w2313:T2)
                  n660 = And(x=w2301, y=w2302) -> (x .and. y?=w2300:bool)
                  n661 = And(x=w2300, y=w2307) -> (x .and. y?=w2305:bool)
                  n662 = And(x=w2300, y=w2308) -> (x .and. y?=w2306:bool)
                }
                frame "FreeRewardPost" {
                  n663 = call "BRig_RT__Case_Exp__generic__incrementCountTilThreshold.vi"("input_dataCurrent"=w2322) -> ("output_dataCurrent"=w2321:u16[], "output_underThreshold"=w2320:bool)  [unwired: 9 in]
                  n664 = Select(t=w2325, s=w2320, f=myRIO_BRig_RT__Case_Exp_stateList."initTrial" ("Enum")) -> (s? t:f=w2323:T2)
                }
                frame "FreeRewardPost_pre" {
                  n665 = call "BRig_dataExp_T_RewardPost.vi"() -> ("output_T_RewardPost"=w2335:i32)  [unwired: 11 in]
                  n666 = call "BRig_dataCurrent_c_generic.vi"() -> ("output_count_generic"=w2338:i32)  [unwired: 11 in]
                  n667 = call "BRig_dataCurrent_T_generic.vi"() -> ("output_T_generic"=w2337:i32)  [unwired: 11 in]
                  n668 = Index Array(array=w2332, index=w2335) -> (element=w2334:u16)
                  n669 = Replace Array Subset(array=w2333, new element #1=u16 0 ("new element/subarray"), index #1=w2338, new element #2=w2334, index #2=w2337) -> (w2331:u16[])
                }
              }
              n670 = call "BRig_RT_panel_manualTriggering_v0,90.vi"("input_dataMTrig"=w1308) -> ("output_Solenoid_R"=w1319:bool, "output_Solenoid_L"=w1318:bool, "output_dataMTrig"=w1351:u16[], "output_Audio_L"=w1350:bool, "output_Audio_R"=w1349:bool, "output_CueLed"=w1347:bool, "output_Laser_l1"=w1323:bool, "output_Laser_l2"=w1343:bool)  [unwired: 11 in]
              n671 = call "BRig_RT__Case_Exp__comm_tcp__data_other.vi"("input_strState"=w1311, "input_strAccum"=w1312, "input_error"=w1313, "input_hTCP"=w1314, "input_I_connected_TCP"=w1315) -> ("output_strAccum"=w1294:string, "output_error"=w1293:errorcluster, "output_hTCP"=w1295:refnum<k5>, "output_I_connect_TCP"=w1296:bool)  [unwired: 3 in]
              n672 = Or(x="STOP_abort", y=w1335) -> (x .or. y?=w1297:bool)
              n673 = Or(x=w1348, y=w1347) -> (x .or. y?=w1326:bool)
              n674 = local read "Laser1_LED"() -> (w1284:bool)
              n675 = local read "Laser2_LED"() -> (w1283:bool)
              n676 = Or(x=w1350, y=w1365) -> (x .or. y?=w1325:bool)
              n677 = Or(x=w1364, y=w1349) -> (x .or. y?=w1324:bool)
              n678 = Or(x=w1322, y=w1323) -> (x .or. y?=w1342:bool)
              n679 = Or(x=w1346, y=w1343) -> (x .or. y?=w1344:bool)
              n680 = call "BRig_RT__Case_Exp__recordLick.vi"("input_dataLick"=w1334, "input_lick__R"=w1328, "input_lick__L"=w1329, "input_lick"=w1330, "intput_state__trialStart"=w1288, "intput_state__trialEnd"=w1333, "input_dataCurrent"=w1332) -> ("output_dataLick"=w1327:u16[][], "output_dataCurrent"=w1331:u16[])  [unwired: 7 in]
              n681 = xnode "Read/Write Control"("FPGA VI Reference In"=w1363, "error in"=w1362, "L1Led_ON"=w1284, "L2Led_ON"=w1283, "Solenoid_trig_L"=w1317, "Solenoid_trig_R"=w1316, "A3_SL"=w1318, "A1_SR"=w1319, "LC_Event_l1"=w1341, "LC_Laser_l1"=w1342, "LC_Event_l2"=w1345, "LC_Laser_l2"=w1344, "CueLed_Event"=w1326, "audioTrigger_L"=w1325, "audioTrigger_R"=w1324) -> ("FPGA VI Reference Out"=w1369:refnum<k20>, "error out"=w1368:errorcluster, "fpga_laser1"=w1282:bool, "fpga_laser2"=w1281:bool, "fpga_solenoid_L"=w1280:bool, "fpga_solenoid_R"=w1279:bool, "AnaIn_0"=w1309:i16, "AnaIn_1"=w1310:i16)
              n682 = local write "Laser1"(w1282) -> ()
              n683 = local write "Laser2"(w1281) -> ()
              n684 = local write "Solenoid L"(w1280) -> ()
              n685 = local write "Solenoid R"(w1279) -> ()
              n686 = call "BRig_RT__Case_Exp__recordAnalogInput__PortC__fifo__1value.vi"("input_iOccurence"=w1339, "resetOccurrence"=w1338, "input_dataCurrent"=w1332, "input_iState_start"=w1288, "rt fifo"=w1287, "input_iState_end"=w1333, "input_fifo_error"=w1286, "input_AI1"=w1310, "input_AI0"=w1309) -> ("output_fifo_error"=w1292:errorcluster, "output_iOccurrence"=w1340:u16)  [unwired: 8 in, 1 out]
              n687 = call "BRig_RT_timeLoop_Exp__noStateLimit.vi"("input_error"=w1292, "input_Threshold_reset"="input_Threshold_reset", "input_Threshold"=w1354, "input_timestamp"=w1355, "input_state"=w1288) -> ("output_Threshold"=w1352:bool, "output_duration"=→"tLoop":dbl)  [unwired: 4 in, 1 out]
              "Threshold" <- w1352
              n688 = node-c288() -> ()  [unwired: 1 in, 1 out]
            }
            "stop_TimedLoop" <- w893
            n689 = while {
              tunnel: w837 -> [w961]
              tunnel: w836 -> [w960]
              shift-right: [w955] -> _
              shift-left: 0 ("element") -> [w956]
              shift-right: [w951] -> _
              shift-left: w842 -> [w957]
              tunnel: [w954] -> w839
              tunnel: [w953] -> w838
              tunnel: w835 -> [w950]
              tunnel: w834 -> [w949]
              tunnel: [w948] -> w833
              tunnel: [w947] -> w832
              shift-right: [w945] -> _
              shift-left: FALSE -> [w946]
              stop <- w944 stop-if-true
              # "timed out?"
              n690 = RT FIFO Read(0:w961, 3:w960) -> (8:w954:refnum<k33>, 9:w958:u16, 10:w965:bool, 11:w962:errorcluster)  [unwired: 2 in, 1 out]
              n691 = Unbundle By Name(w962) -> ("code"=w966:i32)
              n692 = Not(x=w965) -> (.not. x?=w964:bool)
              n693 = Equal To 0?(x=w966) -> (x = 0?=w963:bool)
              n694 = And(x=w963, y=w964) -> (x .and. y?=w959:bool)
              n695 = Select(t=w962, s=w963, f=w960) -> (s? t:f=w953:errorcluster)
              n696 = case shown="True" w959 {
                tunnel: w958 -> [_ w997]
                tunnel: w957 -> [w989 w999]
                tunnel: w956 -> [w988 w996]
                tunnel: [w989 w998] -> w951
                tunnel: [w988 w992] -> w955
                tunnel: [_ w990] -> w952
                frame False {
                }
                frame True {
                  n697 = Replace Array Subset(array=w999, new element=w997, index=w996) -> (w998:u16[])
                  n698 = Increment(x=w996) -> (x+1=w994:i32)
                  n699 = Less?(x=w996, y=7 ("dimension size")) -> (x < y?=w991:bool)
                  n700 = Select(t=w994, s=w991, f=0) -> (s? t:f=w992:i32)
                  n701 = Not(x=w991) -> (.not. x?=w990:bool)
                }
              }
              n702 = case shown="True" w952 {
                tunnel: w951 -> [_ w978]
                tunnel: w950 -> [w969 w977]
                tunnel: w949 -> [w968 w976]
                tunnel: [w969 w974] -> w948
                tunnel: [w968 w973] -> w947
                tunnel: w946 -> [w967 w971]
                tunnel: [w967 w970] -> w945
                frame False {
                }
                frame True {
                  n703 = for {
                    N: 8 -> [_]
                    tunnel: w978 -> [w985] mode=indexing
                    tunnel: w977 -> [w987]
                    tunnel: w976 -> [w986]
                    shift-right: [w980] -> w972
                    shift-left: FALSE -> [w984]
                    tunnel: [w983] -> w974
                    tunnel: [w982] -> w973
                    n704 = shared-variable-write(w987, w986, w985) -> (w983:refnum<k21>, w982:errorcluster, w981:bool)  [unwired: 1 in]
                    n705 = Or(x=w984, y=w981) -> (x .or. y?=w980:bool)
                  }
                  n706 = Or(x=w971, y=w972) -> (x .or. y?=w970:bool)
                }
              }
              n707 = local read "stop_TimedLoop"() -> (w944:bool)
            }
            n708 = while {
              shift-right: [w1070] -> _
              shift-left: 0 -> [w1059]
              tunnel: w890 -> [w1077]
              tunnel: w882 -> [w1079]
              shift-right: [w1066] -> _
              shift-left: 0 -> [w1061]
              shift-right: [w1071] -> _
              shift-left: w829 -> [w1078]
              shift-right: [w1067] -> _
              shift-left: w857 -> [w1080]
              shift-right: [w1074] -> w879
              shift-left: w851 -> [w1087]
              shift-right: [w1075] -> w873
              shift-left: w850 -> [w1081]
              tunnel: w854 -> [w1064]
              tunnel: w858 -> [w1063]
              shift-right: [w1052] -> _
              shift-left: w824 -> [w1058]
              shift-right: [w1051] -> _
              shift-left: 0 -> [w1057]
              tunnel: w827 -> [w1055]
              tunnel: w826 -> [w1056]
              tunnel: [w1050] -> w821
              tunnel: [w1049] -> w820
              stop <- w1088 stop-if-true
              # "nColumns dataBlock"
              # "nColumns dataTrial"
              # "buffer_dataTrial"
              # "buffer_dataBlock"
              # "buffer_dataTrial"
              # "buffer_dataBlock"
              n709 = local read "stop_TimedLoop"() -> (w1088:bool)
              n710 = Not Equal To 0?(x=w1061) -> (x != 0?=w1062:bool)
              n711 = Not Equal To 0?(x=w1057) -> (x != 0?=w1048:bool)
              n712 = case shown="True" w1062 {
                tunnel: w1080 -> [w1240 w1243]
                tunnel: w1061 -> [w1241 w1245]
                tunnel: w1079 -> [_ w1254]
                tunnel: [w1241 w1242] -> w1068
                tunnel: [w1240 w1243] -> w1069
                frame False {
                }
                frame True {
                  n713 = Array Subset(array=w1243, length (row)=w1245) -> (w1256:u16[][])  [unwired: 3 in]
                  n714 = call "BRig_dataBlock_iBlock.vi"() -> ("output_iBlock"=w1251:i32)  [unwired: 11 in]
                  n715 = Index Array(array=w1243, index (row)=0, index (col)=w1251) -> (element=w1250:u16)
                  n716 = To Double Precision Float(number=w1256) -> (double precision float=w1255:dbl[][])
                  n717 = Not Equal?(x=u16 1, y=w1250) -> (x != y?=w1248:bool)
                  n718 = call-poly <vilib>:"Write To Spreadsheet File.vi"("delimiter (\\t)"="," ("delimiter (\\t)"), "append to file? (new file:F)"=w1248, "2D data"=w1255, "file path (dialog if empty)"=w1254) -> ("new file path (Not A Path if cancelled)"=w1247:path)  [unwired: 4 in]
                  n719 = call <vilib>:"Is Path and Not Empty.vi"("path"=w1247) -> ("Is Path and Not Empty?"=w1246:bool)  [unwired: 4 in]
                  n720 = Select(t=0, s=w1246, f=w1245) -> (s? t:f=w1242:i32)
                }
              }
              n721 = case shown="True" w1048 {
                tunnel: w1058 -> [w1092 w1101]
                tunnel: w1057 -> [w1091 w1094]
                tunnel: [w1091 w1100] -> w1053
                tunnel: [w1092 w1101] -> w1054
                tunnel: w1056 -> [w1090 w1109]
                tunnel: w1055 -> [w1089 w1108]
                tunnel: [w1090 w1099] -> w1050
                tunnel: [w1089 w1098] -> w1049
                frame False {
                }
                frame True {
                  n722 = Decrement(x=w1094) -> (x-1=w1093:i32)
                  n723 = Multiply(x=w1093, y=2 ("index")) -> (x*y=w1095:i32)
                  n724 = Increment(x=w1095) -> (x+1=w1096:i32)
                  n725 = Index Array(array=w1101, index #1=w1095, index #2=w1096) -> (element #1=w1107:u16, element #2=w1103:u16)
                  n726 = shared-variable-write(w1109, w1108, w1107) -> (w1104:refnum<k21>, w1105:errorcluster, w1106:bool)  [unwired: 1 in]
                  n727 = case shown="False" w1106 {
                    selector: w1106 -> [_ w1118]
                    tunnel: w1105 -> [w1115 w1116]
                    tunnel: w1104 -> [w1114 w1117]
                    tunnel: w1103 -> [w1113 _]
                    tunnel: [w1112 w1118] -> w1102
                    tunnel: [w1111 w1117] -> w1099
                    tunnel: [w1110 w1116] -> w1098
                    frame False {
                      n728 = shared-variable-write(w1114, w1115, w1113) -> (w1111:refnum<k21>, w1110:errorcluster, w1112:bool)  [unwired: 1 in]
                    }
                    frame True {
                    }
                  }
                  n729 = Select(t=w1094, s=w1102, f=w1093) -> (s? t:f=w1100:i32)
                }
              }
              n730 = RT FIFO Read(0:w1087, 3:w1081) -> (8:w1074:refnum<k33>, 9:w1065:u16[], 10:w1085:bool, 11:w1082:errorcluster)  [unwired: 2 in, 1 out]
              n731 = Unbundle By Name(w1082) -> ("code"=w1086:i32)
              n732 = Not(x=w1085) -> (.not. x?=w1084:bool)
              n733 = Equal To 0?(x=w1086) -> (x = 0?=w1083:bool)
              n734 = And(x=w1083, y=w1084) -> (x .and. y?=w1076:bool)
              n735 = Select(t=w1082, s=w1083, f=w1081) -> (s? t:f=w1075:errorcluster)
              n736 = Not Equal To 0?(x=w1059) -> (x != 0?=w1060:bool)
              n737 = case shown="True" w1060 {
                tunnel: w1078 -> [w1223 w1226]
                tunnel: w1059 -> [w1224 w1228]
                tunnel: w1077 -> [_ w1237]
                tunnel: [w1224 w1225] -> w1072
                tunnel: [w1223 w1226] -> w1073
                frame False {
                }
                frame True {
                  n738 = Array Subset(array=w1226, length (row)=w1228) -> (w1239:u16[][])  [unwired: 3 in]
                  n739 = call "BRig_dataTrial_nTrial.vi"() -> ("output_nTrial"=w1234:i32)  [unwired: 11 in]
                  n740 = Index Array(array=w1226, index (row)=0, index (col)=w1234) -> (element=w1233:u16)
                  n741 = To Double Precision Float(number=w1239) -> (double precision float=w1238:dbl[][])
                  n742 = Not Equal?(x=u16 1, y=w1233) -> (x != y?=w1231:bool)
                  n743 = call-poly <vilib>:"Write To Spreadsheet File.vi"("delimiter (\\t)"="," ("delimiter (\\t)"), "append to file? (new file:F)"=w1231, "2D data"=w1238, "file path (dialog if empty)"=w1237) -> ("new file path (Not A Path if cancelled)"=w1230:path)  [unwired: 4 in]
                  n744 = call <vilib>:"Is Path and Not Empty.vi"("path"=w1230) -> ("Is Path and Not Empty?"=w1229:bool)  [unwired: 4 in]
                  n745 = Select(t=0, s=w1229, f=w1228) -> (s? t:f=w1225:i32)
                }
              }
              n746 = case shown="True" w1076 {
                tunnel: w1073 -> [w1125 w1145]
                tunnel: w1072 -> [w1124 w1143]
                tunnel: [w1125 w1144] -> w1071
                tunnel: [w1124 w1142] -> w1070
                tunnel: w1069 -> [w1123 w1141]
                tunnel: w1068 -> [w1122 w1139]
                tunnel: [w1123 w1140] -> w1067
                tunnel: [w1122 w1138] -> w1066
                tunnel: w1065 -> [_ w1146]
                tunnel: w1064 -> [_ w1137]
                tunnel: w1063 -> [_ w1136]
                tunnel: w1054 -> [w1120 w1129]
                tunnel: w1053 -> [w1119 w1128]
                tunnel: [w1120 w1127] -> w1052
                tunnel: [w1119 w1126] -> w1051
                frame False {
                  n747 = Wait (ms)(milliseconds to wait=u32 10) -> ()  [unwired: 1 out]
                }
                frame True {
                  n748 = Index Array(array=w1146, index=0) -> (element=w1130:u16)
                  n749 = Equal?(x=w1130, y=u16 1) -> (x = y?=w1131:bool)
                  n750 = Equal?(x=w1130, y=u16 2) -> (x = y?=w1133:bool)
                  n751 = Or(x=w1131, y=w1133) -> (x .or. y?=w1132:bool)
                  n752 = case shown="False" w1132 {
                    tunnel: w1146 -> [w1154 w1202]
                    tunnel: w1145 -> [w1158 w1195]
                    tunnel: [w1158 w1194] -> w1144
                    tunnel: w1143 -> [w1157 w1193]
                    tunnel: [w1157 w1192] -> w1142
                    tunnel: w1141 -> [w1156 w1199]
                    tunnel: [w1156 w1197] -> w1140
                    tunnel: w1139 -> [w1155 w1198]
                    tunnel: [w1155 w1196] -> w1138
                    tunnel: w1137 -> [_ w1201]
                    tunnel: w1136 -> [_ w1200]
                    tunnel: w1131 -> [_ w1191]
                    tunnel: w1130 -> [w1159 _]
                    tunnel: w1129 -> [w1151 w1190]
                    tunnel: w1128 -> [w1152 w1189]
                    tunnel: [w1150 w1190] -> w1127
                    tunnel: [w1149 w1189] -> w1126
                    frame False {
                      n753 = Equal?(x=w1159, y=u16 3) -> (x = y?=w1148:bool)
                      n754 = case shown="True" w1148 {
                        tunnel: w1154 -> [_ w1166]
                        tunnel: w1152 -> [w1160 w1165]
                        tunnel: w1151 -> [w1161 w1164]
                        tunnel: [w1161 w1163] -> w1150
                        tunnel: [w1160 w1162] -> w1149
                        frame False {
                        }
                        frame True {
                          w1173 = 3 ("y")
                          n755 = Array Size(array=w1166) -> (size(s)=w1167:i32)
                          n756 = To Double Precision Float(number=w1167) -> (double precision float=w1168:dbl)
                          n757 = To Double Precision Float(number=w1173) -> (double precision float=w1172:dbl)
                          n758 = Divide(x=w1168, y=w1172) -> (x/y=w1169:dbl)
                          n759 = Round Toward -Infinity(1:w1169) -> (0:w1170:dbl)
                          n760 = To Long Integer(number=w1170) -> (32bit integer=w1171:i32)
                          n761 = for {
                            N: w1171 -> [_]
                            tunnel: w1173 -> [w1188]
                            tunnel: w1166 -> [w1185]
                            shift-right: [w1174] -> w1162
                            shift-left: w1165 -> [w1180]
                            shift-right: [w1175] -> w1163
                            shift-left: w1164 -> [w1182]
                            i -> [w1187]
                            n762 = Multiply(x=2 ("index"), y=w1180) -> (x*y=w1179:i32)
                            n763 = Multiply(x=w1187, y=w1188) -> (x*y=w1186:i32)
                            n764 = Increment(x=w1186) -> (x+1=w1184:i32)
                            n765 = Increment(x=w1184) -> (x+1=w1183:i32)
                            n766 = Increment(x=w1180) -> (x+1=w1174:i32)
                            n767 = Index Array(array=w1185, index #1=w1184, index #2=w1183) -> (element #1=w1177:u16, element #2=w1176:u16)
                            n768 = Increment(x=w1179) -> (x+1=w1178:i32)
                            n769 = Replace Array Subset(array=w1182, new element #1=w1177, index #1=w1179, new element #2=w1176, index #2=w1178) -> (w1175:u16[])
                          }
                        }
                      }
                    }
                    frame True {
                      n770 = case shown="True" w1191 {
                        tunnel: w1202 -> [w1210 w1222]
                        tunnel: w1201 -> [w1208 _]
                        tunnel: w1200 -> [_ w1217]
                        tunnel: w1199 -> [w1212 w1216]
                        tunnel: w1198 -> [w1211 w1218]
                        tunnel: [w1212 w1215] -> w1197
                        tunnel: [w1211 w1214] -> w1196
                        tunnel: w1195 -> [w1207 w1219]
                        tunnel: [w1205 w1219] -> w1194
                        tunnel: w1193 -> [w1204 w1213]
                        tunnel: [w1203 w1213] -> w1192
                        frame True {
                          n771 = Array Subset(array=w1210, index=1, length=w1208) -> (w1206:u16[])
                          n772 = Increment(x=w1204) -> (x+1=w1203:i32)
                          n773 = Replace Array Subset(array=w1207, new element=w1206, index (row)=w1204) -> (w1205:u16[][])  [unwired: 1 in]
                        }
                        frame False {
                          n774 = Array Subset(array=w1222, index=1, length=w1217) -> (w1220:u16[])
                          n775 = Increment(x=w1218) -> (x+1=w1214:i32)
                          n776 = Replace Array Subset(array=w1216, new element=w1220, index (row)=w1218) -> (w1215:u16[][])  [unwired: 1 in]
                        }
                      }
                    }
                  }
                }
              }
            }
            n777 = node-c288(w942) -> ()  [unwired: 1 out]
            n778 = RT FIFO Delete(0:w879, 2:TRUE ("force destroy? (F)"), 3:w873) -> ()  [unwired: 1 out]
            n779 = RT FIFO Delete(0:w839, 2:TRUE ("force destroy? (F)"), 3:w838) -> ()  [unwired: 1 out]
            n780 = flat-sequence {
              tunnel: w913 -> [w1258]
              tunnel: w912 -> [w1261]
              tunnel: w911 -> [w1260]
              tunnel: w910 -> [w1259]
              tunnel: w909 -> [w1263]
              tunnel: w907 -> [_]
              tunnel: w830 -> [w1265]
              tunnel: w877 -> [w1264]
              tunnel: [w1257] -> w888
              tunnel: w873 -> [_]
              tunnel: w906 -> [w1276]
              tunnel: w905 -> [w1275]
              tunnel: w904 -> [w1274]
              tunnel: [w1273] -> w903
              tunnel: [w1272] -> w902
              tunnel: [w1267] -> w898
              tunnel: w888 -> [w1266]
              frame #0 {
                # "Store"
                n781 = call "BRig_RT__Case_Exp__storeData__endExp__v5__p1.vi"("input_dataCurrent"=w1259, "input_dataLC"=w1264, "input_dataExp"=w1265, "input_dataExp_end"=w1260, "input_dataLC_end"=w1261) -> ("output_True"=w1262:bool)  [unwired: 10 in]
                n782 = call "BRig_RT__Case_Exp__storeData__endExp__v5__p2.vi"("input_dataCurrent"=w1259, "input_dataLick"=w1263, "input_True"=w1262, "input_dataMTrig"=w1258) -> ("output_True"=w1257:bool)  [unwired: 11 in]
              }
              frame #1 {
                # "Send"
                n783 = local read "Data Set Prefix"() -> (w1268:string)
                n784 = call "BRig_RT_comm_webdav_upload_all__v3.vi"("input_I_connected_webdav"=w1274, "input_fileName_prefix"=w1268, "input_hSession"=w1275, "input_error"=w1276, "input_True"=w1266) -> ("output_hSession"=w1272:T4, "error out"=w1273:errorcluster, "output_nFilenames"=w1269:i32, "output_arrFilenames"=w1270:string[], "output_uploaded"=w1271:bool[], "output_strCmd"=w1267:string)  [unwired: 5 in]
                n785 = call "BRig_RT_comm_webdav_upload_all_warnUser.vi"("input_n"=w1269, "input_arrFilenames"=w1270, "input_arrUploaded"=w1271) -> ()  [unwired: 9 in]
              }
            }
            n786 = flat-sequence {
              tunnel: w922 -> [w1277]
              tunnel: [w1277] -> w908
              frame #0 {
                w1278 = FALSE ("START")
                n787 = local write "START"(w1278) -> ()
                n788 = local write "STOP_endTrial"(w1278) -> ()
                n789 = local write "STOP_endBlock"(w1278) -> ()
              }
            }
            n790 = xnode "Read/Write Control"("FPGA VI Reference In"=w939, "error in"=w908, "Counts_Reset"=TRUE, "audioTrigger_L"=w925, "audioFreq_L_kHz"=w923, "audioAmp_L"=w924, "audioTrigger_R"=w925, "audioFreq_R_kHz"=w923, "audioAmp_R"=w924, "A3_SL"=w925, "A1_SR"=w925, "A6_Act"=w925) -> ("FPGA VI Reference Out"=w938:refnum<k20>, "error out"=w907:errorcluster)
            n791 = call "BRig_RT__Case_Exp__comm_tcp__data_other.vi"("input_strState"=w898, "input_strAccum"="" ("f"), "input_error"=w899, "input_hTCP"=w900, "input_I_connected_TCP"=w901) -> ("output_error"=w894:errorcluster, "output_hTCP"=w895:refnum<k5>, "output_I_connect_TCP"=w896:bool)  [unwired: 3 in, 1 out]
          }
        }
        n792 = local read "STOP_abort"() -> (w328:bool)
      }
    }
  }
  n793 = flat-sequence {
    tunnel: w96 -> [w2353]
    tunnel: w95 -> [w2355]
    tunnel: w89 -> [w2354]
    tunnel: [w2354] -> w101
    tunnel: [w2353] -> w100
    tunnel: [w2352] -> w99
    tunnel: w74 -> [w2351]
    tunnel: [w2351] -> w98
    tunnel: w75 -> [w2350]
    tunnel: [w2350] -> w97
    tunnel: w82 -> [w2348]
    tunnel: w81 -> [w2347]
    tunnel: w80 -> [w2346]
    tunnel: w76 -> [w2349]
    tunnel: [w2349] -> w94
    tunnel: w93 -> [_]
    tunnel: [w2348] -> w88
    tunnel: [w2347] -> w87
    tunnel: [w2346] -> w86
    tunnel: w101 -> [w2375]
    tunnel: w100 -> [w2374]
    tunnel: w99 -> [w2373]
    tunnel: [w2372] -> _
    tunnel: w98 -> [w2371]
    tunnel: w97 -> [w2370]
    tunnel: w94 -> [w2369]
    tunnel: w88 -> [w2368]
    tunnel: w87 -> [w2367]
    tunnel: w86 -> [w2366]
    frame #0 {
      # "Stop FPGA\nSend QUIT to Host"
      n794 = case shown="True" w2354 {
        tunnel: w2353 -> [_ w2364]
        tunnel: w2355 -> [w2361 w2363]
        tunnel: [w2361 w2362] -> w2352
        frame False {
        }
        frame True {
          n795 = xnode "Read/Write Control"("FPGA VI Reference In"=w2364, "error in"=w2363, "FPGA_Stop"=TRUE) -> ("error out"=w2362:errorcluster)  [unwired: 1 out]
        }
      }
      n796 = case shown="True" w2348 {
        tunnel: w2347 -> [_ w2360]
        tunnel: w2346 -> [_ w2359]
        frame False {
        }
        frame True {
          w2356 = "<S,Q><S,Q><S,Q><S,Q>" ("input_packet")
          n797 = call "BRig_RT_comm_tcp_write_RTwrite.vi"("input_error"=w2359, "input_packet"=w2356, "input_hTCP"=w2360) -> ("output_error"=w2358:errorcluster, "output_hTCP"=w2357:refnum<k5>)  [unwired: 5 in, 2 out]
          n798 = call "BRig_RT_comm_tcp_write_RTwrite.vi"("input_error"=w2358, "input_packet"=w2356, "input_hTCP"=w2357) -> ()  [unwired: 5 in, 4 out]
        }
      }
    }
    frame #1 {
      # "Disconnect FPGA\nDisconnect comm webdav"
      n799 = case shown="True" w2375 {
        tunnel: w2373 -> [w2380 w2383]
        tunnel: w2374 -> [_ w2382]
        tunnel: [w2380 w2381] -> w2372
        frame False {
        }
        frame True {
          n800 = xnode "Close FPGA VI Reference"("FPGA VI Reference In"=w2382, "error in"=w2383) -> ("error out"=w2384:errorcluster)
          n801 = call <vilib>:"Reset myRIO.vi"("error in (no error)"=w2384) -> ("error out"=w2381:errorcluster)  [unwired: 10 in]
        }
      }
      n802 = case shown="True" w2368 {
        tunnel: w2367 -> [_ w2377]
        tunnel: w2366 -> [_ w2376]
        frame False {
        }
        frame True {
          n803 = TCP Close Connection(connection ID=w2377, error in (no error)=w2376) -> ()  [unwired: 1 in, 2 out]
        }
      }
      n804 = case shown="True" w2371 {
        tunnel: w2370 -> [_ w2379]
        tunnel: w2369 -> [_ w2378]
        frame False {
        }
        frame True {
          n805 = call <vilib>:"Close Session.vi"("session handle"=w2379, "error in (no error)"=w2378) -> ()  [unwired: 13 in, 1 out]
        }
      }
    }
  }
  n806 = Flush Stream(8:w1, 11:w2) -> (0:w3:errorcluster, 3:w4:refnum<k21>)  [unwired: 2 in, 1 out]
  n807 = Flush Stream(8:w13, 11:w14) -> (0:w15:errorcluster, 3:w16:refnum<k21>)  [unwired: 2 in, 1 out]
  n808 = Destroy Stream Endpoint(8:w3, 11:w4) -> ()  [unwired: 1 out]
  n809 = Destroy Stream Endpoint(8:w15, 11:w16) -> ()  [unwired: 1 out]
